vi "HP8753 Collect and Display Data_Modified_V3.vi"(4 "saved data comments":string, 5 "saver's name":string, 6 "saved data title":string, 7 "file name (read description)":path, 8 "error in (no error)":errorcluster, 9 "save to file":bool=TRUE, 10 "data type (6 : formatted data)":u16(ring)=6 items=["raw data array 1", "raw data array 2", "raw data array 3", "raw data array 4", "error-corrected data", "error-corrected trace memory", "formatted data", "formatted memory", "formatted data / memory", "formatted data - memory"], 11 "VISA session":refnum<visa-resource-name>="GPIB0::22::INSTR") -> (0 "error out":errorcluster, 1 "data values":cluster{"real / stim":dbl, "imag / resp":sgl}[](array[cluster])=[{"real / stim"=50000000.0, "imag / resp"=-3.4421387}, {"real / stim"=51531250.0, "imag / resp"=-3.4520264}, {"real / stim"=53062500.0, "imag / resp"=-3.460205}, {"real / stim"=54593750.0, "imag / resp"=-3.465454}, {"real / stim"=56125000.0, "imag / resp"=-3.4788818}, {"real / stim"=57656250.0, "imag / resp"=-3.4852295}, {"real / stim"=59187500.0, "imag / resp"=-3.4934082}, {"real / stim"=60718750.0, "imag / resp"=-3.501587}, {"real / stim"=62250000.0, "imag / resp"=-3.5073242}, {"real / stim"=63781250.0, "imag / resp"=-3.5158691}, {"real / stim"=65312500.0, "imag / resp"=-3.5167236}, {"real / stim"=66843750.0, "imag / resp"=-3.5233154}, {"real / stim"=68375000.0, "imag / resp"=-3.5305176}, {"real / stim"=69906250.0, "imag / resp"=-3.5341797}, {"real / stim"=71437500.0, "imag / resp"=-3.5355225}, {"real / stim"=72968750.0, "imag / resp"=-3.5379639}, {"real / stim"=74500000.0, "imag / resp"=-3.53833}, {"real / stim"=76031250.0, "imag / resp"=-3.5405273}, {"real / stim"=77562500.0, "imag / resp"=-3.539917}, {"real / stim"=79093750.0, "imag / resp"=-3.5395508}, {"real / stim"=80625000.0, "imag / resp"=-3.5390625}, {"real / stim"=82156250.0, "imag / resp"=-3.53833}, {"real / stim"=83687500.0, "imag / resp"=-3.536499}, {"real / stim"=85218750.0, "imag / resp"=-3.5343018}, {"real / stim"=86750000.0, "imag / resp"=-3.53479}, {"real / stim"=88281250.0, "imag / resp"=-3.5333252}, {"real / stim"=89812500.0, "imag / resp"=-3.5310059}, {"real / stim"=91343750.0, "imag / resp"=-3.5339355}, {"real / stim"=92875000.0, "imag / resp"=-3.5319824}, {"real / stim"=94406250.0, "imag / resp"=-3.53479}, {"real / stim"=95937500.0, "imag / resp"=-3.5344238}, {"real / stim"=97468750.0, "imag / resp"=-3.5341797}, {"real / stim"=99000000.0, "imag / resp"=-3.5372314}, {"real / stim"=100531250.0, "imag / resp"=-3.539917}, {"real / stim"=102062500.0, "imag / resp"=-3.5408936}, {"real / stim"=103593750.0, "imag / resp"=-3.5462646}, {"real / stim"=105125000.0, "imag / resp"=-3.548706}, {"real / stim"=106656250.0, "imag / resp"=-3.5534668}, {"real / stim"=108187500.0, "imag / resp"=-3.557495}, {"real / stim"=109718750.0, "imag / resp"=-3.5615234}, {"real / stim"=111250000.0, "imag / resp"=-3.567871}, {"real / stim"=112781250.0, "imag / resp"=-3.5754395}, {"real / stim"=114312500.0, "imag / resp"=-3.578125}, {"real / stim"=115843750.0, "imag / resp"=-3.586792}, {"real / stim"=117375000.0, "imag / resp"=-3.5878906}, {"real / stim"=118906250.0, "imag / resp"=-3.5941162}, {"real / stim"=120437500.0, "imag / resp"=-3.600708}, {"real / stim"=121968750.0, "imag / resp"=-3.6297607}, {"real / stim"=123500000.0, "imag / resp"=-3.6346436}, {"real / stim"=125031250.0, "imag / resp"=-3.637329}, {"real / stim"=126562500.0, "imag / resp"=-3.6402588}, {"real / stim"=128093750.0, "imag / resp"=-3.6430664}, {"real / stim"=129625000.0, "imag / resp"=-3.6451416}, {"real / stim"=131156250.0, "imag / resp"=-3.6461182}, {"real / stim"=132687500.0, "imag / resp"=-3.649414}, {"real / stim"=134218750.0, "imag / resp"=-3.6500244}, {"real / stim"=135750000.0, "imag / resp"=-3.650879}, {"real / stim"=137281250.0, "imag / resp"=-3.649414}, {"real / stim"=138812500.0, "imag / resp"=-3.6502686}, {"real / stim"=140343750.0, "imag / resp"=-3.6501465}, {"real / stim"=141875000.0, "imag / resp"=-3.6499023}, {"real / stim"=143406250.0, "imag / resp"=-3.6488037}, {"real / stim"=144937500.0, "imag / resp"=-3.6505127}, {"real / stim"=146468750.0, "imag / resp"=-3.645874}, {"real / stim"=148000000.0, "imag / resp"=-3.6451416}, {"real / stim"=149531250.0, "imag / resp"=-3.6470947}, {"real / stim"=151062500.0, "imag / resp"=-3.647583}, {"real / stim"=152593750.0, "imag / resp"=-3.647583}, {"real / stim"=154125000.0, "imag / resp"=-3.6468506}, {"real / stim"=155656250.0, "imag / resp"=-3.6461182}, {"real / stim"=157187500.0, "imag / resp"=-3.6483154}, {"real / stim"=158718750.0, "imag / resp"=-3.6479492}, {"real / stim"=160250000.0, "imag / resp"=-3.6478271}, {"real / stim"=161781250.0, "imag / resp"=-3.6495361}, {"real / stim"=163312500.0, "imag / resp"=-3.647461}, {"real / stim"=164843750.0, "imag / resp"=-3.6467285}, {"real / stim"=166375000.0, "imag / resp"=-3.6429443}, {"real / stim"=167906250.0, "imag / resp"=-3.6403809}, {"real / stim"=169437500.0, "imag / resp"=-3.6375732}, {"real / stim"=170968750.0, "imag / resp"=-3.6330566}, {"real / stim"=172500000.0, "imag / resp"=-3.628296}, {"real / stim"=174031250.0, "imag / resp"=-3.6224365}, {"real / stim"=175562500.0, "imag / resp"=-3.6166992}, {"real / stim"=177093750.0, "imag / resp"=-3.6138916}, {"real / stim"=178625000.0, "imag / resp"=-3.605713}, {"real / stim"=180156250.0, "imag / resp"=-3.6018066}, {"real / stim"=181687500.0, "imag / resp"=-3.5952148}, {"real / stim"=183218750.0, "imag / resp"=-3.5897217}, {"real / stim"=184750000.0, "imag / resp"=-3.588501}, {"real / stim"=186281250.0, "imag / resp"=-3.5822754}, {"real / stim"=187812500.0, "imag / resp"=-3.5819092}, {"real / stim"=189343750.0, "imag / resp"=-3.5794678}, {"real / stim"=190875000.0, "imag / resp"=-3.5766602}, {"real / stim"=192406250.0, "imag / resp"=-3.5737305}, {"real / stim"=193937500.0, "imag / resp"=-3.5733643}, {"real / stim"=195468750.0, "imag / resp"=-3.5751953}, {"real / stim"=197000000.0, "imag / resp"=-3.5737305}, {"real / stim"=198531250.0, "imag / resp"=-3.5755615}, {"real / stim"=200062500.0, "imag / resp"=-3.5767822}, {"real / stim"=201593750.0, "imag / resp"=-3.5800781}, {"real / stim"=203125000.0, "imag / resp"=-3.5819092}, {"real / stim"=204656250.0, "imag / resp"=-3.5917969}, {"real / stim"=206187500.0, "imag / resp"=-3.5958252}, {"real / stim"=207718750.0, "imag / resp"=-3.6035156}, {"real / stim"=209250000.0, "imag / resp"=-3.611084}, {"real / stim"=210781250.0, "imag / resp"=-3.6195068}, {"real / stim"=212312500.0, "imag / resp"=-3.6246338}, {"real / stim"=213843750.0, "imag / resp"=-3.6364746}, {"real / stim"=215375000.0, "imag / resp"=-3.6450195}, {"real / stim"=216906250.0, "imag / resp"=-3.6513672}, {"real / stim"=218437500.0, "imag / resp"=-3.6573486}, {"real / stim"=219968750.0, "imag / resp"=-3.664795}, {"real / stim"=221500000.0, "imag / resp"=-3.6678467}, {"real / stim"=223031250.0, "imag / resp"=-3.6729736}, {"real / stim"=224562500.0, "imag / resp"=-3.6712646}, {"real / stim"=226093750.0, "imag / resp"=-3.670288}, {"real / stim"=227625000.0, "imag / resp"=-3.666626}, {"real / stim"=229156250.0, "imag / resp"=-3.6635742}, {"real / stim"=230687500.0, "imag / resp"=-3.657837}, {"real / stim"=232218750.0, "imag / resp"=-3.6553955}, {"real / stim"=233750000.0, "imag / resp"=-3.6481934}, {"real / stim"=235281250.0, "imag / resp"=-3.6396484}, {"real / stim"=236812500.0, "imag / resp"=-3.631836}, {"real / stim"=238343750.0, "imag / resp"=-3.6229248}, {"real / stim"=239875000.0, "imag / resp"=-3.6166992}, {"real / stim"=241406250.0, "imag / resp"=-3.6079102}, {"real / stim"=242937500.0, "imag / resp"=-3.602295}, {"real / stim"=244468750.0, "imag / resp"=-3.5928955}, {"real / stim"=246000000.0, "imag / resp"=-3.5859375}, {"real / stim"=247531250.0, "imag / resp"=-3.579712}, {"real / stim"=249062500.0, "imag / resp"=-3.5720215}, {"real / stim"=250593750.0, "imag / resp"=-3.5701904}, {"real / stim"=252125000.0, "imag / resp"=-3.567871}, {"real / stim"=253656250.0, "imag / resp"=-3.564087}, {"real / stim"=255187500.0, "imag / resp"=-3.5595703}, {"real / stim"=256718750.0, "imag / resp"=-3.5560303}, {"real / stim"=258250000.0, "imag / resp"=-3.5516357}, {"real / stim"=259781250.0, "imag / resp"=-3.5488281}, {"real / stim"=261312500.0, "imag / resp"=-3.5445557}, {"real / stim"=262843750.0, "imag / resp"=-3.545288}, {"real / stim"=264375000.0, "imag / resp"=-3.541626}, {"real / stim"=265906250.0, "imag / resp"=-3.5411377}, {"real / stim"=267437500.0, "imag / resp"=-3.5386963}, {"real / stim"=268968750.0, "imag / resp"=-3.5327148}, {"real / stim"=270500000.0, "imag / resp"=-3.529541}, {"real / stim"=272031250.0, "imag / resp"=-3.5256348}, {"real / stim"=273562500.0, "imag / resp"=-3.5212402}, {"real / stim"=275093750.0, "imag / resp"=-3.5153809}, {"real / stim"=276625000.0, "imag / resp"=-3.5135498}, {"real / stim"=278156250.0, "imag / resp"=-3.5101318}, {"real / stim"=279687500.0, "imag / resp"=-3.5045166}, {"real / stim"=281218750.0, "imag / resp"=-3.50354}, {"real / stim"=282750000.0, "imag / resp"=-3.5014648}, {"real / stim"=284281250.0, "imag / resp"=-3.4952393}, {"real / stim"=285812500.0, "imag / resp"=-3.4960938}, {"real / stim"=287343750.0, "imag / resp"=-3.4942627}, {"real / stim"=288875000.0, "imag / resp"=-3.4920654}, {"real / stim"=290406250.0, "imag / resp"=-3.4903564}, {"real / stim"=291937500.0, "imag / resp"=-3.4906006}, {"real / stim"=293468750.0, "imag / resp"=-3.493042}, {"real / stim"=295000000.0, "imag / resp"=-3.4952393}, {"real / stim"=296531250.0, "imag / resp"=-3.496582}, {"real / stim"=298062500.0, "imag / resp"=-3.5}, {"real / stim"=299593750.0, "imag / resp"=-3.5042725}, {"real / stim"=301125000.0, "imag / resp"=-3.5093994}, {"real / stim"=302656250.0, "imag / resp"=-3.515503}, {"real / stim"=304187500.0, "imag / resp"=-3.5222168}, {"real / stim"=305718750.0, "imag / resp"=-3.5230713}, {"real / stim"=307250000.0, "imag / resp"=-3.5317383}, {"real / stim"=308781250.0, "imag / resp"=-3.5350342}, {"real / stim"=310312500.0, "imag / resp"=-3.5384521}, {"real / stim"=311843750.0, "imag / resp"=-3.5410156}, {"real / stim"=313375000.0, "imag / resp"=-3.5408936}, {"real / stim"=314906250.0, "imag / resp"=-3.5386963}, {"real / stim"=316437500.0, "imag / resp"=-3.536499}, {"real / stim"=317968750.0, "imag / resp"=-3.5317383}, {"real / stim"=319500000.0, "imag / resp"=-3.5231934}, {"real / stim"=321031250.0, "imag / resp"=-3.5150146}, {"real / stim"=322562500.0, "imag / resp"=-3.5029297}, {"real / stim"=324093750.0, "imag / resp"=-3.4937744}, {"real / stim"=325625000.0, "imag / resp"=-3.4818115}, {"real / stim"=327156250.0, "imag / resp"=-3.4685059}, {"real / stim"=328687500.0, "imag / resp"=-3.4542236}, {"real / stim"=330218750.0, "imag / resp"=-3.4396973}, {"real / stim"=331750000.0, "imag / resp"=-3.4239502}, {"real / stim"=333281250.0, "imag / resp"=-3.4139404}, {"real / stim"=334812500.0, "imag / resp"=-3.3981934}, {"real / stim"=336343750.0, "imag / resp"=-3.3891602}, {"real / stim"=337875000.0, "imag / resp"=-3.3780518}, {"real / stim"=339406250.0, "imag / resp"=-3.3676758}, {"real / stim"=340937500.0, "imag / resp"=-3.359253}, {"real / stim"=342468750.0, "imag / resp"=-3.348877}, {"real / stim"=344000000.0, "imag / resp"=-3.3426514}, {"real / stim"=345531250.0, "imag / resp"=-3.3361816}, {"real / stim"=347062500.0, "imag / resp"=-3.3267822}, {"real / stim"=348593750.0, "imag / resp"=-3.3200684}, {"real / stim"=350125000.0, "imag / resp"=-3.314209}, {"real / stim"=351656250.0, "imag / resp"=-3.3060303}, {"real / stim"=353187500.0, "imag / resp"=-3.2999268}, {"real / stim"=354718750.0, "imag / resp"=-3.2924805}, {"real / stim"=356250000.0, "imag / resp"=-3.2878418}, {"real / stim"=357781250.0, "imag / resp"=-3.2827148}, {"real / stim"=359312500.0, "imag / resp"=-3.2756348}, {"real / stim"=360843750.0, "imag / resp"=-3.268921}, {"real / stim"=362375000.0, "imag / resp"=-3.265747}, {"real / stim"=363906250.0, "imag / resp"=-3.2613525}, {"real / stim"=365437500.0, "imag / resp"=-3.2561035}, {"real / stim"=366968750.0, "imag / resp"=-3.248291}, {"real / stim"=368500000.0, "imag / resp"=-3.2403564}, {"real / stim"=370031250.0, "imag / resp"=-3.2387695}, {"real / stim"=371562500.0, "imag / resp"=-3.232544}, {"real / stim"=373093750.0, "imag / resp"=-3.2229004}, {"real / stim"=374625000.0, "imag / resp"=-3.2219238}, {"real / stim"=376156250.0, "imag / resp"=-3.213379}, {"real / stim"=377687500.0, "imag / resp"=-3.2088623}, {"real / stim"=379218750.0, "imag / resp"=-3.2069092}, {"real / stim"=380750000.0, "imag / resp"=-3.2022705}, {"real / stim"=382281250.0, "imag / resp"=-3.197998}, {"real / stim"=383812500.0, "imag / resp"=-3.1929932}, {"real / stim"=385343750.0, "imag / resp"=-3.1867676}, {"real / stim"=386875000.0, "imag / resp"=-3.1846924}, {"real / stim"=388406250.0, "imag / resp"=-3.182251}, {"real / stim"=389937500.0, "imag / resp"=-3.1723633}, {"real / stim"=391468750.0, "imag / resp"=-3.1693115}, {"real / stim"=393000000.0, "imag / resp"=-3.1618652}, {"real / stim"=394531250.0, "imag / resp"=-3.1582031}, {"real / stim"=396062500.0, "imag / resp"=-3.151123}, {"real / stim"=397593750.0, "imag / resp"=-3.1497803}, {"real / stim"=399125000.0, "imag / resp"=-3.1468506}, {"real / stim"=400656250.0, "imag / resp"=-3.142334}, {"real / stim"=402187500.0, "imag / resp"=-3.1401367}, {"real / stim"=403718750.0, "imag / resp"=-3.1350098}, {"real / stim"=405250000.0, "imag / resp"=-3.1322021}, {"real / stim"=406781250.0, "imag / resp"=-3.1287842}, {"real / stim"=408312500.0, "imag / resp"=-3.1269531}, {"real / stim"=409843750.0, "imag / resp"=-3.1207275}, {"real / stim"=411375000.0, "imag / resp"=-3.1124268}, {"real / stim"=412906250.0, "imag / resp"=-3.109253}, {"real / stim"=414437500.0, "imag / resp"=-3.1004639}, {"real / stim"=415968750.0, "imag / resp"=-3.0942383}, {"real / stim"=417500000.0, "imag / resp"=-3.086792}, {"real / stim"=419031250.0, "imag / resp"=-3.0787354}, {"real / stim"=420562500.0, "imag / resp"=-3.071289}, {"real / stim"=422093750.0, "imag / resp"=-3.0628662}, {"real / stim"=423625000.0, "imag / resp"=-3.060913}, {"real / stim"=425156250.0, "imag / resp"=-3.0493164}, {"real / stim"=426687500.0, "imag / resp"=-3.0463867}, {"real / stim"=428218750.0, "imag / resp"=-3.0390625}, {"real / stim"=429750000.0, "imag / resp"=-3.0340576}, {"real / stim"=431281250.0, "imag / resp"=-3.0281982}, {"real / stim"=432812500.0, "imag / resp"=-3.020752}, {"real / stim"=434343750.0, "imag / resp"=-3.0109863}, {"real / stim"=435875000.0, "imag / resp"=-3.0072021}, {"real / stim"=437406250.0, "imag / resp"=-3.0039062}, {"real / stim"=438937500.0, "imag / resp"=-2.9969482}, {"real / stim"=440468750.0, "imag / resp"=-2.994873}, {"real / stim"=442000000.0, "imag / resp"=-2.9940186}, {"real / stim"=443531250.0, "imag / resp"=-2.9868164}, {"real / stim"=445062500.0, "imag / resp"=-2.9829102}, {"real / stim"=446593750.0, "imag / resp"=-2.9801025}, {"real / stim"=448125000.0, "imag / resp"=-2.9782715}, {"real / stim"=449656250.0, "imag / resp"=-2.979248}, {"real / stim"=451187500.0, "imag / resp"=-2.9776611}, {"real / stim"=452718750.0, "imag / resp"=-2.9768066}, {"real / stim"=454250000.0, "imag / resp"=-2.97583}, {"real / stim"=455781250.0, "imag / resp"=-2.975586}, {"real / stim"=457312500.0, "imag / resp"=-2.9731445}, {"real / stim"=458843750.0, "imag / resp"=-2.9672852}, {"real / stim"=460375000.0, "imag / resp"=-2.963379}, {"real / stim"=461906250.0, "imag / resp"=-2.9614258}, {"real / stim"=463437500.0, "imag / resp"=-2.9541016}, {"real / stim"=464968750.0, "imag / resp"=-2.947998}, {"real / stim"=466500000.0, "imag / resp"=-2.939087}, {"real / stim"=468031250.0, "imag / resp"=-2.930664}, {"real / stim"=469562500.0, "imag / resp"=-2.9232178}, {"real / stim"=471093750.0, "imag / resp"=-2.9160156}, {"real / stim"=472625000.0, "imag / resp"=-2.9084473}, {"real / stim"=474156250.0, "imag / resp"=-2.8984375}, {"real / stim"=475687500.0, "imag / resp"=-2.8894043}, {"real / stim"=477218750.0, "imag / resp"=-2.8780518}, {"real / stim"=478750000.0, "imag / resp"=-2.87146}, {"real / stim"=480281250.0, "imag / resp"=-2.862915}, {"real / stim"=481812500.0, "imag / resp"=-2.8583984}, {"real / stim"=483343750.0, "imag / resp"=-2.8497314}, {"real / stim"=484875000.0, "imag / resp"=-2.8443604}, {"real / stim"=486406250.0, "imag / resp"=-2.8378906}, {"real / stim"=487937500.0, "imag / resp"=-2.833496}, {"real / stim"=489468750.0, "imag / resp"=-2.8250732}, {"real / stim"=491000000.0, "imag / resp"=-2.826416}, {"real / stim"=492531250.0, "imag / resp"=-2.8209229}, {"real / stim"=494062500.0, "imag / resp"=-2.8170166}, {"real / stim"=495593750.0, "imag / resp"=-2.8131104}, {"real / stim"=497125000.0, "imag / resp"=-2.8127441}, {"real / stim"=498656250.0, "imag / resp"=-2.8111572}, {"real / stim"=500187500.0, "imag / resp"=-2.8095703}, {"real / stim"=501718750.0, "imag / resp"=-2.8087158}, {"real / stim"=503250000.0, "imag / resp"=-2.8051758}, {"real / stim"=504781250.0, "imag / resp"=-2.800415}, {"real / stim"=506312500.0, "imag / resp"=-2.7983398}, {"real / stim"=507843750.0, "imag / resp"=-2.800537}, {"real / stim"=509375000.0, "imag / resp"=-2.7972412}, {"real / stim"=510906250.0, "imag / resp"=-2.7955322}, {"real / stim"=512437500.0, "imag / resp"=-2.7893066}, {"real / stim"=513968750.0, "imag / resp"=-2.789795}, {"real / stim"=515500000.0, "imag / resp"=-2.7834473}, {"real / stim"=517031250.0, "imag / resp"=-2.779541}, {"real / stim"=518562500.0, "imag / resp"=-2.7781982}, {"real / stim"=520093750.0, "imag / resp"=-2.775879}, {"real / stim"=521625000.0, "imag / resp"=-2.7729492}, {"real / stim"=523156250.0, "imag / resp"=-2.770874}, {"real / stim"=524687500.0, "imag / resp"=-2.7645264}, {"real / stim"=526218750.0, "imag / resp"=-2.7635498}, {"real / stim"=527750000.0, "imag / resp"=-2.7574463}, {"real / stim"=529281250.0, "imag / resp"=-2.7558594}, {"real / stim"=530812500.0, "imag / resp"=-2.7543945}, {"real / stim"=532343750.0, "imag / resp"=-2.7503662}, {"real / stim"=533875000.0, "imag / resp"=-2.7474365}, {"real / stim"=535406250.0, "imag / resp"=-2.7425537}, {"real / stim"=536937500.0, "imag / resp"=-2.7371826}, {"real / stim"=538468750.0, "imag / resp"=-2.7368164}, {"real / stim"=540000000.0, "imag / resp"=-2.7336426}, {"real / stim"=541531250.0, "imag / resp"=-2.7313232}, {"real / stim"=543062500.0, "imag / resp"=-2.72937}, {"real / stim"=544593750.0, "imag / resp"=-2.7286377}, {"real / stim"=546125000.0, "imag / resp"=-2.7264404}, {"real / stim"=547656250.0, "imag / resp"=-2.7231445}, {"real / stim"=549187500.0, "imag / resp"=-2.7215576}, {"real / stim"=550718750.0, "imag / resp"=-2.71875}, {"real / stim"=552250000.0, "imag / resp"=-2.7202148}, {"real / stim"=553781250.0, "imag / resp"=-2.7163086}, {"real / stim"=555312500.0, "imag / resp"=-2.7155762}, {"real / stim"=556843750.0, "imag / resp"=-2.7121582}, {"real / stim"=558375000.0, "imag / resp"=-2.709961}, {"real / stim"=559906250.0, "imag / resp"=-2.709961}, {"real / stim"=561437500.0, "imag / resp"=-2.7073975}, {"real / stim"=562968750.0, "imag / resp"=-2.7020264}, {"real / stim"=564500000.0, "imag / resp"=-2.701416}, {"real / stim"=566031250.0, "imag / resp"=-2.6993408}, {"real / stim"=567562500.0, "imag / resp"=-2.6949463}, {"real / stim"=569093750.0, "imag / resp"=-2.6939697}, {"real / stim"=570625000.0, "imag / resp"=-2.6903076}, {"real / stim"=572156250.0, "imag / resp"=-2.6895752}, {"real / stim"=573687500.0, "imag / resp"=-2.6875}, {"real / stim"=575218750.0, "imag / resp"=-2.684082}, {"real / stim"=576750000.0, "imag / resp"=-2.6843262}, {"real / stim"=578281250.0, "imag / resp"=-2.6846924}, {"real / stim"=579812500.0, "imag / resp"=-2.6829834}, {"real / stim"=581343750.0, "imag / resp"=-2.6826172}, {"real / stim"=582875000.0, "imag / resp"=-2.6817627}, {"real / stim"=584406250.0, "imag / resp"=-2.684082}, {"real / stim"=585937500.0, "imag / resp"=-2.6811523}, {"real / stim"=587468750.0, "imag / resp"=-2.683838}, {"real / stim"=589000000.0, "imag / resp"=-2.685669}, {"real / stim"=590531250.0, "imag / resp"=-2.6853027}, {"real / stim"=592062500.0, "imag / resp"=-2.6868896}, {"real / stim"=593593750.0, "imag / resp"=-2.6906738}, {"real / stim"=595125000.0, "imag / resp"=-2.6914062}, {"real / stim"=596656250.0, "imag / resp"=-2.6934814}, {"real / stim"=598187500.0, "imag / resp"=-2.6942139}, {"real / stim"=599718750.0, "imag / resp"=-2.6964111}, {"real / stim"=601250000.0, "imag / resp"=-2.7023926}, {"real / stim"=602781250.0, "imag / resp"=-2.7038574}, {"real / stim"=604312500.0, "imag / resp"=-2.7019043}, {"real / stim"=605843750.0, "imag / resp"=-2.7053223}, {"real / stim"=607375000.0, "imag / resp"=-2.7088623}, {"real / stim"=608906250.0, "imag / resp"=-2.7130127}, {"real / stim"=610437500.0, "imag / resp"=-2.713501}, {"real / stim"=611968750.0, "imag / resp"=-2.7181396}, {"real / stim"=613500000.0, "imag / resp"=-2.7231445}, {"real / stim"=615031250.0, "imag / resp"=-2.7226562}, {"real / stim"=616562500.0, "imag / resp"=-2.7263184}, {"real / stim"=618093750.0, "imag / resp"=-2.7285156}, {"real / stim"=619625000.0, "imag / resp"=-2.7320557}, {"real / stim"=621156250.0, "imag / resp"=-2.732788}, {"real / stim"=622687500.0, "imag / resp"=-2.7375488}, {"real / stim"=624218750.0, "imag / resp"=-2.7432861}, {"real / stim"=625750000.0, "imag / resp"=-2.7454834}, {"real / stim"=627281250.0, "imag / resp"=-2.7487793}, {"real / stim"=628812500.0, "imag / resp"=-2.7545166}, {"real / stim"=630343750.0, "imag / resp"=-2.7589111}, {"real / stim"=631875000.0, "imag / resp"=-2.7633057}, {"real / stim"=633406250.0, "imag / resp"=-2.7698975}, {"real / stim"=634937500.0, "imag / resp"=-2.7734375}, {"real / stim"=636468750.0, "imag / resp"=-2.7840576}, {"real / stim"=638000000.0, "imag / resp"=-2.7890625}, {"real / stim"=639531250.0, "imag / resp"=-2.7982178}, {"real / stim"=641062500.0, "imag / resp"=-2.8051758}, {"real / stim"=642593750.0, "imag / resp"=-2.8135986}, {"real / stim"=644125000.0, "imag / resp"=-2.819336}, {"real / stim"=645656250.0, "imag / resp"=-2.8310547}, {"real / stim"=647187500.0, "imag / resp"=-2.8365479}, {"real / stim"=648718750.0, "imag / resp"=-2.850586}, {"real / stim"=650250000.0, "imag / resp"=-2.857544}, {"real / stim"=651781250.0, "imag / resp"=-2.866211}, {"real / stim"=653312500.0, "imag / resp"=-2.8760986}, {"real / stim"=654843750.0, "imag / resp"=-2.8884277}, {"real / stim"=656375000.0, "imag / resp"=-2.900879}, {"real / stim"=657906250.0, "imag / resp"=-2.9106445}, {"real / stim"=659437500.0, "imag / resp"=-2.9228516}, {"real / stim"=660968750.0, "imag / resp"=-2.9395752}, {"real / stim"=662500000.0, "imag / resp"=-2.951416}, {"real / stim"=664031250.0, "imag / resp"=-2.9677734}, {"real / stim"=665562500.0, "imag / resp"=-2.9816895}, {"real / stim"=667093750.0, "imag / resp"=-2.9985352}, {"real / stim"=668625000.0, "imag / resp"=-3.0142822}, {"real / stim"=670156250.0, "imag / resp"=-3.0336914}, {"real / stim"=671687500.0, "imag / resp"=-3.0532227}, {"real / stim"=673218750.0, "imag / resp"=-3.0703125}, {"real / stim"=674750000.0, "imag / resp"=-3.0942383}, {"real / stim"=676281250.0, "imag / resp"=-3.1136475}, {"real / stim"=677812500.0, "imag / resp"=-3.1384277}, {"real / stim"=679343750.0, "imag / resp"=-3.1657715}, {"real / stim"=680875000.0, "imag / resp"=-3.1912842}, {"real / stim"=682406250.0, "imag / resp"=-3.2218018}, {"real / stim"=683937500.0, "imag / resp"=-3.2485352}, {"real / stim"=685468750.0, "imag / resp"=-3.2784424}, {"real / stim"=687000000.0, "imag / resp"=-3.3138428}, {"real / stim"=688531250.0, "imag / resp"=-3.345337}, {"real / stim"=690062500.0, "imag / resp"=-3.3814697}, {"real / stim"=691593750.0, "imag / resp"=-3.418457}, {"real / stim"=693125000.0, "imag / resp"=-3.4538574}, {"real / stim"=694656250.0, "imag / resp"=-3.4940186}, {"real / stim"=696187500.0, "imag / resp"=-3.5374756}, {"real / stim"=697718750.0, "imag / resp"=-3.579834}, {"real / stim"=699250000.0, "imag / resp"=-3.619751}, {"real / stim"=700781250.0, "imag / resp"=-3.665039}, {"real / stim"=702312500.0, "imag / resp"=-3.7087402}, {"real / stim"=703843750.0, "imag / resp"=-3.7529297}, {"real / stim"=705375000.0, "imag / resp"=-3.796875}, {"real / stim"=706906250.0, "imag / resp"=-3.843872}, {"real / stim"=708437500.0, "imag / resp"=-3.8878174}, {"real / stim"=709968750.0, "imag / resp"=-3.928711}, {"real / stim"=711500000.0, "imag / resp"=-3.9735107}, {"real / stim"=713031250.0, "imag / resp"=-4.0117188}, {"real / stim"=714562500.0, "imag / resp"=-4.0495605}, {"real / stim"=716093750.0, "imag / resp"=-4.08667}, {"real / stim"=717625000.0, "imag / resp"=-4.1210938}, {"real / stim"=719156250.0, "imag / resp"=-4.150879}, {"real / stim"=720687500.0, "imag / resp"=-4.178955}, {"real / stim"=722218750.0, "imag / resp"=-4.2009277}, {"real / stim"=723750000.0, "imag / resp"=-4.220459}, {"real / stim"=725281250.0, "imag / resp"=-4.2370605}, {"real / stim"=726812500.0, "imag / resp"=-4.2470703}, {"real / stim"=728343750.0, "imag / resp"=-4.2509766}, {"real / stim"=729875000.0, "imag / resp"=-4.253174}, {"real / stim"=731406250.0, "imag / resp"=-4.2487793}, {"real / stim"=732937500.0, "imag / resp"=-4.238037}, {"real / stim"=734468750.0, "imag / resp"=-4.2250977}, {"real / stim"=736000000.0, "imag / resp"=-4.2106934}, {"real / stim"=737531250.0, "imag / resp"=-4.1884766}, {"real / stim"=739062500.0, "imag / resp"=-4.166748}, {"real / stim"=740593750.0, "imag / resp"=-4.147461}, {"real / stim"=742125000.0, "imag / resp"=-4.116455}, {"real / stim"=743656250.0, "imag / resp"=-4.0915527}, {"real / stim"=745187500.0, "imag / resp"=-4.065918}, {"real / stim"=746718750.0, "imag / resp"=-4.033203}, {"real / stim"=748250000.0, "imag / resp"=-4.0080566}, {"real / stim"=749781250.0, "imag / resp"=-3.9819336}, {"real / stim"=751312500.0, "imag / resp"=-3.9525146}, {"real / stim"=752843750.0, "imag / resp"=-3.9273682}, {"real / stim"=754375000.0, "imag / resp"=-3.9002686}, {"real / stim"=755906250.0, "imag / resp"=-3.8754883}, {"real / stim"=757437500.0, "imag / resp"=-3.8496094}, {"real / stim"=758968750.0, "imag / resp"=-3.8243408}, {"real / stim"=760500000.0, "imag / resp"=-3.8017578}, {"real / stim"=762031250.0, "imag / resp"=-3.7774658}, {"real / stim"=763562500.0, "imag / resp"=-3.7528076}, {"real / stim"=765093750.0, "imag / resp"=-3.7271729}, {"real / stim"=766625000.0, "imag / resp"=-3.7041016}, {"real / stim"=768156250.0, "imag / resp"=-3.6816406}, {"real / stim"=769687500.0, "imag / resp"=-3.659546}, {"real / stim"=771218750.0, "imag / resp"=-3.6368408}, {"real / stim"=772750000.0, "imag / resp"=-3.6119385}, {"real / stim"=774281250.0, "imag / resp"=-3.5906982}, {"real / stim"=775812500.0, "imag / resp"=-3.5682373}, {"real / stim"=777343750.0, "imag / resp"=-3.546997}, {"real / stim"=778875000.0, "imag / resp"=-3.5256348}, {"real / stim"=780406250.0, "imag / resp"=-3.5039062}, {"real / stim"=781937500.0, "imag / resp"=-3.4840088}, {"real / stim"=783468750.0, "imag / resp"=-3.4656982}, {"real / stim"=785000000.0, "imag / resp"=-3.4483643}, {"real / stim"=786531250.0, "imag / resp"=-3.432129}, {"real / stim"=788062500.0, "imag / resp"=-3.4139404}, {"real / stim"=789593750.0, "imag / resp"=-3.4006348}, {"real / stim"=791125000.0, "imag / resp"=-3.3862305}, {"real / stim"=792656250.0, "imag / resp"=-3.374878}, {"real / stim"=794187500.0, "imag / resp"=-3.362671}, {"real / stim"=795718750.0, "imag / resp"=-3.3515625}, {"real / stim"=797250000.0, "imag / resp"=-3.3410645}, {"real / stim"=798781250.0, "imag / resp"=-3.3305664}, {"real / stim"=800312500.0, "imag / resp"=-3.3204346}, {"real / stim"=801843750.0, "imag / resp"=-3.3148193}, {"real / stim"=803375000.0, "imag / resp"=-3.307495}, {"real / stim"=804906250.0, "imag / resp"=-3.3006592}, {"real / stim"=806437500.0, "imag / resp"=-3.293335}, {"real / stim"=807968750.0, "imag / resp"=-3.286499}, {"real / stim"=809500000.0, "imag / resp"=-3.2797852}, {"real / stim"=811031250.0, "imag / resp"=-3.2736816}, {"real / stim"=812562500.0, "imag / resp"=-3.2696533}, {"real / stim"=814093750.0, "imag / resp"=-3.2633057}, {"real / stim"=815625000.0, "imag / resp"=-3.255005}, {"real / stim"=817156250.0, "imag / resp"=-3.2507324}, {"real / stim"=818687500.0, "imag / resp"=-3.248291}, {"real / stim"=820218750.0, "imag / resp"=-3.241211}, {"real / stim"=821750000.0, "imag / resp"=-3.2398682}, {"real / stim"=823281250.0, "imag / resp"=-3.2357178}, {"real / stim"=824812500.0, "imag / resp"=-3.2305908}, {"real / stim"=826343750.0, "imag / resp"=-3.225708}, {"real / stim"=827875000.0, "imag / resp"=-3.2196045}, {"real / stim"=829406250.0, "imag / resp"=-3.2180176}, {"real / stim"=830937500.0, "imag / resp"=-3.2143555}, {"real / stim"=832468750.0, "imag / resp"=-3.208252}, {"real / stim"=834000000.0, "imag / resp"=-3.2075195}, {"real / stim"=835531250.0, "imag / resp"=-3.2010498}, {"real / stim"=837062500.0, "imag / resp"=-3.1973877}, {"real / stim"=838593750.0, "imag / resp"=-3.1965332}, {"real / stim"=840125000.0, "imag / resp"=-3.1904297}, {"real / stim"=841656250.0, "imag / resp"=-3.1870117}, {"real / stim"=843187500.0, "imag / resp"=-3.1846924}, {"real / stim"=844718750.0, "imag / resp"=-3.1813965}, {"real / stim"=846250000.0, "imag / resp"=-3.177246}, {"real / stim"=847781250.0, "imag / resp"=-3.1762695}, {"real / stim"=849312500.0, "imag / resp"=-3.1711426}, {"real / stim"=850843750.0, "imag / resp"=-3.1711426}, {"real / stim"=852375000.0, "imag / resp"=-3.168213}, {"real / stim"=853906250.0, "imag / resp"=-3.1643066}, {"real / stim"=855437500.0, "imag / resp"=-3.1606445}, {"real / stim"=856968750.0, "imag / resp"=-3.1583252}, {"real / stim"=858500000.0, "imag / resp"=-3.1530762}, {"real / stim"=860031250.0, "imag / resp"=-3.1481934}, {"real / stim"=861562500.0, "imag / resp"=-3.1428223}, {"real / stim"=863093750.0, "imag / resp"=-3.1376953}, {"real / stim"=864625000.0, "imag / resp"=-3.1367188}, {"real / stim"=866156250.0, "imag / resp"=-3.1328125}, {"real / stim"=867687500.0, "imag / resp"=-3.1315918}, {"real / stim"=869218750.0, "imag / resp"=-3.1312256}, {"real / stim"=870750000.0, "imag / resp"=-3.1274414}, {"real / stim"=872281250.0, "imag / resp"=-3.1226807}, {"real / stim"=873812500.0, "imag / resp"=-3.1237793}, {"real / stim"=875343750.0, "imag / resp"=-3.1235352}, {"real / stim"=876875000.0, "imag / resp"=-3.1228027}, {"real / stim"=878406250.0, "imag / resp"=-3.1208496}, {"real / stim"=879937500.0, "imag / resp"=-3.1206055}, {"real / stim"=881468750.0, "imag / resp"=-3.1218262}, {"real / stim"=883000000.0, "imag / resp"=-3.1241455}, {"real / stim"=884531250.0, "imag / resp"=-3.1257324}, {"real / stim"=886062500.0, "imag / resp"=-3.1291504}, {"real / stim"=887593750.0, "imag / resp"=-3.126709}, {"real / stim"=889125000.0, "imag / resp"=-3.1326904}, {"real / stim"=890656250.0, "imag / resp"=-3.1345215}, {"real / stim"=892187500.0, "imag / resp"=-3.1363525}, {"real / stim"=893718750.0, "imag / resp"=-3.142456}, {"real / stim"=895250000.0, "imag / resp"=-3.143921}, {"real / stim"=896781250.0, "imag / resp"=-3.1467285}, {"real / stim"=898312500.0, "imag / resp"=-3.151123}, {"real / stim"=899843750.0, "imag / resp"=-3.154419}, {"real / stim"=901375000.0, "imag / resp"=-3.1571045}, {"real / stim"=902906250.0, "imag / resp"=-3.1629639}, {"real / stim"=904437500.0, "imag / resp"=-3.1638184}, {"real / stim"=905968750.0, "imag / resp"=-3.168457}, {"real / stim"=907500000.0, "imag / resp"=-3.1716309}, {"real / stim"=909031250.0, "imag / resp"=-3.1750488}, {"real / stim"=910562500.0, "imag / resp"=-3.1816406}, {"real / stim"=912093750.0, "imag / resp"=-3.1827393}, {"real / stim"=913625000.0, "imag / resp"=-3.1862793}, {"real / stim"=915156250.0, "imag / resp"=-3.1881104}, {"real / stim"=916687500.0, "imag / resp"=-3.1901855}, {"real / stim"=918218750.0, "imag / resp"=-3.1948242}, {"real / stim"=919750000.0, "imag / resp"=-3.1934814}, {"real / stim"=921281250.0, "imag / resp"=-3.1986084}, {"real / stim"=922812500.0, "imag / resp"=-3.199829}, {"real / stim"=924343750.0, "imag / resp"=-3.2038574}, {"real / stim"=925875000.0, "imag / resp"=-3.2055664}, {"real / stim"=927406250.0, "imag / resp"=-3.206665}, {"real / stim"=928937500.0, "imag / resp"=-3.2087402}, {"real / stim"=930468750.0, "imag / resp"=-3.2126465}, {"real / stim"=932000000.0, "imag / resp"=-3.2144775}, {"real / stim"=933531250.0, "imag / resp"=-3.211792}, {"real / stim"=935062500.0, "imag / resp"=-3.2163086}, {"real / stim"=936593750.0, "imag / resp"=-3.2172852}, {"real / stim"=938125000.0, "imag / resp"=-3.2183838}, {"real / stim"=939656250.0, "imag / resp"=-3.2194824}, {"real / stim"=941187500.0, "imag / resp"=-3.2210693}, {"real / stim"=942718750.0, "imag / resp"=-3.2216797}, {"real / stim"=944250000.0, "imag / resp"=-3.2247314}, {"real / stim"=945781250.0, "imag / resp"=-3.2253418}, {"real / stim"=947312500.0, "imag / resp"=-3.2283936}, {"real / stim"=948843750.0, "imag / resp"=-3.2266846}, {"real / stim"=950375000.0, "imag / resp"=-3.2281494}, {"real / stim"=951906250.0, "imag / resp"=-3.227295}, {"real / stim"=953437500.0, "imag / resp"=-3.2299805}, {"real / stim"=954968750.0, "imag / resp"=-3.2301025}, {"real / stim"=956500000.0, "imag / resp"=-3.2319336}, {"real / stim"=958031250.0, "imag / resp"=-3.231079}, {"real / stim"=959562500.0, "imag / resp"=-3.229248}, {"real / stim"=961093750.0, "imag / resp"=-3.235962}, {"real / stim"=962625000.0, "imag / resp"=-3.2352295}, {"real / stim"=964156250.0, "imag / resp"=-3.2340088}, {"real / stim"=965687500.0, "imag / resp"=-3.2347412}, {"real / stim"=967218750.0, "imag / resp"=-3.237793}, {"real / stim"=968750000.0, "imag / resp"=-3.2388916}, {"real / stim"=970281250.0, "imag / resp"=-3.2403564}, {"real / stim"=971812500.0, "imag / resp"=-3.241455}, {"real / stim"=973343750.0, "imag / resp"=-3.2427979}, {"real / stim"=974875000.0, "imag / resp"=-3.2443848}, {"real / stim"=976406250.0, "imag / resp"=-3.244995}, {"real / stim"=977937500.0, "imag / resp"=-3.2458496}, {"real / stim"=979468750.0, "imag / resp"=-3.249878}, {"real / stim"=981000000.0, "imag / resp"=-3.2520752}, {"real / stim"=982531250.0, "imag / resp"=-3.2528076}, {"real / stim"=984062500.0, "imag / resp"=-3.2559814}, {"real / stim"=985593750.0, "imag / resp"=-3.26062}, {"real / stim"=987125000.0, "imag / resp"=-3.2652588}, {"real / stim"=988656250.0, "imag / resp"=-3.2664795}, {"real / stim"=990187500.0, "imag / resp"=-3.2722168}, {"real / stim"=991718750.0, "imag / resp"=-3.2752686}, {"real / stim"=993250000.0, "imag / resp"=-3.2823486}, {"real / stim"=994781250.0, "imag / resp"=-3.2877197}, {"real / stim"=996312500.0, "imag / resp"=-3.2929688}, {"real / stim"=997843750.0, "imag / resp"=-3.2956543}, {"real / stim"=999375000.0, "imag / resp"=-3.2980957}, {"real / stim"=1000906250.0, "imag / resp"=-3.30542}, {"real / stim"=1002437500.0, "imag / resp"=-3.3076172}, {"real / stim"=1003968750.0, "imag / resp"=-3.3115234}, {"real / stim"=1005500000.0, "imag / resp"=-3.3162842}, {"real / stim"=1007031250.0, "imag / resp"=-3.3223877}, {"real / stim"=1008562500.0, "imag / resp"=-3.326416}, {"real / stim"=1010093750.0, "imag / resp"=-3.3325195}, {"real / stim"=1011625000.0, "imag / resp"=-3.3370361}, {"real / stim"=1013156250.0, "imag / resp"=-3.3406982}, {"real / stim"=1014687500.0, "imag / resp"=-3.3479004}, {"real / stim"=1016218750.0, "imag / resp"=-3.3535156}, {"real / stim"=1017750000.0, "imag / resp"=-3.359253}, {"real / stim"=1019281250.0, "imag / resp"=-3.3649902}, {"real / stim"=1020812500.0, "imag / resp"=-3.3685303}, {"real / stim"=1022343750.0, "imag / resp"=-3.3742676}, {"real / stim"=1023875000.0, "imag / resp"=-3.3774414}, {"real / stim"=1025406250.0, "imag / resp"=-3.3811035}, {"real / stim"=1026937500.0, "imag / resp"=-3.388794}, {"real / stim"=1028468750.0, "imag / resp"=-3.3950195}, {"real / stim"=1030000000.0, "imag / resp"=-3.3966064}, {"real / stim"=1031531250.0, "imag / resp"=-3.401123}, {"real / stim"=1033062500.0, "imag / resp"=-3.4075928}, {"real / stim"=1034593750.0, "imag / resp"=-3.413086}, {"real / stim"=1036125000.0, "imag / resp"=-3.420044}, {"real / stim"=1037656250.0, "imag / resp"=-3.4213867}, {"real / stim"=1039187500.0, "imag / resp"=-3.4277344}, {"real / stim"=1040718750.0, "imag / resp"=-3.4311523}, {"real / stim"=1042250000.0, "imag / resp"=-3.434204}, {"real / stim"=1043781250.0, "imag / resp"=-3.4375}, {"real / stim"=1045312500.0, "imag / resp"=-3.4422607}, {"real / stim"=1046843750.0, "imag / resp"=-3.4468994}, {"real / stim"=1048375000.0, "imag / resp"=-3.4510498}, {"real / stim"=1049906250.0, "imag / resp"=-3.454956}, {"real / stim"=1051437500.0, "imag / resp"=-3.4575195}, {"real / stim"=1052968750.0, "imag / resp"=-3.46167}, {"real / stim"=1054500000.0, "imag / resp"=-3.4609375}, {"real / stim"=1056031250.0, "imag / resp"=-3.465088}, {"real / stim"=1057562500.0, "imag / resp"=-3.4649658}, {"real / stim"=1059093750.0, "imag / resp"=-3.468872}, {"real / stim"=1060625000.0, "imag / resp"=-3.472168}, {"real / stim"=1062156250.0, "imag / resp"=-3.4746094}, {"real / stim"=1063687500.0, "imag / resp"=-3.4770508}, {"real / stim"=1065218750.0, "imag / resp"=-3.473755}, {"real / stim"=1066750000.0, "imag / resp"=-3.4766846}, {"real / stim"=1068281250.0, "imag / resp"=-3.4798584}, {"real / stim"=1069812500.0, "imag / resp"=-3.481079}, {"real / stim"=1071343750.0, "imag / resp"=-3.4829102}, {"real / stim"=1072875000.0, "imag / resp"=-3.4838867}, {"real / stim"=1074406250.0, "imag / resp"=-3.4837646}, {"real / stim"=1075937500.0, "imag / resp"=-3.4854736}, {"real / stim"=1077468750.0, "imag / resp"=-3.4841309}, {"real / stim"=1079000000.0, "imag / resp"=-3.487915}, {"real / stim"=1080531250.0, "imag / resp"=-3.4907227}, {"real / stim"=1082062500.0, "imag / resp"=-3.4937744}, {"real / stim"=1083593750.0, "imag / resp"=-3.4938965}, {"real / stim"=1085125000.0, "imag / resp"=-3.498291}, {"real / stim"=1086656250.0, "imag / resp"=-3.5039062}, {"real / stim"=1088187500.0, "imag / resp"=-3.508667}, {"real / stim"=1089718750.0, "imag / resp"=-3.5117188}, {"real / stim"=1091250000.0, "imag / resp"=-3.5144043}, {"real / stim"=1092781250.0, "imag / resp"=-3.5184326}, {"real / stim"=1094312500.0, "imag / resp"=-3.5250244}, {"real / stim"=1095843750.0, "imag / resp"=-3.5289307}, {"real / stim"=1097375000.0, "imag / resp"=-3.536377}, {"real / stim"=1098906250.0, "imag / resp"=-3.5441895}, {"real / stim"=1100437500.0, "imag / resp"=-3.548706}, {"real / stim"=1101968750.0, "imag / resp"=-3.559082}, {"real / stim"=1103500000.0, "imag / resp"=-3.567749}, {"real / stim"=1105031250.0, "imag / resp"=-3.5739746}, {"real / stim"=1106562500.0, "imag / resp"=-3.5822754}, {"real / stim"=1108093750.0, "imag / resp"=-3.5888672}, {"real / stim"=1109625000.0, "imag / resp"=-3.6013184}, {"real / stim"=1111156250.0, "imag / resp"=-3.605835}, {"real / stim"=1112687500.0, "imag / resp"=-3.6142578}, {"real / stim"=1114218750.0, "imag / resp"=-3.6201172}, {"real / stim"=1115750000.0, "imag / resp"=-3.6317139}, {"real / stim"=1117281250.0, "imag / resp"=-3.6385498}, {"real / stim"=1118812500.0, "imag / resp"=-3.6501465}, {"real / stim"=1120343750.0, "imag / resp"=-3.6552734}, {"real / stim"=1121875000.0, "imag / resp"=-3.665039}, {"real / stim"=1123406250.0, "imag / resp"=-3.675293}, {"real / stim"=1124937500.0, "imag / resp"=-3.6831055}, {"real / stim"=1126468750.0, "imag / resp"=-3.692871}, {"real / stim"=1128000000.0, "imag / resp"=-3.7001953}, {"real / stim"=1129531250.0, "imag / resp"=-3.70813}, {"real / stim"=1131062500.0, "imag / resp"=-3.7164307}, {"real / stim"=1132593750.0, "imag / resp"=-3.7252197}, {"real / stim"=1134125000.0, "imag / resp"=-3.7302246}, {"real / stim"=1135656250.0, "imag / resp"=-3.741455}, {"real / stim"=1137187500.0, "imag / resp"=-3.7492676}, {"real / stim"=1138718750.0, "imag / resp"=-3.7556152}, {"real / stim"=1140250000.0, "imag / resp"=-3.7614746}, {"real / stim"=1141781250.0, "imag / resp"=-3.7717285}, {"real / stim"=1143312500.0, "imag / resp"=-3.777832}, {"real / stim"=1144843750.0, "imag / resp"=-3.7824707}, {"real / stim"=1146375000.0, "imag / resp"=-3.7896729}, {"real / stim"=1147906250.0, "imag / resp"=-3.7929688}, {"real / stim"=1149437500.0, "imag / resp"=-3.798706}, {"real / stim"=1150968750.0, "imag / resp"=-3.8051758}, {"real / stim"=1152500000.0, "imag / resp"=-3.8129883}, {"real / stim"=1154031250.0, "imag / resp"=-3.815796}, {"real / stim"=1155562500.0, "imag / resp"=-3.8222656}, {"real / stim"=1157093750.0, "imag / resp"=-3.8220215}, {"real / stim"=1158625000.0, "imag / resp"=-3.8272705}, {"real / stim"=1160156250.0, "imag / resp"=-3.831421}, {"real / stim"=1161687500.0, "imag / resp"=-3.8342285}, {"real / stim"=1163218750.0, "imag / resp"=-3.8389893}, {"real / stim"=1164750000.0, "imag / resp"=-3.8457031}, {"real / stim"=1166281250.0, "imag / resp"=-3.8481445}, {"real / stim"=1167812500.0, "imag / resp"=-3.85437}, {"real / stim"=1169343750.0, "imag / resp"=-3.8603516}, {"real / stim"=1170875000.0, "imag / resp"=-3.8613281}, {"real / stim"=1172406250.0, "imag / resp"=-3.8706055}, {"real / stim"=1173937500.0, "imag / resp"=-3.8745117}, {"real / stim"=1175468750.0, "imag / resp"=-3.8824463}, {"real / stim"=1177000000.0, "imag / resp"=-3.8867188}, {"real / stim"=1178531250.0, "imag / resp"=-3.8934326}, {"real / stim"=1180062500.0, "imag / resp"=-3.8989258}, {"real / stim"=1181593750.0, "imag / resp"=-3.907959}, {"real / stim"=1183125000.0, "imag / resp"=-3.9172363}, {"real / stim"=1184656250.0, "imag / resp"=-3.9246826}, {"real / stim"=1186187500.0, "imag / resp"=-3.9372559}, {"real / stim"=1187718750.0, "imag / resp"=-3.9468994}, {"real / stim"=1189250000.0, "imag / resp"=-3.9558105}, {"real / stim"=1190781250.0, "imag / resp"=-3.9692383}, {"real / stim"=1192312500.0, "imag / resp"=-3.980713}, {"real / stim"=1193843750.0, "imag / resp"=-3.9919434}, {"real / stim"=1195375000.0, "imag / resp"=-4.0058594}, {"real / stim"=1196906250.0, "imag / resp"=-4.0161133}, {"real / stim"=1198437500.0, "imag / resp"=-4.0334473}, {"real / stim"=1199968750.0, "imag / resp"=-4.0456543}, {"real / stim"=1201500000.0, "imag / resp"=-4.0634766}, {"real / stim"=1203031250.0, "imag / resp"=-4.074463}, {"real / stim"=1204562500.0, "imag / resp"=-4.0944824}, {"real / stim"=1206093750.0, "imag / resp"=-4.1105957}, {"real / stim"=1207625000.0, "imag / resp"=-4.1279297}, {"real / stim"=1209156250.0, "imag / resp"=-4.140625}, {"real / stim"=1210687500.0, "imag / resp"=-4.161377}, {"real / stim"=1212218750.0, "imag / resp"=-4.1726074}, {"real / stim"=1213750000.0, "imag / resp"=-4.1882324}, {"real / stim"=1215281250.0, "imag / resp"=-4.2109375}, {"real / stim"=1216812500.0, "imag / resp"=-4.2248535}, {"real / stim"=1218343750.0, "imag / resp"=-4.243164}, {"real / stim"=1219875000.0, "imag / resp"=-4.2612305}, {"real / stim"=1221406250.0, "imag / resp"=-4.279541}, {"real / stim"=1222937500.0, "imag / resp"=-4.2980957}, {"real / stim"=1224468750.0, "imag / resp"=-4.3137207}, {"real / stim"=1226000000.0, "imag / resp"=-4.335205}, {"real / stim"=1227531250.0, "imag / resp"=-4.352539}, {"real / stim"=1229062500.0, "imag / resp"=-4.371826}, {"real / stim"=1230593750.0, "imag / resp"=-4.3916016}, {"real / stim"=1232125000.0, "imag / resp"=-4.409912}, {"real / stim"=1233656250.0, "imag / resp"=-4.430664}, {"real / stim"=1235187500.0, "imag / resp"=-4.4519043}, {"real / stim"=1236718750.0, "imag / resp"=-4.468994}, {"real / stim"=1238250000.0, "imag / resp"=-4.4919434}, {"real / stim"=1239781250.0, "imag / resp"=-4.5097656}, {"real / stim"=1241312500.0, "imag / resp"=-4.5319824}, {"real / stim"=1242843750.0, "imag / resp"=-4.554199}, {"real / stim"=1244375000.0, "imag / resp"=-4.574951}, {"real / stim"=1245906250.0, "imag / resp"=-4.597168}, {"real / stim"=1247437500.0, "imag / resp"=-4.6186523}, {"real / stim"=1248968750.0, "imag / resp"=-4.6398926}, {"real / stim"=1250500000.0, "imag / resp"=-4.664795}, {"real / stim"=1252031250.0, "imag / resp"=-4.685791}, {"real / stim"=1253562500.0, "imag / resp"=-4.71167}, {"real / stim"=1255093750.0, "imag / resp"=-4.731201}, {"real / stim"=1256625000.0, "imag / resp"=-4.755127}, {"real / stim"=1258156250.0, "imag / resp"=-4.776367}, {"real / stim"=1259687500.0, "imag / resp"=-4.8032227}, {"real / stim"=1261218750.0, "imag / resp"=-4.8237305}, {"real / stim"=1262750000.0, "imag / resp"=-4.8500977}, {"real / stim"=1264281250.0, "imag / resp"=-4.878662}, {"real / stim"=1265812500.0, "imag / resp"=-4.898926}, {"real / stim"=1267343750.0, "imag / resp"=-4.9257812}, {"real / stim"=1268875000.0, "imag / resp"=-4.951172}, {"real / stim"=1270406250.0, "imag / resp"=-4.9797363}, {"real / stim"=1271937500.0, "imag / resp"=-5.005615}, {"real / stim"=1273468750.0, "imag / resp"=-5.0317383}, {"real / stim"=1275000000.0, "imag / resp"=-5.064209}, {"real / stim"=1276531250.0, "imag / resp"=-5.090088}, {"real / stim"=1278062500.0, "imag / resp"=-5.1208496}, {"real / stim"=1279593750.0, "imag / resp"=-5.1540527}, {"real / stim"=1281125000.0, "imag / resp"=-5.1853027}, {"real / stim"=1282656250.0, "imag / resp"=-5.2177734}, {"real / stim"=1284187500.0, "imag / resp"=-5.253662}, {"real / stim"=1285718750.0, "imag / resp"=-5.2856445}, {"real / stim"=1287250000.0, "imag / resp"=-5.32251}, {"real / stim"=1288781250.0, "imag / resp"=-5.362793}, {"real / stim"=1290312500.0, "imag / resp"=-5.3984375}, {"real / stim"=1291843750.0, "imag / resp"=-5.437744}, {"real / stim"=1293375000.0, "imag / resp"=-5.477783}, {"real / stim"=1294906250.0, "imag / resp"=-5.5166016}, {"real / stim"=1296437500.0, "imag / resp"=-5.5617676}, {"real / stim"=1297968750.0, "imag / resp"=-5.604248}, {"real / stim"=1299500000.0, "imag / resp"=-5.644287}, {"real / stim"=1301031250.0, "imag / resp"=-5.6896973}, {"real / stim"=1302562500.0, "imag / resp"=-5.734375}, {"real / stim"=1304093750.0, "imag / resp"=-5.779297}, {"real / stim"=1305625000.0, "imag / resp"=-5.8239746}, {"real / stim"=1307156250.0, "imag / resp"=-5.8720703}, {"real / stim"=1308687500.0, "imag / resp"=-5.9189453}, {"real / stim"=1310218750.0, "imag / resp"=-5.966797}, {"real / stim"=1311750000.0, "imag / resp"=-6.0129395}, {"real / stim"=1313281250.0, "imag / resp"=-6.0632324}, {"real / stim"=1314812500.0, "imag / resp"=-6.114258}, {"real / stim"=1316343750.0, "imag / resp"=-6.163086}, {"real / stim"=1317875000.0, "imag / resp"=-6.215576}, {"real / stim"=1319406250.0, "imag / resp"=-6.2651367}, {"real / stim"=1320937500.0, "imag / resp"=-6.315674}, {"real / stim"=1322468750.0, "imag / resp"=-6.369873}, {"real / stim"=1324000000.0, "imag / resp"=-6.419922}, {"real / stim"=1325531250.0, "imag / resp"=-6.472412}, {"real / stim"=1327062500.0, "imag / resp"=-6.524414}, {"real / stim"=1328593750.0, "imag / resp"=-6.581543}, {"real / stim"=1330125000.0, "imag / resp"=-6.6325684}, {"real / stim"=1331656250.0, "imag / resp"=-6.684082}, {"real / stim"=1333187500.0, "imag / resp"=-6.739746}, {"real / stim"=1334718750.0, "imag / resp"=-6.793213}, {"real / stim"=1336250000.0, "imag / resp"=-6.8481445}, {"real / stim"=1337781250.0, "imag / resp"=-6.9018555}, {"real / stim"=1339312500.0, "imag / resp"=-6.956787}, {"real / stim"=1340843750.0, "imag / resp"=-7.0131836}, {"real / stim"=1342375000.0, "imag / resp"=-7.071533}, {"real / stim"=1343906250.0, "imag / resp"=-7.1271973}, {"real / stim"=1345437500.0, "imag / resp"=-7.18042}, {"real / stim"=1346968750.0, "imag / resp"=-7.236084}, {"real / stim"=1348500000.0, "imag / resp"=-7.29126}, {"real / stim"=1350031250.0, "imag / resp"=-7.347412}, {"real / stim"=1351562500.0, "imag / resp"=-7.4016113}, {"real / stim"=1353093750.0, "imag / resp"=-7.4553223}, {"real / stim"=1354625000.0, "imag / resp"=-7.512207}, {"real / stim"=1356156250.0, "imag / resp"=-7.567627}, {"real / stim"=1357687500.0, "imag / resp"=-7.618408}, {"real / stim"=1359218750.0, "imag / resp"=-7.671875}, {"real / stim"=1360750000.0, "imag / resp"=-7.7282715}, {"real / stim"=1362281250.0, "imag / resp"=-7.783203}, {"real / stim"=1363812500.0, "imag / resp"=-7.8320312}, {"real / stim"=1365343750.0, "imag / resp"=-7.883789}, {"real / stim"=1366875000.0, "imag / resp"=-7.9401855}, {"real / stim"=1368406250.0, "imag / resp"=-7.9919434}, {"real / stim"=1369937500.0, "imag / resp"=-8.044434}, {"real / stim"=1371468750.0, "imag / resp"=-8.097168}, {"real / stim"=1373000000.0, "imag / resp"=-8.150391}, {"real / stim"=1374531250.0, "imag / resp"=-8.205566}, {"real / stim"=1376062500.0, "imag / resp"=-8.255371}, {"real / stim"=1377593750.0, "imag / resp"=-8.312988}, {"real / stim"=1379125000.0, "imag / resp"=-8.361816}, {"real / stim"=1380656250.0, "imag / resp"=-8.416504}, {"real / stim"=1382187500.0, "imag / resp"=-8.469238}, {"real / stim"=1383718750.0, "imag / resp"=-8.521973}, {"real / stim"=1385250000.0, "imag / resp"=-8.572754}, {"real / stim"=1386781250.0, "imag / resp"=-8.625977}, {"real / stim"=1388312500.0, "imag / resp"=-8.681152}, {"real / stim"=1389843750.0, "imag / resp"=-8.731445}, {"real / stim"=1391375000.0, "imag / resp"=-8.786133}, {"real / stim"=1392906250.0, "imag / resp"=-8.838379}, {"real / stim"=1394437500.0, "imag / resp"=-8.891113}, {"real / stim"=1395968750.0, "imag / resp"=-8.938477}, {"real / stim"=1397500000.0, "imag / resp"=-8.993164}, {"real / stim"=1399031250.0, "imag / resp"=-9.042969}, {"real / stim"=1400562500.0, "imag / resp"=-9.093262}, {"real / stim"=1402093750.0, "imag / resp"=-9.140137}, {"real / stim"=1403625000.0, "imag / resp"=-9.189453}, {"real / stim"=1405156250.0, "imag / resp"=-9.236328}, {"real / stim"=1406687500.0, "imag / resp"=-9.28125}, {"real / stim"=1408218750.0, "imag / resp"=-9.32666}, {"real / stim"=1409750000.0, "imag / resp"=-9.368652}, {"real / stim"=1411281250.0, "imag / resp"=-9.412109}, {"real / stim"=1412812500.0, "imag / resp"=-9.452637}, {"real / stim"=1414343750.0, "imag / resp"=-9.495605}, {"real / stim"=1415875000.0, "imag / resp"=-9.534668}, {"real / stim"=1417406250.0, "imag / resp"=-9.572754}, {"real / stim"=1418937500.0, "imag / resp"=-9.60791}, {"real / stim"=1420468750.0, "imag / resp"=-9.641113}, {"real / stim"=1422000000.0, "imag / resp"=-9.674316}, {"real / stim"=1423531250.0, "imag / resp"=-9.703613}, {"real / stim"=1425062500.0, "imag / resp"=-9.73291}, {"real / stim"=1426593750.0, "imag / resp"=-9.755859}, {"real / stim"=1428125000.0, "imag / resp"=-9.783203}, {"real / stim"=1429656250.0, "imag / resp"=-9.803711}, {"real / stim"=1431187500.0, "imag / resp"=-9.82373}, {"real / stim"=1432718750.0, "imag / resp"=-9.845215}, {"real / stim"=1434250000.0, "imag / resp"=-9.858887}, {"real / stim"=1435781250.0, "imag / resp"=-9.873535}, {"real / stim"=1437312500.0, "imag / resp"=-9.881836}, {"real / stim"=1438843750.0, "imag / resp"=-9.89209}, {"real / stim"=1440375000.0, "imag / resp"=-9.8984375}, {"real / stim"=1441906250.0, "imag / resp"=-9.901855}, {"real / stim"=1443437500.0, "imag / resp"=-9.908203}, {"real / stim"=1444968750.0, "imag / resp"=-9.912598}, {"real / stim"=1446500000.0, "imag / resp"=-9.907715}, {"real / stim"=1448031250.0, "imag / resp"=-9.904785}, {"real / stim"=1449562500.0, "imag / resp"=-9.901367}, {"real / stim"=1451093750.0, "imag / resp"=-9.893066}, {"real / stim"=1452625000.0, "imag / resp"=-9.888672}, {"real / stim"=1454156250.0, "imag / resp"=-9.878418}, {"real / stim"=1455687500.0, "imag / resp"=-9.87207}, {"real / stim"=1457218750.0, "imag / resp"=-9.85791}, {"real / stim"=1458750000.0, "imag / resp"=-9.84375}, {"real / stim"=1460281250.0, "imag / resp"=-9.830566}, {"real / stim"=1461812500.0, "imag / resp"=-9.816895}, {"real / stim"=1463343750.0, "imag / resp"=-9.800293}, {"real / stim"=1464875000.0, "imag / resp"=-9.783691}, {"real / stim"=1466406250.0, "imag / resp"=-9.765625}, {"real / stim"=1467937500.0, "imag / resp"=-9.745605}, {"real / stim"=1469468750.0, "imag / resp"=-9.728027}, {"real / stim"=1471000000.0, "imag / resp"=-9.705078}, {"real / stim"=1472531250.0, "imag / resp"=-9.689453}, {"real / stim"=1474062500.0, "imag / resp"=-9.6640625}, {"real / stim"=1475593750.0, "imag / resp"=-9.643555}, {"real / stim"=1477125000.0, "imag / resp"=-9.617676}, {"real / stim"=1478656250.0, "imag / resp"=-9.596191}, {"real / stim"=1480187500.0, "imag / resp"=-9.568359}, {"real / stim"=1481718750.0, "imag / resp"=-9.54541}, {"real / stim"=1483250000.0, "imag / resp"=-9.518555}, {"real / stim"=1484781250.0, "imag / resp"=-9.495605}, {"real / stim"=1486312500.0, "imag / resp"=-9.464355}, {"real / stim"=1487843750.0, "imag / resp"=-9.436035}, {"real / stim"=1489375000.0, "imag / resp"=-9.40918}, {"real / stim"=1490906250.0, "imag / resp"=-9.376953}, {"real / stim"=1492437500.0, "imag / resp"=-9.347656}, {"real / stim"=1493968750.0, "imag / resp"=-9.320801}, {"real / stim"=1495500000.0, "imag / resp"=-9.290039}, {"real / stim"=1497031250.0, "imag / resp"=-9.258301}, {"real / stim"=1498562500.0, "imag / resp"=-9.227051}, {"real / stim"=1500093750.0, "imag / resp"=-9.191895}, {"real / stim"=1501625000.0, "imag / resp"=-9.162598}, {"real / stim"=1503156250.0, "imag / resp"=-9.122559}, {"real / stim"=1504687500.0, "imag / resp"=-9.090332}, {"real / stim"=1506218750.0, "imag / resp"=-9.057617}, {"real / stim"=1507750000.0, "imag / resp"=-9.023926}, {"real / stim"=1509281250.0, "imag / resp"=-8.988281}, {"real / stim"=1510812500.0, "imag / resp"=-8.949219}, {"real / stim"=1512343750.0, "imag / resp"=-8.911133}, {"real / stim"=1513875000.0, "imag / resp"=-8.871582}, {"real / stim"=1515406250.0, "imag / resp"=-8.836426}, {"real / stim"=1516937500.0, "imag / resp"=-8.795898}, {"real / stim"=1518468750.0, "imag / resp"=-8.76123}, {"real / stim"=1520000000.0, "imag / resp"=-8.720703}, {"real / stim"=1521531250.0, "imag / resp"=-8.682129}, {"real / stim"=1523062500.0, "imag / resp"=-8.642578}, {"real / stim"=1524593750.0, "imag / resp"=-8.599609}, {"real / stim"=1526125000.0, "imag / resp"=-8.563965}, {"real / stim"=1527656250.0, "imag / resp"=-8.52002}, {"real / stim"=1529187500.0, "imag / resp"=-8.484863}, {"real / stim"=1530718750.0, "imag / resp"=-8.444336}, {"real / stim"=1532250000.0, "imag / resp"=-8.407227}, {"real / stim"=1533781250.0, "imag / resp"=-8.36377}, {"real / stim"=1535312500.0, "imag / resp"=-8.325684}, {"real / stim"=1536843750.0, "imag / resp"=-8.286621}, {"real / stim"=1538375000.0, "imag / resp"=-8.245117}, {"real / stim"=1539906250.0, "imag / resp"=-8.209473}, {"real / stim"=1541437500.0, "imag / resp"=-8.171387}, {"real / stim"=1542968750.0, "imag / resp"=-8.1328125}, {"real / stim"=1544500000.0, "imag / resp"=-8.097168}, {"real / stim"=1546031250.0, "imag / resp"=-8.054199}, {"real / stim"=1547562500.0, "imag / resp"=-8.021973}, {"real / stim"=1549093750.0, "imag / resp"=-7.9836426}, {"real / stim"=1550625000.0, "imag / resp"=-7.946289}, {"real / stim"=1552156250.0, "imag / resp"=-7.9089355}, {"real / stim"=1553687500.0, "imag / resp"=-7.875}, {"real / stim"=1555218750.0, "imag / resp"=-7.840332}, {"real / stim"=1556750000.0, "imag / resp"=-7.802246}, {"real / stim"=1558281250.0, "imag / resp"=-7.7678223}, {"real / stim"=1559812500.0, "imag / resp"=-7.7382812}, {"real / stim"=1561343750.0, "imag / resp"=-7.7036133}, {"real / stim"=1562875000.0, "imag / resp"=-7.6730957}, {"real / stim"=1564406250.0, "imag / resp"=-7.6428223}, {"real / stim"=1565937500.0, "imag / resp"=-7.6064453}, {"real / stim"=1567468750.0, "imag / resp"=-7.5751953}, {"real / stim"=1569000000.0, "imag / resp"=-7.5461426}, {"real / stim"=1570531250.0, "imag / resp"=-7.5148926}, {"real / stim"=1572062500.0, "imag / resp"=-7.4890137}, {"real / stim"=1573593750.0, "imag / resp"=-7.4560547}, {"real / stim"=1575125000.0, "imag / resp"=-7.429199}, {"real / stim"=1576656250.0, "imag / resp"=-7.404541}, {"real / stim"=1578187500.0, "imag / resp"=-7.3759766}, {"real / stim"=1579718750.0, "imag / resp"=-7.348877}, {"real / stim"=1581250000.0, "imag / resp"=-7.32251}, {"real / stim"=1582781250.0, "imag / resp"=-7.2963867}, {"real / stim"=1584312500.0, "imag / resp"=-7.270752}, {"real / stim"=1585843750.0, "imag / resp"=-7.240967}, {"real / stim"=1587375000.0, "imag / resp"=-7.2194824}, {"real / stim"=1588906250.0, "imag / resp"=-7.194092}, {"real / stim"=1590437500.0, "imag / resp"=-7.1679688}, {"real / stim"=1591968750.0, "imag / resp"=-7.1450195}, {"real / stim"=1593500000.0, "imag / resp"=-7.1191406}, {"real / stim"=1595031250.0, "imag / resp"=-7.095459}, {"real / stim"=1596562500.0, "imag / resp"=-7.072754}, {"real / stim"=1598093750.0, "imag / resp"=-7.046875}, {"real / stim"=1599625000.0, "imag / resp"=-7.0249023}, {"real / stim"=1601156250.0, "imag / resp"=-7.0046387}, {"real / stim"=1602687500.0, "imag / resp"=-6.9821777}, {"real / stim"=1604218750.0, "imag / resp"=-6.960449}, {"real / stim"=1605750000.0, "imag / resp"=-6.935791}, {"real / stim"=1607281250.0, "imag / resp"=-6.919922}, {"real / stim"=1608812500.0, "imag / resp"=-6.900879}, {"real / stim"=1610343750.0, "imag / resp"=-6.8776855}, {"real / stim"=1611875000.0, "imag / resp"=-6.8586426}, {"real / stim"=1613406250.0, "imag / resp"=-6.8359375}, {"real / stim"=1614937500.0, "imag / resp"=-6.819824}, {"real / stim"=1616468750.0, "imag / resp"=-6.8032227}, {"real / stim"=1618000000.0, "imag / resp"=-6.7802734}, {"real / stim"=1619531250.0, "imag / resp"=-6.7668457}, {"real / stim"=1621062500.0, "imag / resp"=-6.748047}, {"real / stim"=1622593750.0, "imag / resp"=-6.732666}, {"real / stim"=1624125000.0, "imag / resp"=-6.7141113}, {"real / stim"=1625656250.0, "imag / resp"=-6.7038574}, {"real / stim"=1627187500.0, "imag / resp"=-6.6862793}, {"real / stim"=1628718750.0, "imag / resp"=-6.6706543}, {"real / stim"=1630250000.0, "imag / resp"=-6.6621094}, {"real / stim"=1631781250.0, "imag / resp"=-6.647217}, {"real / stim"=1633312500.0, "imag / resp"=-6.640381}, {"real / stim"=1634843750.0, "imag / resp"=-6.625244}, {"real / stim"=1636375000.0, "imag / resp"=-6.618164}, {"real / stim"=1637906250.0, "imag / resp"=-6.6049805}, {"real / stim"=1639437500.0, "imag / resp"=-6.599121}, {"real / stim"=1640968750.0, "imag / resp"=-6.5895996}, {"real / stim"=1642500000.0, "imag / resp"=-6.578369}, {"real / stim"=1644031250.0, "imag / resp"=-6.5756836}, {"real / stim"=1645562500.0, "imag / resp"=-6.5668945}, {"real / stim"=1647093750.0, "imag / resp"=-6.5620117}, {"real / stim"=1648625000.0, "imag / resp"=-6.555908}, {"real / stim"=1650156250.0, "imag / resp"=-6.5498047}, {"real / stim"=1651687500.0, "imag / resp"=-6.546875}, {"real / stim"=1653218750.0, "imag / resp"=-6.5495605}, {"real / stim"=1654750000.0, "imag / resp"=-6.5458984}, {"real / stim"=1656281250.0, "imag / resp"=-6.5463867}, {"real / stim"=1657812500.0, "imag / resp"=-6.5495605}, {"real / stim"=1659343750.0, "imag / resp"=-6.5463867}, {"real / stim"=1660875000.0, "imag / resp"=-6.548828}, {"real / stim"=1662406250.0, "imag / resp"=-6.553467}, {"real / stim"=1663937500.0, "imag / resp"=-6.5583496}, {"real / stim"=1665468750.0, "imag / resp"=-6.562256}, {"real / stim"=1667000000.0, "imag / resp"=-6.5686035}, {"real / stim"=1668531250.0, "imag / resp"=-6.5754395}, {"real / stim"=1670062500.0, "imag / resp"=-6.581299}, {"real / stim"=1671593750.0, "imag / resp"=-6.5910645}, {"real / stim"=1673125000.0, "imag / resp"=-6.602295}, {"real / stim"=1674656250.0, "imag / resp"=-6.6118164}, {"real / stim"=1676187500.0, "imag / resp"=-6.6210938}, {"real / stim"=1677718750.0, "imag / resp"=-6.6330566}, {"real / stim"=1679250000.0, "imag / resp"=-6.644287}, {"real / stim"=1680781250.0, "imag / resp"=-6.6569824}, {"real / stim"=1682312500.0, "imag / resp"=-6.669922}, {"real / stim"=1683843750.0, "imag / resp"=-6.6845703}, {"real / stim"=1685375000.0, "imag / resp"=-6.7004395}, {"real / stim"=1686906250.0, "imag / resp"=-6.71167}, {"real / stim"=1688437500.0, "imag / resp"=-6.7263184}, {"real / stim"=1689968750.0, "imag / resp"=-6.7441406}, {"real / stim"=1691500000.0, "imag / resp"=-6.7595215}, {"real / stim"=1693031250.0, "imag / resp"=-6.7753906}, {"real / stim"=1694562500.0, "imag / resp"=-6.7929688}, {"real / stim"=1696093750.0, "imag / resp"=-6.809326}, {"real / stim"=1697625000.0, "imag / resp"=-6.824951}, {"real / stim"=1699156250.0, "imag / resp"=-6.840332}, {"real / stim"=1700687500.0, "imag / resp"=-6.86084}, {"real / stim"=1702218750.0, "imag / resp"=-6.876465}, {"real / stim"=1703750000.0, "imag / resp"=-6.894043}, {"real / stim"=1705281250.0, "imag / resp"=-6.911133}, {"real / stim"=1706812500.0, "imag / resp"=-6.925537}, {"real / stim"=1708343750.0, "imag / resp"=-6.942627}, {"real / stim"=1709875000.0, "imag / resp"=-6.960449}, {"real / stim"=1711406250.0, "imag / resp"=-6.979248}, {"real / stim"=1712937500.0, "imag / resp"=-6.99292}, {"real / stim"=1714468750.0, "imag / resp"=-7.0126953}, {"real / stim"=1716000000.0, "imag / resp"=-7.0319824}, {"real / stim"=1717531250.0, "imag / resp"=-7.04541}, {"real / stim"=1719062500.0, "imag / resp"=-7.0620117}, {"real / stim"=1720593750.0, "imag / resp"=-7.080078}, {"real / stim"=1722125000.0, "imag / resp"=-7.0930176}, {"real / stim"=1723656250.0, "imag / resp"=-7.1098633}, {"real / stim"=1725187500.0, "imag / resp"=-7.125244}, {"real / stim"=1726718750.0, "imag / resp"=-7.1401367}, {"real / stim"=1728250000.0, "imag / resp"=-7.1569824}, {"real / stim"=1729781250.0, "imag / resp"=-7.168213}, {"real / stim"=1731312500.0, "imag / resp"=-7.1831055}, {"real / stim"=1732843750.0, "imag / resp"=-7.191162}, {"real / stim"=1734375000.0, "imag / resp"=-7.20459}, {"real / stim"=1735906250.0, "imag / resp"=-7.2158203}, {"real / stim"=1737437500.0, "imag / resp"=-7.2226562}, {"real / stim"=1738968750.0, "imag / resp"=-7.2336426}, {"real / stim"=1740500000.0, "imag / resp"=-7.23999}, {"real / stim"=1742031250.0, "imag / resp"=-7.2470703}, {"real / stim"=1743562500.0, "imag / resp"=-7.253418}, {"real / stim"=1745093750.0, "imag / resp"=-7.2546387}, {"real / stim"=1746625000.0, "imag / resp"=-7.2578125}, {"real / stim"=1748156250.0, "imag / resp"=-7.259033}, {"real / stim"=1749687500.0, "imag / resp"=-7.2614746}, {"real / stim"=1751218750.0, "imag / resp"=-7.2597656}, {"real / stim"=1752750000.0, "imag / resp"=-7.2578125}, {"real / stim"=1754281250.0, "imag / resp"=-7.25708}, {"real / stim"=1755812500.0, "imag / resp"=-7.253174}, {"real / stim"=1757343750.0, "imag / resp"=-7.246582}, {"real / stim"=1758875000.0, "imag / resp"=-7.242676}, {"real / stim"=1760406250.0, "imag / resp"=-7.229248}, {"real / stim"=1761937500.0, "imag / resp"=-7.2231445}, {"real / stim"=1763468750.0, "imag / resp"=-7.209961}, {"real / stim"=1765000000.0, "imag / resp"=-7.19751}, {"real / stim"=1766531250.0, "imag / resp"=-7.184326}, {"real / stim"=1768062500.0, "imag / resp"=-7.1660156}, {"real / stim"=1769593750.0, "imag / resp"=-7.1516113}, {"real / stim"=1771125000.0, "imag / resp"=-7.133301}, {"real / stim"=1772656250.0, "imag / resp"=-7.1154785}, {"real / stim"=1774187500.0, "imag / resp"=-7.093506}, {"real / stim"=1775718750.0, "imag / resp"=-7.069092}, {"real / stim"=1777250000.0, "imag / resp"=-7.0476074}, {"real / stim"=1778781250.0, "imag / resp"=-7.023926}, {"real / stim"=1780312500.0, "imag / resp"=-6.999756}, {"real / stim"=1781843750.0, "imag / resp"=-6.970459}, {"real / stim"=1783375000.0, "imag / resp"=-6.947998}, {"real / stim"=1784906250.0, "imag / resp"=-6.914795}, {"real / stim"=1786437500.0, "imag / resp"=-6.887207}, {"real / stim"=1787968750.0, "imag / resp"=-6.854492}, {"real / stim"=1789500000.0, "imag / resp"=-6.821045}, {"real / stim"=1791031250.0, "imag / resp"=-6.7922363}, {"real / stim"=1792562500.0, "imag / resp"=-6.7612305}, {"real / stim"=1794093750.0, "imag / resp"=-6.727295}, {"real / stim"=1795625000.0, "imag / resp"=-6.688965}, {"real / stim"=1797156250.0, "imag / resp"=-6.6520996}, {"real / stim"=1798687500.0, "imag / resp"=-6.6169434}, {"real / stim"=1800218750.0, "imag / resp"=-6.5788574}, {"real / stim"=1801750000.0, "imag / resp"=-6.540039}, {"real / stim"=1803281250.0, "imag / resp"=-6.501709}, {"real / stim"=1804812500.0, "imag / resp"=-6.467285}, {"real / stim"=1806343750.0, "imag / resp"=-6.4333496}, {"real / stim"=1807875000.0, "imag / resp"=-6.3916016}, {"real / stim"=1809406250.0, "imag / resp"=-6.3535156}, {"real / stim"=1810937500.0, "imag / resp"=-6.3154297}, {"real / stim"=1812468750.0, "imag / resp"=-6.2785645}, {"real / stim"=1814000000.0, "imag / resp"=-6.238037}, {"real / stim"=1815531250.0, "imag / resp"=-6.199463}, {"real / stim"=1817062500.0, "imag / resp"=-6.159424}, {"real / stim"=1818593750.0, "imag / resp"=-6.1223145}, {"real / stim"=1820125000.0, "imag / resp"=-6.0844727}, {"real / stim"=1821656250.0, "imag / resp"=-6.0495605}, {"real / stim"=1823187500.0, "imag / resp"=-6.012207}, {"real / stim"=1824718750.0, "imag / resp"=-5.9750977}, {"real / stim"=1826250000.0, "imag / resp"=-5.940918}, {"real / stim"=1827781250.0, "imag / resp"=-5.9069824}, {"real / stim"=1829312500.0, "imag / resp"=-5.8669434}, {"real / stim"=1830843750.0, "imag / resp"=-5.8339844}, {"real / stim"=1832375000.0, "imag / resp"=-5.800537}, {"real / stim"=1833906250.0, "imag / resp"=-5.763916}, {"real / stim"=1835437500.0, "imag / resp"=-5.7319336}, {"real / stim"=1836968750.0, "imag / resp"=-5.696533}, {"real / stim"=1838500000.0, "imag / resp"=-5.6672363}, {"real / stim"=1840031250.0, "imag / resp"=-5.6342773}, {"real / stim"=1841562500.0, "imag / resp"=-5.598633}, {"real / stim"=1843093750.0, "imag / resp"=-5.569824}, {"real / stim"=1844625000.0, "imag / resp"=-5.5407715}, {"real / stim"=1846156250.0, "imag / resp"=-5.509033}, {"real / stim"=1847687500.0, "imag / resp"=-5.4726562}, {"real / stim"=1849218750.0, "imag / resp"=-5.445801}, {"real / stim"=1850750000.0, "imag / resp"=-5.41333}, {"real / stim"=1852281250.0, "imag / resp"=-5.3828125}, {"real / stim"=1853812500.0, "imag / resp"=-5.3566895}, {"real / stim"=1855343750.0, "imag / resp"=-5.3342285}, {"real / stim"=1856875000.0, "imag / resp"=-5.307129}, {"real / stim"=1858406250.0, "imag / resp"=-5.282959}, {"real / stim"=1859937500.0, "imag / resp"=-5.2578125}, {"real / stim"=1861468750.0, "imag / resp"=-5.230713}, {"real / stim"=1863000000.0, "imag / resp"=-5.206543}, {"real / stim"=1864531250.0, "imag / resp"=-5.182373}, {"real / stim"=1866062500.0, "imag / resp"=-5.165039}, {"real / stim"=1867593750.0, "imag / resp"=-5.1396484}, {"real / stim"=1869125000.0, "imag / resp"=-5.119385}, {"real / stim"=1870656250.0, "imag / resp"=-5.1013184}, {"real / stim"=1872187500.0, "imag / resp"=-5.08374}, {"real / stim"=1873718750.0, "imag / resp"=-5.0651855}, {"real / stim"=1875250000.0, "imag / resp"=-5.0480957}, {"real / stim"=1876781250.0, "imag / resp"=-5.0302734}, {"real / stim"=1878312500.0, "imag / resp"=-5.0144043}, {"real / stim"=1879843750.0, "imag / resp"=-4.9992676}, {"real / stim"=1881375000.0, "imag / resp"=-4.980713}, {"real / stim"=1882906250.0, "imag / resp"=-4.967041}, {"real / stim"=1884437500.0, "imag / resp"=-4.949463}, {"real / stim"=1885968750.0, "imag / resp"=-4.9313965}, {"real / stim"=1887500000.0, "imag / resp"=-4.916992}, {"real / stim"=1889031250.0, "imag / resp"=-4.9040527}, {"real / stim"=1890562500.0, "imag / resp"=-4.888672}, {"real / stim"=1892093750.0, "imag / resp"=-4.8710938}, {"real / stim"=1893625000.0, "imag / resp"=-4.8586426}, {"real / stim"=1895156250.0, "imag / resp"=-4.841797}, {"real / stim"=1896687500.0, "imag / resp"=-4.8291016}, {"real / stim"=1898218750.0, "imag / resp"=-4.811035}, {"real / stim"=1899750000.0, "imag / resp"=-4.79834}, {"real / stim"=1901281250.0, "imag / resp"=-4.7834473}, {"real / stim"=1902812500.0, "imag / resp"=-4.7666016}, {"real / stim"=1904343750.0, "imag / resp"=-4.7526855}, {"real / stim"=1905875000.0, "imag / resp"=-4.734619}, {"real / stim"=1907406250.0, "imag / resp"=-4.720459}, {"real / stim"=1908937500.0, "imag / resp"=-4.704834}, {"real / stim"=1910468750.0, "imag / resp"=-4.6875}, {"real / stim"=1912000000.0, "imag / resp"=-4.6708984}, {"real / stim"=1913531250.0, "imag / resp"=-4.6557617}, {"real / stim"=1915062500.0, "imag / resp"=-4.6379395}, {"real / stim"=1916593750.0, "imag / resp"=-4.625244}, {"real / stim"=1918125000.0, "imag / resp"=-4.607422}, {"real / stim"=1919656250.0, "imag / resp"=-4.593506}, {"real / stim"=1921187500.0, "imag / resp"=-4.5791016}, {"real / stim"=1922718750.0, "imag / resp"=-4.562256}, {"real / stim"=1924250000.0, "imag / resp"=-4.5461426}, {"real / stim"=1925781250.0, "imag / resp"=-4.5300293}, {"real / stim"=1927312500.0, "imag / resp"=-4.5166016}, {"real / stim"=1928843750.0, "imag / resp"=-4.5007324}, {"real / stim"=1930375000.0, "imag / resp"=-4.4838867}, {"real / stim"=1931906250.0, "imag / resp"=-4.468994}, {"real / stim"=1933437500.0, "imag / resp"=-4.4541016}, {"real / stim"=1934968750.0, "imag / resp"=-4.439453}, {"real / stim"=1936500000.0, "imag / resp"=-4.425293}, {"real / stim"=1938031250.0, "imag / resp"=-4.4106445}, {"real / stim"=1939562500.0, "imag / resp"=-4.395996}, {"real / stim"=1941093750.0, "imag / resp"=-4.3813477}, {"real / stim"=1942625000.0, "imag / resp"=-4.3657227}, {"real / stim"=1944156250.0, "imag / resp"=-4.3515625}, {"real / stim"=1945687500.0, "imag / resp"=-4.338135}, {"real / stim"=1947218750.0, "imag / resp"=-4.323242}, {"real / stim"=1948750000.0, "imag / resp"=-4.3112793}, {"real / stim"=1950281250.0, "imag / resp"=-4.29834}, {"real / stim"=1951812500.0, "imag / resp"=-4.2839355}, {"real / stim"=1953343750.0, "imag / resp"=-4.2702637}, {"real / stim"=1954875000.0, "imag / resp"=-4.2592773}, {"real / stim"=1956406250.0, "imag / resp"=-4.2487793}, {"real / stim"=1957937500.0, "imag / resp"=-4.2304688}, {"real / stim"=1959468750.0, "imag / resp"=-4.2211914}, {"real / stim"=1961000000.0, "imag / resp"=-4.213867}, {"real / stim"=1962531250.0, "imag / resp"=-4.202881}, {"real / stim"=1964062500.0, "imag / resp"=-4.1901855}, {"real / stim"=1965593750.0, "imag / resp"=-4.179199}, {"real / stim"=1967125000.0, "imag / resp"=-4.1711426}, {"real / stim"=1968656250.0, "imag / resp"=-4.165039}, {"real / stim"=1970187500.0, "imag / resp"=-4.152588}, {"real / stim"=1971718750.0, "imag / resp"=-4.147217}, {"real / stim"=1973250000.0, "imag / resp"=-4.135498}, {"real / stim"=1974781250.0, "imag / resp"=-4.1293945}, {"real / stim"=1976312500.0, "imag / resp"=-4.1228027}, {"real / stim"=1977843750.0, "imag / resp"=-4.119385}, {"real / stim"=1979375000.0, "imag / resp"=-4.107666}, {"real / stim"=1980906250.0, "imag / resp"=-4.105713}, {"real / stim"=1982437500.0, "imag / resp"=-4.0998535}, {"real / stim"=1983968750.0, "imag / resp"=-4.090576}, {"real / stim"=1985500000.0, "imag / resp"=-4.087158}, {"real / stim"=1987031250.0, "imag / resp"=-4.0776367}, {"real / stim"=1988562500.0, "imag / resp"=-4.072998}, {"real / stim"=1990093750.0, "imag / resp"=-4.0649414}, {"real / stim"=1991625000.0, "imag / resp"=-4.057129}, {"real / stim"=1993156250.0, "imag / resp"=-4.0549316}, {"real / stim"=1994687500.0, "imag / resp"=-4.0473633}, {"real / stim"=1996218750.0, "imag / resp"=-4.0405273}, {"real / stim"=1997750000.0, "imag / resp"=-4.0356445}, {"real / stim"=1999281250.0, "imag / resp"=-4.0273438}, {"real / stim"=2000812500.0, "imag / resp"=-4.017578}, {"real / stim"=2002343750.0, "imag / resp"=-4.015381}, {"real / stim"=2003875000.0, "imag / resp"=-4.0046387}, {"real / stim"=2005406250.0, "imag / resp"=-3.9997559}, {"real / stim"=2006937500.0, "imag / resp"=-3.9918213}, {"real / stim"=2008468750.0, "imag / resp"=-3.986206}, {"real / stim"=2010000000.0, "imag / resp"=-3.977539}, {"real / stim"=2011531250.0, "imag / resp"=-3.9718018}, {"real / stim"=2013062500.0, "imag / resp"=-3.9674072}, {"real / stim"=2014593750.0, "imag / resp"=-3.956421}, {"real / stim"=2016125000.0, "imag / resp"=-3.9472656}, {"real / stim"=2017656250.0, "imag / resp"=-3.9422607}, {"real / stim"=2019187500.0, "imag / resp"=-3.9353027}, {"real / stim"=2020718750.0, "imag / resp"=-3.928711}, {"real / stim"=2022250000.0, "imag / resp"=-3.9207764}, {"real / stim"=2023781250.0, "imag / resp"=-3.9140625}, {"real / stim"=2025312500.0, "imag / resp"=-3.9055176}, {"real / stim"=2026843750.0, "imag / resp"=-3.901123}, {"real / stim"=2028375000.0, "imag / resp"=-3.8945312}, {"real / stim"=2029906250.0, "imag / resp"=-3.883667}, {"real / stim"=2031437500.0, "imag / resp"=-3.8762207}, {"real / stim"=2032968750.0, "imag / resp"=-3.8707275}, {"real / stim"=2034500000.0, "imag / resp"=-3.859253}, {"real / stim"=2036031250.0, "imag / resp"=-3.8570557}, {"real / stim"=2037562500.0, "imag / resp"=-3.8464355}, {"real / stim"=2039093750.0, "imag / resp"=-3.842163}, {"real / stim"=2040625000.0, "imag / resp"=-3.8321533}, {"real / stim"=2042156250.0, "imag / resp"=-3.8220215}, {"real / stim"=2043687500.0, "imag / resp"=-3.817505}, {"real / stim"=2045218750.0, "imag / resp"=-3.8083496}, {"real / stim"=2046750000.0, "imag / resp"=-3.800293}, {"real / stim"=2048281250.0, "imag / resp"=-3.7906494}, {"real / stim"=2049812500.0, "imag / resp"=-3.7860107}, {"real / stim"=2051343750.0, "imag / resp"=-3.7747803}, {"real / stim"=2052875000.0, "imag / resp"=-3.7714844}, {"real / stim"=2054406250.0, "imag / resp"=-3.7598877}, {"real / stim"=2055937500.0, "imag / resp"=-3.7537842}, {"real / stim"=2057468750.0, "imag / resp"=-3.7456055}, {"real / stim"=2059000000.0, "imag / resp"=-3.73938}, {"real / stim"=2060531250.0, "imag / resp"=-3.7329102}, {"real / stim"=2062062500.0, "imag / resp"=-3.7261963}, {"real / stim"=2063593750.0, "imag / resp"=-3.720337}, {"real / stim"=2065125000.0, "imag / resp"=-3.7145996}, {"real / stim"=2066656250.0, "imag / resp"=-3.7052002}, {"real / stim"=2068187500.0, "imag / resp"=-3.7003174}, {"real / stim"=2069718750.0, "imag / resp"=-3.6976318}, {"real / stim"=2071250000.0, "imag / resp"=-3.690918}, {"real / stim"=2072781250.0, "imag / resp"=-3.6905518}, {"real / stim"=2074312500.0, "imag / resp"=-3.6849365}, {"real / stim"=2075843750.0, "imag / resp"=-3.6782227}, {"real / stim"=2077375000.0, "imag / resp"=-3.6779785}, {"real / stim"=2078906250.0, "imag / resp"=-3.6756592}, {"real / stim"=2080437500.0, "imag / resp"=-3.675415}, {"real / stim"=2081968750.0, "imag / resp"=-3.6711426}, {"real / stim"=2083500000.0, "imag / resp"=-3.6693115}, {"real / stim"=2085031250.0, "imag / resp"=-3.6711426}, {"real / stim"=2086562500.0, "imag / resp"=-3.6625977}, {"real / stim"=2088093750.0, "imag / resp"=-3.6627197}, {"real / stim"=2089625000.0, "imag / resp"=-3.6600342}, {"real / stim"=2091156250.0, "imag / resp"=-3.6610107}, {"real / stim"=2092687500.0, "imag / resp"=-3.6569824}, {"real / stim"=2094218750.0, "imag / resp"=-3.6514893}, {"real / stim"=2095750000.0, "imag / resp"=-3.6507568}, {"real / stim"=2097281250.0, "imag / resp"=-3.6450195}, {"real / stim"=2098812500.0, "imag / resp"=-3.6408691}, {"real / stim"=2100343750.0, "imag / resp"=-3.6403809}, {"real / stim"=2101875000.0, "imag / resp"=-3.635498}, {"real / stim"=2103406250.0, "imag / resp"=-3.6292725}, {"real / stim"=2104937500.0, "imag / resp"=-3.626709}, {"real / stim"=2106468750.0, "imag / resp"=-3.6254883}, {"real / stim"=2108000000.0, "imag / resp"=-3.6166992}, {"real / stim"=2109531250.0, "imag / resp"=-3.61438}, {"real / stim"=2111062500.0, "imag / resp"=-3.6088867}, {"real / stim"=2112593750.0, "imag / resp"=-3.6052246}, {"real / stim"=2114125000.0, "imag / resp"=-3.5979004}, {"real / stim"=2115656250.0, "imag / resp"=-3.5957031}, {"real / stim"=2117187500.0, "imag / resp"=-3.5909424}, {"real / stim"=2118718750.0, "imag / resp"=-3.5847168}, {"real / stim"=2120250000.0, "imag / resp"=-3.5855713}, {"real / stim"=2121781250.0, "imag / resp"=-3.5770264}, {"real / stim"=2123312500.0, "imag / resp"=-3.5761719}, {"real / stim"=2124843750.0, "imag / resp"=-3.5655518}, {"real / stim"=2126375000.0, "imag / resp"=-3.5601807}, {"real / stim"=2127906250.0, "imag / resp"=-3.5568848}, {"real / stim"=2129437500.0, "imag / resp"=-3.552124}, {"real / stim"=2130968750.0, "imag / resp"=-3.5465088}, {"real / stim"=2132500000.0, "imag / resp"=-3.543335}, {"real / stim"=2134031250.0, "imag / resp"=-3.5371094}, {"real / stim"=2135562500.0, "imag / resp"=-3.5236816}, {"real / stim"=2137093750.0, "imag / resp"=-3.5180664}, {"real / stim"=2138625000.0, "imag / resp"=-3.5124512}, {"real / stim"=2140156250.0, "imag / resp"=-3.508789}, {"real / stim"=2141687500.0, "imag / resp"=-3.5019531}, {"real / stim"=2143218750.0, "imag / resp"=-3.496582}, {"real / stim"=2144750000.0, "imag / resp"=-3.482544}, {"real / stim"=2146281250.0, "imag / resp"=-3.4769287}, {"real / stim"=2147812500.0, "imag / resp"=-3.4666748}, {"real / stim"=2149343750.0, "imag / resp"=-3.4608154}, {"real / stim"=2150875000.0, "imag / resp"=-3.453125}, {"real / stim"=2152406250.0, "imag / resp"=-3.4439697}, {"real / stim"=2153937500.0, "imag / resp"=-3.4361572}, {"real / stim"=2155468750.0, "imag / resp"=-3.4310303}, {"real / stim"=2157000000.0, "imag / resp"=-3.421875}, {"real / stim"=2158531250.0, "imag / resp"=-3.4146729}, {"real / stim"=2160062500.0, "imag / resp"=-3.4055176}, {"real / stim"=2161593750.0, "imag / resp"=-3.3973389}, {"real / stim"=2163125000.0, "imag / resp"=-3.3886719}, {"real / stim"=2164656250.0, "imag / resp"=-3.3829346}, {"real / stim"=2166187500.0, "imag / resp"=-3.3770752}, {"real / stim"=2167718750.0, "imag / resp"=-3.3728027}, {"real / stim"=2169250000.0, "imag / resp"=-3.369873}, {"real / stim"=2170781250.0, "imag / resp"=-3.3620605}, {"real / stim"=2172312500.0, "imag / resp"=-3.3583984}, {"real / stim"=2173843750.0, "imag / resp"=-3.3518066}, {"real / stim"=2175375000.0, "imag / resp"=-3.3477783}, {"real / stim"=2176906250.0, "imag / resp"=-3.3464355}, {"real / stim"=2178437500.0, "imag / resp"=-3.3426514}, {"real / stim"=2179968750.0, "imag / resp"=-3.3370361}, {"real / stim"=2181500000.0, "imag / resp"=-3.3370361}, {"real / stim"=2183031250.0, "imag / resp"=-3.3354492}, {"real / stim"=2184562500.0, "imag / resp"=-3.333496}, {"real / stim"=2186093750.0, "imag / resp"=-3.3320312}, {"real / stim"=2187625000.0, "imag / resp"=-3.3306885}, {"real / stim"=2189156250.0, "imag / resp"=-3.328003}, {"real / stim"=2190687500.0, "imag / resp"=-3.3267822}, {"real / stim"=2192218750.0, "imag / resp"=-3.3275146}, {"real / stim"=2193750000.0, "imag / resp"=-3.3286133}, {"real / stim"=2195281250.0, "imag / resp"=-3.3291016}, {"real / stim"=2196812500.0, "imag / resp"=-3.328247}, {"real / stim"=2198343750.0, "imag / resp"=-3.3250732}, {"real / stim"=2199875000.0, "imag / resp"=-3.31958}, {"real / stim"=2201406250.0, "imag / resp"=-3.321289}, {"real / stim"=2202937500.0, "imag / resp"=-3.3187256}, {"real / stim"=2204468750.0, "imag / resp"=-3.3173828}, {"real / stim"=2206000000.0, "imag / resp"=-3.3154297}, {"real / stim"=2207531250.0, "imag / resp"=-3.3165283}, {"real / stim"=2209062500.0, "imag / resp"=-3.310669}, {"real / stim"=2210593750.0, "imag / resp"=-3.3114014}, {"real / stim"=2212125000.0, "imag / resp"=-3.3067627}, {"real / stim"=2213656250.0, "imag / resp"=-3.307373}, {"real / stim"=2215187500.0, "imag / resp"=-3.2988281}, {"real / stim"=2216718750.0, "imag / resp"=-3.3006592}, {"real / stim"=2218250000.0, "imag / resp"=-3.2982178}, {"real / stim"=2219781250.0, "imag / resp"=-3.2922363}, {"real / stim"=2221312500.0, "imag / resp"=-3.2929688}, {"real / stim"=2222843750.0, "imag / resp"=-3.288086}, {"real / stim"=2224375000.0, "imag / resp"=-3.2839355}, {"real / stim"=2225906250.0, "imag / resp"=-3.284912}, {"real / stim"=2227437500.0, "imag / resp"=-3.281372}, {"real / stim"=2228968750.0, "imag / resp"=-3.2757568}, {"real / stim"=2230500000.0, "imag / resp"=-3.2767334}, {"real / stim"=2232031250.0, "imag / resp"=-3.269165}, {"real / stim"=2233562500.0, "imag / resp"=-3.270752}, {"real / stim"=2235093750.0, "imag / resp"=-3.2653809}, {"real / stim"=2236625000.0, "imag / resp"=-3.2624512}, {"real / stim"=2238156250.0, "imag / resp"=-3.260376}, {"real / stim"=2239687500.0, "imag / resp"=-3.251831}, {"real / stim"=2241218750.0, "imag / resp"=-3.2508545}, {"real / stim"=2242750000.0, "imag / resp"=-3.2487793}, {"real / stim"=2244281250.0, "imag / resp"=-3.2388916}, {"real / stim"=2245812500.0, "imag / resp"=-3.23938}, {"real / stim"=2247343750.0, "imag / resp"=-3.2299805}, {"real / stim"=2248875000.0, "imag / resp"=-3.2282715}, {"real / stim"=2250406250.0, "imag / resp"=-3.220581}, {"real / stim"=2251937500.0, "imag / resp"=-3.2132568}, {"real / stim"=2253468750.0, "imag / resp"=-3.210205}, {"real / stim"=2255000000.0, "imag / resp"=-3.203247}, {"real / stim"=2256531250.0, "imag / resp"=-3.1948242}, {"real / stim"=2258062500.0, "imag / resp"=-3.1879883}, {"real / stim"=2259593750.0, "imag / resp"=-3.1833496}, {"real / stim"=2261125000.0, "imag / resp"=-3.1776123}, {"real / stim"=2262656250.0, "imag / resp"=-3.1693115}, {"real / stim"=2264187500.0, "imag / resp"=-3.1639404}, {"real / stim"=2265718750.0, "imag / resp"=-3.158081}, {"real / stim"=2267250000.0, "imag / resp"=-3.1452637}, {"real / stim"=2268781250.0, "imag / resp"=-3.1385498}, {"real / stim"=2270312500.0, "imag / resp"=-3.1365967}, {"real / stim"=2271843750.0, "imag / resp"=-3.128662}, {"real / stim"=2273375000.0, "imag / resp"=-3.1271973}, {"real / stim"=2274906250.0, "imag / resp"=-3.1209717}, {"real / stim"=2276437500.0, "imag / resp"=-3.116333}, {"real / stim"=2277968750.0, "imag / resp"=-3.1157227}, {"real / stim"=2279500000.0, "imag / resp"=-3.107666}, {"real / stim"=2281031250.0, "imag / resp"=-3.106079}, {"real / stim"=2282562500.0, "imag / resp"=-3.0980225}, {"real / stim"=2284093750.0, "imag / resp"=-3.1026611}, {"real / stim"=2285625000.0, "imag / resp"=-3.0979004}, {"real / stim"=2287156250.0, "imag / resp"=-3.0998535}, {"real / stim"=2288687500.0, "imag / resp"=-3.0981445}, {"real / stim"=2290218750.0, "imag / resp"=-3.0960693}, {"real / stim"=2291750000.0, "imag / resp"=-3.095337}, {"real / stim"=2293281250.0, "imag / resp"=-3.0957031}, {"real / stim"=2294812500.0, "imag / resp"=-3.0968018}, {"real / stim"=2296343750.0, "imag / resp"=-3.0947266}, {"real / stim"=2297875000.0, "imag / resp"=-3.0914307}, {"real / stim"=2299406250.0, "imag / resp"=-3.0926514}, {"real / stim"=2300937500.0, "imag / resp"=-3.093872}, {"real / stim"=2302468750.0, "imag / resp"=-3.0979004}, {"real / stim"=2304000000.0, "imag / resp"=-3.0931396}, {"real / stim"=2305531250.0, "imag / resp"=-3.0946045}, {"real / stim"=2307062500.0, "imag / resp"=-3.09375}, {"real / stim"=2308593750.0, "imag / resp"=-3.097412}, {"real / stim"=2310125000.0, "imag / resp"=-3.0943604}, {"real / stim"=2311656250.0, "imag / resp"=-3.1019287}, {"real / stim"=2313187500.0, "imag / resp"=-3.0994873}, {"real / stim"=2314718750.0, "imag / resp"=-3.1031494}, {"real / stim"=2316250000.0, "imag / resp"=-3.1009521}, {"real / stim"=2317781250.0, "imag / resp"=-3.1031494}, {"real / stim"=2319312500.0, "imag / resp"=-3.1064453}, {"real / stim"=2320843750.0, "imag / resp"=-3.1068115}, {"real / stim"=2322375000.0, "imag / resp"=-3.1107178}, {"real / stim"=2323906250.0, "imag / resp"=-3.1091309}, {"real / stim"=2325437500.0, "imag / resp"=-3.1120605}, {"real / stim"=2326968750.0, "imag / resp"=-3.1120605}, {"real / stim"=2328500000.0, "imag / resp"=-3.1124268}, {"real / stim"=2330031250.0, "imag / resp"=-3.1152344}, {"real / stim"=2331562500.0, "imag / resp"=-3.1101074}, {"real / stim"=2333093750.0, "imag / resp"=-3.113037}, {"real / stim"=2334625000.0, "imag / resp"=-3.1173096}, {"real / stim"=2336156250.0, "imag / resp"=-3.1192627}, {"real / stim"=2337687500.0, "imag / resp"=-3.1157227}, {"real / stim"=2339218750.0, "imag / resp"=-3.1165771}, {"real / stim"=2340750000.0, "imag / resp"=-3.1160889}, {"real / stim"=2342281250.0, "imag / resp"=-3.1118164}, {"real / stim"=2343812500.0, "imag / resp"=-3.1114502}, {"real / stim"=2345343750.0, "imag / resp"=-3.1108398}, {"real / stim"=2346875000.0, "imag / resp"=-3.1037598}, {"real / stim"=2348406250.0, "imag / resp"=-3.0998535}, {"real / stim"=2349937500.0, "imag / resp"=-3.098999}, {"real / stim"=2351468750.0, "imag / resp"=-3.0914307}, {"real / stim"=2353000000.0, "imag / resp"=-3.0875244}, {"real / stim"=2354531250.0, "imag / resp"=-3.081421}, {"real / stim"=2356062500.0, "imag / resp"=-3.0734863}, {"real / stim"=2357593750.0, "imag / resp"=-3.069336}, {"real / stim"=2359125000.0, "imag / resp"=-3.0598145}, {"real / stim"=2360656250.0, "imag / resp"=-3.0541992}, {"real / stim"=2362187500.0, "imag / resp"=-3.0496826}, {"real / stim"=2363718750.0, "imag / resp"=-3.0427246}, {"real / stim"=2365250000.0, "imag / resp"=-3.0343018}, {"real / stim"=2366781250.0, "imag / resp"=-3.0245361}, {"real / stim"=2368312500.0, "imag / resp"=-3.0179443}, {"real / stim"=2369843750.0, "imag / resp"=-3.0126953}, {"real / stim"=2371375000.0, "imag / resp"=-3.0056152}, {"real / stim"=2372906250.0, "imag / resp"=-3.0007324}, {"real / stim"=2374437500.0, "imag / resp"=-2.9925537}, {"real / stim"=2375968750.0, "imag / resp"=-2.984253}, {"real / stim"=2377500000.0, "imag / resp"=-2.9816895}, {"real / stim"=2379031250.0, "imag / resp"=-2.9752197}, {"real / stim"=2380562500.0, "imag / resp"=-2.96875}, {"real / stim"=2382093750.0, "imag / resp"=-2.9677734}, {"real / stim"=2383625000.0, "imag / resp"=-2.9610596}, {"real / stim"=2385156250.0, "imag / resp"=-2.9559326}, {"real / stim"=2386687500.0, "imag / resp"=-2.9537354}, {"real / stim"=2388218750.0, "imag / resp"=-2.9473877}, {"real / stim"=2389750000.0, "imag / resp"=-2.9467773}, {"real / stim"=2391281250.0, "imag / resp"=-2.9448242}, {"real / stim"=2392812500.0, "imag / resp"=-2.9434814}, {"real / stim"=2394343750.0, "imag / resp"=-2.942627}, {"real / stim"=2395875000.0, "imag / resp"=-2.9398193}, {"real / stim"=2397406250.0, "imag / resp"=-2.9399414}, {"real / stim"=2398937500.0, "imag / resp"=-2.9383545}, {"real / stim"=2400468750.0, "imag / resp"=-2.9383545}, {"real / stim"=2402000000.0, "imag / resp"=-2.9348145}, {"real / stim"=2403531250.0, "imag / resp"=-2.9333496}, {"real / stim"=2405062500.0, "imag / resp"=-2.9345703}, {"real / stim"=2406593750.0, "imag / resp"=-2.9326172}, {"real / stim"=2408125000.0, "imag / resp"=-2.9331055}, {"real / stim"=2409656250.0, "imag / resp"=-2.932495}, {"real / stim"=2411187500.0, "imag / resp"=-2.9333496}, {"real / stim"=2412718750.0, "imag / resp"=-2.93042}, {"real / stim"=2414250000.0, "imag / resp"=-2.928955}, {"real / stim"=2415781250.0, "imag / resp"=-2.9348145}, {"real / stim"=2417312500.0, "imag / resp"=-2.9331055}, {"real / stim"=2418843750.0, "imag / resp"=-2.9351807}, {"real / stim"=2420375000.0, "imag / resp"=-2.9399414}, {"real / stim"=2421906250.0, "imag / resp"=-2.9355469}, {"real / stim"=2423437500.0, "imag / resp"=-2.9403076}, {"real / stim"=2424968750.0, "imag / resp"=-2.9415283}, {"real / stim"=2426500000.0, "imag / resp"=-2.9486084}, {"real / stim"=2428031250.0, "imag / resp"=-2.9442139}, {"real / stim"=2429562500.0, "imag / resp"=-2.947754}, {"real / stim"=2431093750.0, "imag / resp"=-2.9526367}, {"real / stim"=2432625000.0, "imag / resp"=-2.9527588}, {"real / stim"=2434156250.0, "imag / resp"=-2.9598389}, {"real / stim"=2435687500.0, "imag / resp"=-2.9631348}, {"real / stim"=2437218750.0, "imag / resp"=-2.9625244}, {"real / stim"=2438750000.0, "imag / resp"=-2.9655762}, {"real / stim"=2440281250.0, "imag / resp"=-2.9666748}, {"real / stim"=2441812500.0, "imag / resp"=-2.9693604}, {"real / stim"=2443343750.0, "imag / resp"=-2.97229}, {"real / stim"=2444875000.0, "imag / resp"=-2.9708252}, {"real / stim"=2446406250.0, "imag / resp"=-2.9694824}, {"real / stim"=2447937500.0, "imag / resp"=-2.9716797}, {"real / stim"=2449468750.0, "imag / resp"=-2.9696045}, {"real / stim"=2451000000.0, "imag / resp"=-2.968872}, {"real / stim"=2452531250.0, "imag / resp"=-2.9713135}, {"real / stim"=2454062500.0, "imag / resp"=-2.9680176}, {"real / stim"=2455593750.0, "imag / resp"=-2.9641113}, {"real / stim"=2457125000.0, "imag / resp"=-2.9631348}, {"real / stim"=2458656250.0, "imag / resp"=-2.9575195}, {"real / stim"=2460187500.0, "imag / resp"=-2.9555664}, {"real / stim"=2461718750.0, "imag / resp"=-2.9476318}, {"real / stim"=2463250000.0, "imag / resp"=-2.9436035}, {"real / stim"=2464781250.0, "imag / resp"=-2.937378}, {"real / stim"=2466312500.0, "imag / resp"=-2.9344482}, {"real / stim"=2467843750.0, "imag / resp"=-2.9240723}, {"real / stim"=2469375000.0, "imag / resp"=-2.920288}, {"real / stim"=2470906250.0, "imag / resp"=-2.9102783}, {"real / stim"=2472437500.0, "imag / resp"=-2.904419}, {"real / stim"=2473968750.0, "imag / resp"=-2.9005127}, {"real / stim"=2475500000.0, "imag / resp"=-2.8952637}, {"real / stim"=2477031250.0, "imag / resp"=-2.8848877}, {"real / stim"=2478562500.0, "imag / resp"=-2.878662}, {"real / stim"=2480093750.0, "imag / resp"=-2.8737793}, {"real / stim"=2481625000.0, "imag / resp"=-2.866455}, {"real / stim"=2483156250.0, "imag / resp"=-2.8590088}, {"real / stim"=2484687500.0, "imag / resp"=-2.8555908}, {"real / stim"=2486218750.0, "imag / resp"=-2.854004}, {"real / stim"=2487750000.0, "imag / resp"=-2.8486328}, {"real / stim"=2489281250.0, "imag / resp"=-2.84375}, {"real / stim"=2490812500.0, "imag / resp"=-2.8417969}, {"real / stim"=2492343750.0, "imag / resp"=-2.838745}, {"real / stim"=2493875000.0, "imag / resp"=-2.8371582}, {"real / stim"=2495406250.0, "imag / resp"=-2.8336182}, {"real / stim"=2496937500.0, "imag / resp"=-2.83313}, {"real / stim"=2498468750.0, "imag / resp"=-2.8311768}, {"real / stim"=2500000000.0, "imag / resp"=-2.8309326}] {"imag / resp" format="%.4e"; "real / stim" format="%.4e"}, 2 "graphical display":cluster{dbl, dbl}[](graph)=[{50000000.0, -3.442138671875}, {51531250.0, -3.4520263671875}, {53062500.0, -3.460205078125}, {54593750.0, -3.4654541015625}, {56125000.0, -3.4788818359375}, {57656250.0, -3.4852294921875}, {59187500.0, -3.493408203125}, {60718750.0, -3.5015869140625}, {62250000.0, -3.50732421875}, {63781250.0, -3.515869140625}, {65312500.0, -3.5167236328125}, {66843750.0, -3.5233154296875}, {68375000.0, -3.530517578125}, {69906250.0, -3.5341796875}, {71437500.0, -3.5355224609375}, {72968750.0, -3.5379638671875}, {74500000.0, -3.538330078125}, {76031250.0, -3.54052734375}, {77562500.0, -3.5399169921875}, {79093750.0, -3.53955078125}, {80625000.0, -3.5390625}, {82156250.0, -3.538330078125}, {83687500.0, -3.5364990234375}, {85218750.0, -3.5343017578125}, {86750000.0, -3.5347900390625}, {88281250.0, -3.5333251953125}, {89812500.0, -3.531005859375}, {91343750.0, -3.533935546875}, {92875000.0, -3.531982421875}, {94406250.0, -3.5347900390625}, {95937500.0, -3.534423828125}, {97468750.0, -3.5341796875}, {99000000.0, -3.5372314453125}, {100531250.0, -3.5399169921875}, {102062500.0, -3.5408935546875}, {103593750.0, -3.5462646484375}, {105125000.0, -3.5487060546875}, {106656250.0, -3.553466796875}, {108187500.0, -3.5574951171875}, {109718750.0, -3.5615234375}, {111250000.0, -3.56787109375}, {112781250.0, -3.575439453125}, {114312500.0, -3.578125}, {115843750.0, -3.5867919921875}, {117375000.0, -3.587890625}, {118906250.0, -3.5941162109375}, {120437500.0, -3.6007080078125}, {121968750.0, -3.6297607421875}, {123500000.0, -3.6346435546875}, {125031250.0, -3.6373291015625}, {126562500.0, -3.6402587890625}, {128093750.0, -3.64306640625}, {129625000.0, -3.6451416015625}, {131156250.0, -3.6461181640625}, {132687500.0, -3.6494140625}, {134218750.0, -3.6500244140625}, {135750000.0, -3.65087890625}, {137281250.0, -3.6494140625}, {138812500.0, -3.6502685546875}, {140343750.0, -3.650146484375}, {141875000.0, -3.64990234375}, {143406250.0, -3.6488037109375}, {144937500.0, -3.6505126953125}, {146468750.0, -3.6458740234375}, {148000000.0, -3.6451416015625}, {149531250.0, -3.6470947265625}, {151062500.0, -3.6475830078125}, {152593750.0, -3.6475830078125}, {154125000.0, -3.6468505859375}, {155656250.0, -3.6461181640625}, {157187500.0, -3.6483154296875}, {158718750.0, -3.64794921875}, {160250000.0, -3.6478271484375}, {161781250.0, -3.6495361328125}, {163312500.0, -3.6474609375}, {164843750.0, -3.646728515625}, {166375000.0, -3.6429443359375}, {167906250.0, -3.640380859375}, {169437500.0, -3.6375732421875}, {170968750.0, -3.633056640625}, {172500000.0, -3.6282958984375}, {174031250.0, -3.6224365234375}, {175562500.0, -3.61669921875}, {177093750.0, -3.6138916015625}, {178625000.0, -3.605712890625}, {180156250.0, -3.601806640625}, {181687500.0, -3.59521484375}, {183218750.0, -3.5897216796875}, {184750000.0, -3.5885009765625}, {186281250.0, -3.582275390625}, {187812500.0, -3.5819091796875}, {189343750.0, -3.5794677734375}, {190875000.0, -3.57666015625}, {192406250.0, -3.57373046875}, {193937500.0, -3.5733642578125}, {195468750.0, -3.5751953125}, {197000000.0, -3.57373046875}, {198531250.0, -3.5755615234375}, {200062500.0, -3.5767822265625}, {201593750.0, -3.580078125}, {203125000.0, -3.5819091796875}, {204656250.0, -3.591796875}, {206187500.0, -3.5958251953125}, {207718750.0, -3.603515625}, {209250000.0, -3.611083984375}, {210781250.0, -3.6195068359375}, {212312500.0, -3.6246337890625}, {213843750.0, -3.636474609375}, {215375000.0, -3.64501953125}, {216906250.0, -3.6513671875}, {218437500.0, -3.6573486328125}, {219968750.0, -3.664794921875}, {221500000.0, -3.6678466796875}, {223031250.0, -3.6729736328125}, {224562500.0, -3.6712646484375}, {226093750.0, -3.6702880859375}, {227625000.0, -3.6666259765625}, {229156250.0, -3.66357421875}, {230687500.0, -3.6578369140625}, {232218750.0, -3.6553955078125}, {233750000.0, -3.648193359375}, {235281250.0, -3.6396484375}, {236812500.0, -3.6318359375}, {238343750.0, -3.6229248046875}, {239875000.0, -3.61669921875}, {241406250.0, -3.60791015625}, {242937500.0, -3.602294921875}, {244468750.0, -3.5928955078125}, {246000000.0, -3.5859375}, {247531250.0, -3.5797119140625}, {249062500.0, -3.572021484375}, {250593750.0, -3.5701904296875}, {252125000.0, -3.56787109375}, {253656250.0, -3.5640869140625}, {255187500.0, -3.5595703125}, {256718750.0, -3.5560302734375}, {258250000.0, -3.5516357421875}, {259781250.0, -3.548828125}, {261312500.0, -3.5445556640625}, {262843750.0, -3.5452880859375}, {264375000.0, -3.5416259765625}, {265906250.0, -3.5411376953125}, {267437500.0, -3.5386962890625}, {268968750.0, -3.53271484375}, {270500000.0, -3.529541015625}, {272031250.0, -3.525634765625}, {273562500.0, -3.521240234375}, {275093750.0, -3.515380859375}, {276625000.0, -3.5135498046875}, {278156250.0, -3.5101318359375}, {279687500.0, -3.5045166015625}, {281218750.0, -3.5035400390625}, {282750000.0, -3.50146484375}, {284281250.0, -3.4952392578125}, {285812500.0, -3.49609375}, {287343750.0, -3.4942626953125}, {288875000.0, -3.4920654296875}, {290406250.0, -3.4903564453125}, {291937500.0, -3.4906005859375}, {293468750.0, -3.4930419921875}, {295000000.0, -3.4952392578125}, {296531250.0, -3.49658203125}, {298062500.0, -3.5}, {299593750.0, -3.5042724609375}, {301125000.0, -3.5093994140625}, {302656250.0, -3.5155029296875}, {304187500.0, -3.522216796875}, {305718750.0, -3.5230712890625}, {307250000.0, -3.53173828125}, {308781250.0, -3.5350341796875}, {310312500.0, -3.5384521484375}, {311843750.0, -3.541015625}, {313375000.0, -3.5408935546875}, {314906250.0, -3.5386962890625}, {316437500.0, -3.5364990234375}, {317968750.0, -3.53173828125}, {319500000.0, -3.523193359375}, {321031250.0, -3.5150146484375}, {322562500.0, -3.5029296875}, {324093750.0, -3.4937744140625}, {325625000.0, -3.4818115234375}, {327156250.0, -3.468505859375}, {328687500.0, -3.4542236328125}, {330218750.0, -3.439697265625}, {331750000.0, -3.4239501953125}, {333281250.0, -3.4139404296875}, {334812500.0, -3.398193359375}, {336343750.0, -3.38916015625}, {337875000.0, -3.3780517578125}, {339406250.0, -3.36767578125}, {340937500.0, -3.3592529296875}, {342468750.0, -3.348876953125}, {344000000.0, -3.3426513671875}, {345531250.0, -3.336181640625}, {347062500.0, -3.3267822265625}, {348593750.0, -3.320068359375}, {350125000.0, -3.314208984375}, {351656250.0, -3.3060302734375}, {353187500.0, -3.2999267578125}, {354718750.0, -3.29248046875}, {356250000.0, -3.287841796875}, {357781250.0, -3.28271484375}, {359312500.0, -3.275634765625}, {360843750.0, -3.2689208984375}, {362375000.0, -3.2657470703125}, {363906250.0, -3.2613525390625}, {365437500.0, -3.256103515625}, {366968750.0, -3.248291015625}, {368500000.0, -3.2403564453125}, {370031250.0, -3.23876953125}, {371562500.0, -3.2325439453125}, {373093750.0, -3.222900390625}, {374625000.0, -3.221923828125}, {376156250.0, -3.21337890625}, {377687500.0, -3.2088623046875}, {379218750.0, -3.2069091796875}, {380750000.0, -3.2022705078125}, {382281250.0, -3.197998046875}, {383812500.0, -3.1929931640625}, {385343750.0, -3.186767578125}, {386875000.0, -3.1846923828125}, {388406250.0, -3.1822509765625}, {389937500.0, -3.17236328125}, {391468750.0, -3.1693115234375}, {393000000.0, -3.161865234375}, {394531250.0, -3.158203125}, {396062500.0, -3.151123046875}, {397593750.0, -3.1497802734375}, {399125000.0, -3.1468505859375}, {400656250.0, -3.142333984375}, {402187500.0, -3.14013671875}, {403718750.0, -3.135009765625}, {405250000.0, -3.1322021484375}, {406781250.0, -3.1287841796875}, {408312500.0, -3.126953125}, {409843750.0, -3.1207275390625}, {411375000.0, -3.1124267578125}, {412906250.0, -3.1092529296875}, {414437500.0, -3.1004638671875}, {415968750.0, -3.09423828125}, {417500000.0, -3.0867919921875}, {419031250.0, -3.0787353515625}, {420562500.0, -3.0712890625}, {422093750.0, -3.0628662109375}, {423625000.0, -3.0609130859375}, {425156250.0, -3.04931640625}, {426687500.0, -3.04638671875}, {428218750.0, -3.0390625}, {429750000.0, -3.0340576171875}, {431281250.0, -3.0281982421875}, {432812500.0, -3.020751953125}, {434343750.0, -3.010986328125}, {435875000.0, -3.0072021484375}, {437406250.0, -3.00390625}, {438937500.0, -2.9969482421875}, {440468750.0, -2.994873046875}, {442000000.0, -2.9940185546875}, {443531250.0, -2.98681640625}, {445062500.0, -2.98291015625}, {446593750.0, -2.9801025390625}, {448125000.0, -2.978271484375}, {449656250.0, -2.979248046875}, {451187500.0, -2.9776611328125}, {452718750.0, -2.976806640625}, {454250000.0, -2.975830078125}, {455781250.0, -2.9755859375}, {457312500.0, -2.97314453125}, {458843750.0, -2.96728515625}, {460375000.0, -2.96337890625}, {461906250.0, -2.96142578125}, {463437500.0, -2.9541015625}, {464968750.0, -2.947998046875}, {466500000.0, -2.9390869140625}, {468031250.0, -2.9306640625}, {469562500.0, -2.9232177734375}, {471093750.0, -2.916015625}, {472625000.0, -2.908447265625}, {474156250.0, -2.8984375}, {475687500.0, -2.889404296875}, {477218750.0, -2.8780517578125}, {478750000.0, -2.8714599609375}, {480281250.0, -2.8629150390625}, {481812500.0, -2.8583984375}, {483343750.0, -2.8497314453125}, {484875000.0, -2.8443603515625}, {486406250.0, -2.837890625}, {487937500.0, -2.83349609375}, {489468750.0, -2.8250732421875}, {491000000.0, -2.826416015625}, {492531250.0, -2.8209228515625}, {494062500.0, -2.8170166015625}, {495593750.0, -2.8131103515625}, {497125000.0, -2.812744140625}, {498656250.0, -2.8111572265625}, {500187500.0, -2.8095703125}, {501718750.0, -2.8087158203125}, {503250000.0, -2.80517578125}, {504781250.0, -2.8004150390625}, {506312500.0, -2.79833984375}, {507843750.0, -2.800537109375}, {509375000.0, -2.7972412109375}, {510906250.0, -2.7955322265625}, {512437500.0, -2.789306640625}, {513968750.0, -2.789794921875}, {515500000.0, -2.783447265625}, {517031250.0, -2.779541015625}, {518562500.0, -2.7781982421875}, {520093750.0, -2.77587890625}, {521625000.0, -2.77294921875}, {523156250.0, -2.7708740234375}, {524687500.0, -2.7645263671875}, {526218750.0, -2.7635498046875}, {527750000.0, -2.7574462890625}, {529281250.0, -2.755859375}, {530812500.0, -2.75439453125}, {532343750.0, -2.7503662109375}, {533875000.0, -2.7474365234375}, {535406250.0, -2.7425537109375}, {536937500.0, -2.7371826171875}, {538468750.0, -2.73681640625}, {540000000.0, -2.733642578125}, {541531250.0, -2.7313232421875}, {543062500.0, -2.7293701171875}, {544593750.0, -2.7286376953125}, {546125000.0, -2.7264404296875}, {547656250.0, -2.72314453125}, {549187500.0, -2.7215576171875}, {550718750.0, -2.71875}, {552250000.0, -2.72021484375}, {553781250.0, -2.71630859375}, {555312500.0, -2.715576171875}, {556843750.0, -2.712158203125}, {558375000.0, -2.7099609375}, {559906250.0, -2.7099609375}, {561437500.0, -2.7073974609375}, {562968750.0, -2.7020263671875}, {564500000.0, -2.701416015625}, {566031250.0, -2.6993408203125}, {567562500.0, -2.6949462890625}, {569093750.0, -2.6939697265625}, {570625000.0, -2.6903076171875}, {572156250.0, -2.6895751953125}, {573687500.0, -2.6875}, {575218750.0, -2.68408203125}, {576750000.0, -2.684326171875}, {578281250.0, -2.6846923828125}, {579812500.0, -2.6829833984375}, {581343750.0, -2.6826171875}, {582875000.0, -2.6817626953125}, {584406250.0, -2.68408203125}, {585937500.0, -2.68115234375}, {587468750.0, -2.683837890625}, {589000000.0, -2.6856689453125}, {590531250.0, -2.685302734375}, {592062500.0, -2.6868896484375}, {593593750.0, -2.690673828125}, {595125000.0, -2.69140625}, {596656250.0, -2.6934814453125}, {598187500.0, -2.6942138671875}, {599718750.0, -2.6964111328125}, {601250000.0, -2.702392578125}, {602781250.0, -2.703857421875}, {604312500.0, -2.701904296875}, {605843750.0, -2.705322265625}, {607375000.0, -2.7088623046875}, {608906250.0, -2.7130126953125}, {610437500.0, -2.7135009765625}, {611968750.0, -2.7181396484375}, {613500000.0, -2.72314453125}, {615031250.0, -2.72265625}, {616562500.0, -2.726318359375}, {618093750.0, -2.728515625}, {619625000.0, -2.7320556640625}, {621156250.0, -2.7327880859375}, {622687500.0, -2.737548828125}, {624218750.0, -2.7432861328125}, {625750000.0, -2.7454833984375}, {627281250.0, -2.748779296875}, {628812500.0, -2.7545166015625}, {630343750.0, -2.7589111328125}, {631875000.0, -2.7633056640625}, {633406250.0, -2.7698974609375}, {634937500.0, -2.7734375}, {636468750.0, -2.7840576171875}, {638000000.0, -2.7890625}, {639531250.0, -2.7982177734375}, {641062500.0, -2.80517578125}, {642593750.0, -2.8135986328125}, {644125000.0, -2.8193359375}, {645656250.0, -2.8310546875}, {647187500.0, -2.8365478515625}, {648718750.0, -2.8505859375}, {650250000.0, -2.8575439453125}, {651781250.0, -2.8662109375}, {653312500.0, -2.8760986328125}, {654843750.0, -2.888427734375}, {656375000.0, -2.90087890625}, {657906250.0, -2.91064453125}, {659437500.0, -2.9228515625}, {660968750.0, -2.9395751953125}, {662500000.0, -2.951416015625}, {664031250.0, -2.9677734375}, {665562500.0, -2.981689453125}, {667093750.0, -2.99853515625}, {668625000.0, -3.0142822265625}, {670156250.0, -3.03369140625}, {671687500.0, -3.05322265625}, {673218750.0, -3.0703125}, {674750000.0, -3.09423828125}, {676281250.0, -3.1136474609375}, {677812500.0, -3.138427734375}, {679343750.0, -3.165771484375}, {680875000.0, -3.1912841796875}, {682406250.0, -3.2218017578125}, {683937500.0, -3.24853515625}, {685468750.0, -3.2784423828125}, {687000000.0, -3.3138427734375}, {688531250.0, -3.3453369140625}, {690062500.0, -3.3814697265625}, {691593750.0, -3.41845703125}, {693125000.0, -3.453857421875}, {694656250.0, -3.4940185546875}, {696187500.0, -3.5374755859375}, {697718750.0, -3.579833984375}, {699250000.0, -3.6197509765625}, {700781250.0, -3.6650390625}, {702312500.0, -3.708740234375}, {703843750.0, -3.7529296875}, {705375000.0, -3.796875}, {706906250.0, -3.8438720703125}, {708437500.0, -3.8878173828125}, {709968750.0, -3.9287109375}, {711500000.0, -3.9735107421875}, {713031250.0, -4.01171875}, {714562500.0, -4.049560546875}, {716093750.0, -4.086669921875}, {717625000.0, -4.12109375}, {719156250.0, -4.15087890625}, {720687500.0, -4.178955078125}, {722218750.0, -4.200927734375}, {723750000.0, -4.220458984375}, {725281250.0, -4.237060546875}, {726812500.0, -4.2470703125}, {728343750.0, -4.2509765625}, {729875000.0, -4.253173828125}, {731406250.0, -4.248779296875}, {732937500.0, -4.238037109375}, {734468750.0, -4.22509765625}, {736000000.0, -4.210693359375}, {737531250.0, -4.1884765625}, {739062500.0, -4.166748046875}, {740593750.0, -4.1474609375}, {742125000.0, -4.116455078125}, {743656250.0, -4.091552734375}, {745187500.0, -4.06591796875}, {746718750.0, -4.033203125}, {748250000.0, -4.008056640625}, {749781250.0, -3.98193359375}, {751312500.0, -3.9525146484375}, {752843750.0, -3.9273681640625}, {754375000.0, -3.9002685546875}, {755906250.0, -3.87548828125}, {757437500.0, -3.849609375}, {758968750.0, -3.8243408203125}, {760500000.0, -3.8017578125}, {762031250.0, -3.7774658203125}, {763562500.0, -3.7528076171875}, {765093750.0, -3.7271728515625}, {766625000.0, -3.7041015625}, {768156250.0, -3.681640625}, {769687500.0, -3.6595458984375}, {771218750.0, -3.6368408203125}, {772750000.0, -3.6119384765625}, {774281250.0, -3.5906982421875}, {775812500.0, -3.5682373046875}, {777343750.0, -3.5469970703125}, {778875000.0, -3.525634765625}, {780406250.0, -3.50390625}, {781937500.0, -3.4840087890625}, {783468750.0, -3.4656982421875}, {785000000.0, -3.4483642578125}, {786531250.0, -3.43212890625}, {788062500.0, -3.4139404296875}, {789593750.0, -3.400634765625}, {791125000.0, -3.38623046875}, {792656250.0, -3.3748779296875}, {794187500.0, -3.3626708984375}, {795718750.0, -3.3515625}, {797250000.0, -3.341064453125}, {798781250.0, -3.33056640625}, {800312500.0, -3.3204345703125}, {801843750.0, -3.3148193359375}, {803375000.0, -3.3074951171875}, {804906250.0, -3.3006591796875}, {806437500.0, -3.2933349609375}, {807968750.0, -3.2864990234375}, {809500000.0, -3.27978515625}, {811031250.0, -3.273681640625}, {812562500.0, -3.2696533203125}, {814093750.0, -3.2633056640625}, {815625000.0, -3.2550048828125}, {817156250.0, -3.250732421875}, {818687500.0, -3.248291015625}, {820218750.0, -3.2412109375}, {821750000.0, -3.2398681640625}, {823281250.0, -3.2357177734375}, {824812500.0, -3.2305908203125}, {826343750.0, -3.2257080078125}, {827875000.0, -3.2196044921875}, {829406250.0, -3.218017578125}, {830937500.0, -3.21435546875}, {832468750.0, -3.208251953125}, {834000000.0, -3.20751953125}, {835531250.0, -3.2010498046875}, {837062500.0, -3.1973876953125}, {838593750.0, -3.196533203125}, {840125000.0, -3.1904296875}, {841656250.0, -3.18701171875}, {843187500.0, -3.1846923828125}, {844718750.0, -3.181396484375}, {846250000.0, -3.17724609375}, {847781250.0, -3.17626953125}, {849312500.0, -3.171142578125}, {850843750.0, -3.171142578125}, {852375000.0, -3.168212890625}, {853906250.0, -3.164306640625}, {855437500.0, -3.16064453125}, {856968750.0, -3.1583251953125}, {858500000.0, -3.153076171875}, {860031250.0, -3.148193359375}, {861562500.0, -3.142822265625}, {863093750.0, -3.1376953125}, {864625000.0, -3.13671875}, {866156250.0, -3.1328125}, {867687500.0, -3.131591796875}, {869218750.0, -3.1312255859375}, {870750000.0, -3.12744140625}, {872281250.0, -3.1226806640625}, {873812500.0, -3.123779296875}, {875343750.0, -3.12353515625}, {876875000.0, -3.122802734375}, {878406250.0, -3.120849609375}, {879937500.0, -3.12060546875}, {881468750.0, -3.121826171875}, {883000000.0, -3.1241455078125}, {884531250.0, -3.125732421875}, {886062500.0, -3.129150390625}, {887593750.0, -3.126708984375}, {889125000.0, -3.1326904296875}, {890656250.0, -3.134521484375}, {892187500.0, -3.1363525390625}, {893718750.0, -3.1424560546875}, {895250000.0, -3.1439208984375}, {896781250.0, -3.146728515625}, {898312500.0, -3.151123046875}, {899843750.0, -3.1544189453125}, {901375000.0, -3.1571044921875}, {902906250.0, -3.1629638671875}, {904437500.0, -3.163818359375}, {905968750.0, -3.16845703125}, {907500000.0, -3.171630859375}, {909031250.0, -3.175048828125}, {910562500.0, -3.181640625}, {912093750.0, -3.1827392578125}, {913625000.0, -3.186279296875}, {915156250.0, -3.1881103515625}, {916687500.0, -3.190185546875}, {918218750.0, -3.19482421875}, {919750000.0, -3.1934814453125}, {921281250.0, -3.1986083984375}, {922812500.0, -3.1998291015625}, {924343750.0, -3.203857421875}, {925875000.0, -3.20556640625}, {927406250.0, -3.2066650390625}, {928937500.0, -3.208740234375}, {930468750.0, -3.212646484375}, {932000000.0, -3.2144775390625}, {933531250.0, -3.2117919921875}, {935062500.0, -3.21630859375}, {936593750.0, -3.21728515625}, {938125000.0, -3.2183837890625}, {939656250.0, -3.219482421875}, {941187500.0, -3.2210693359375}, {942718750.0, -3.2216796875}, {944250000.0, -3.2247314453125}, {945781250.0, -3.225341796875}, {947312500.0, -3.2283935546875}, {948843750.0, -3.2266845703125}, {950375000.0, -3.2281494140625}, {951906250.0, -3.227294921875}, {953437500.0, -3.22998046875}, {954968750.0, -3.2301025390625}, {956500000.0, -3.23193359375}, {958031250.0, -3.2310791015625}, {959562500.0, -3.229248046875}, {961093750.0, -3.2359619140625}, {962625000.0, -3.2352294921875}, {964156250.0, -3.2340087890625}, {965687500.0, -3.2347412109375}, {967218750.0, -3.23779296875}, {968750000.0, -3.2388916015625}, {970281250.0, -3.2403564453125}, {971812500.0, -3.241455078125}, {973343750.0, -3.2427978515625}, {974875000.0, -3.244384765625}, {976406250.0, -3.2449951171875}, {977937500.0, -3.245849609375}, {979468750.0, -3.2498779296875}, {981000000.0, -3.2520751953125}, {982531250.0, -3.2528076171875}, {984062500.0, -3.2559814453125}, {985593750.0, -3.2606201171875}, {987125000.0, -3.2652587890625}, {988656250.0, -3.2664794921875}, {990187500.0, -3.272216796875}, {991718750.0, -3.2752685546875}, {993250000.0, -3.2823486328125}, {994781250.0, -3.2877197265625}, {996312500.0, -3.29296875}, {997843750.0, -3.295654296875}, {999375000.0, -3.298095703125}, {1000906250.0, -3.305419921875}, {1002437500.0, -3.3076171875}, {1003968750.0, -3.3115234375}, {1005500000.0, -3.3162841796875}, {1007031250.0, -3.3223876953125}, {1008562500.0, -3.326416015625}, {1010093750.0, -3.33251953125}, {1011625000.0, -3.3370361328125}, {1013156250.0, -3.3406982421875}, {1014687500.0, -3.347900390625}, {1016218750.0, -3.353515625}, {1017750000.0, -3.3592529296875}, {1019281250.0, -3.364990234375}, {1020812500.0, -3.3685302734375}, {1022343750.0, -3.374267578125}, {1023875000.0, -3.37744140625}, {1025406250.0, -3.381103515625}, {1026937500.0, -3.3887939453125}, {1028468750.0, -3.39501953125}, {1030000000.0, -3.3966064453125}, {1031531250.0, -3.401123046875}, {1033062500.0, -3.4075927734375}, {1034593750.0, -3.4130859375}, {1036125000.0, -3.4200439453125}, {1037656250.0, -3.42138671875}, {1039187500.0, -3.427734375}, {1040718750.0, -3.43115234375}, {1042250000.0, -3.4342041015625}, {1043781250.0, -3.4375}, {1045312500.0, -3.4422607421875}, {1046843750.0, -3.4468994140625}, {1048375000.0, -3.4510498046875}, {1049906250.0, -3.4549560546875}, {1051437500.0, -3.45751953125}, {1052968750.0, -3.461669921875}, {1054500000.0, -3.4609375}, {1056031250.0, -3.465087890625}, {1057562500.0, -3.4649658203125}, {1059093750.0, -3.4688720703125}, {1060625000.0, -3.47216796875}, {1062156250.0, -3.474609375}, {1063687500.0, -3.47705078125}, {1065218750.0, -3.4737548828125}, {1066750000.0, -3.4766845703125}, {1068281250.0, -3.4798583984375}, {1069812500.0, -3.4810791015625}, {1071343750.0, -3.48291015625}, {1072875000.0, -3.48388671875}, {1074406250.0, -3.4837646484375}, {1075937500.0, -3.4854736328125}, {1077468750.0, -3.484130859375}, {1079000000.0, -3.4879150390625}, {1080531250.0, -3.49072265625}, {1082062500.0, -3.4937744140625}, {1083593750.0, -3.493896484375}, {1085125000.0, -3.498291015625}, {1086656250.0, -3.50390625}, {1088187500.0, -3.5086669921875}, {1089718750.0, -3.51171875}, {1091250000.0, -3.514404296875}, {1092781250.0, -3.5184326171875}, {1094312500.0, -3.5250244140625}, {1095843750.0, -3.5289306640625}, {1097375000.0, -3.536376953125}, {1098906250.0, -3.544189453125}, {1100437500.0, -3.5487060546875}, {1101968750.0, -3.55908203125}, {1103500000.0, -3.5677490234375}, {1105031250.0, -3.573974609375}, {1106562500.0, -3.582275390625}, {1108093750.0, -3.5888671875}, {1109625000.0, -3.601318359375}, {1111156250.0, -3.6058349609375}, {1112687500.0, -3.6142578125}, {1114218750.0, -3.6201171875}, {1115750000.0, -3.6317138671875}, {1117281250.0, -3.6385498046875}, {1118812500.0, -3.650146484375}, {1120343750.0, -3.6552734375}, {1121875000.0, -3.6650390625}, {1123406250.0, -3.67529296875}, {1124937500.0, -3.68310546875}, {1126468750.0, -3.69287109375}, {1128000000.0, -3.7001953125}, {1129531250.0, -3.7081298828125}, {1131062500.0, -3.7164306640625}, {1132593750.0, -3.7252197265625}, {1134125000.0, -3.730224609375}, {1135656250.0, -3.741455078125}, {1137187500.0, -3.749267578125}, {1138718750.0, -3.755615234375}, {1140250000.0, -3.761474609375}, {1141781250.0, -3.771728515625}, {1143312500.0, -3.77783203125}, {1144843750.0, -3.782470703125}, {1146375000.0, -3.7896728515625}, {1147906250.0, -3.79296875}, {1149437500.0, -3.7987060546875}, {1150968750.0, -3.80517578125}, {1152500000.0, -3.81298828125}, {1154031250.0, -3.8157958984375}, {1155562500.0, -3.822265625}, {1157093750.0, -3.822021484375}, {1158625000.0, -3.8272705078125}, {1160156250.0, -3.8314208984375}, {1161687500.0, -3.834228515625}, {1163218750.0, -3.8389892578125}, {1164750000.0, -3.845703125}, {1166281250.0, -3.84814453125}, {1167812500.0, -3.8543701171875}, {1169343750.0, -3.8603515625}, {1170875000.0, -3.861328125}, {1172406250.0, -3.87060546875}, {1173937500.0, -3.87451171875}, {1175468750.0, -3.8824462890625}, {1177000000.0, -3.88671875}, {1178531250.0, -3.8934326171875}, {1180062500.0, -3.89892578125}, {1181593750.0, -3.907958984375}, {1183125000.0, -3.917236328125}, {1184656250.0, -3.9246826171875}, {1186187500.0, -3.937255859375}, {1187718750.0, -3.9468994140625}, {1189250000.0, -3.955810546875}, {1190781250.0, -3.96923828125}, {1192312500.0, -3.980712890625}, {1193843750.0, -3.991943359375}, {1195375000.0, -4.005859375}, {1196906250.0, -4.01611328125}, {1198437500.0, -4.033447265625}, {1199968750.0, -4.045654296875}, {1201500000.0, -4.0634765625}, {1203031250.0, -4.074462890625}, {1204562500.0, -4.094482421875}, {1206093750.0, -4.110595703125}, {1207625000.0, -4.1279296875}, {1209156250.0, -4.140625}, {1210687500.0, -4.161376953125}, {1212218750.0, -4.172607421875}, {1213750000.0, -4.188232421875}, {1215281250.0, -4.2109375}, {1216812500.0, -4.224853515625}, {1218343750.0, -4.2431640625}, {1219875000.0, -4.26123046875}, {1221406250.0, -4.279541015625}, {1222937500.0, -4.298095703125}, {1224468750.0, -4.313720703125}, {1226000000.0, -4.335205078125}, {1227531250.0, -4.3525390625}, {1229062500.0, -4.371826171875}, {1230593750.0, -4.3916015625}, {1232125000.0, -4.409912109375}, {1233656250.0, -4.4306640625}, {1235187500.0, -4.451904296875}, {1236718750.0, -4.468994140625}, {1238250000.0, -4.491943359375}, {1239781250.0, -4.509765625}, {1241312500.0, -4.531982421875}, {1242843750.0, -4.55419921875}, {1244375000.0, -4.574951171875}, {1245906250.0, -4.59716796875}, {1247437500.0, -4.61865234375}, {1248968750.0, -4.639892578125}, {1250500000.0, -4.664794921875}, {1252031250.0, -4.685791015625}, {1253562500.0, -4.711669921875}, {1255093750.0, -4.731201171875}, {1256625000.0, -4.755126953125}, {1258156250.0, -4.7763671875}, {1259687500.0, -4.80322265625}, {1261218750.0, -4.82373046875}, {1262750000.0, -4.85009765625}, {1264281250.0, -4.878662109375}, {1265812500.0, -4.89892578125}, {1267343750.0, -4.92578125}, {1268875000.0, -4.951171875}, {1270406250.0, -4.979736328125}, {1271937500.0, -5.005615234375}, {1273468750.0, -5.03173828125}, {1275000000.0, -5.064208984375}, {1276531250.0, -5.090087890625}, {1278062500.0, -5.120849609375}, {1279593750.0, -5.154052734375}, {1281125000.0, -5.185302734375}, {1282656250.0, -5.2177734375}, {1284187500.0, -5.253662109375}, {1285718750.0, -5.28564453125}, {1287250000.0, -5.322509765625}, {1288781250.0, -5.36279296875}, {1290312500.0, -5.3984375}, {1291843750.0, -5.437744140625}, {1293375000.0, -5.477783203125}, {1294906250.0, -5.5166015625}, {1296437500.0, -5.561767578125}, {1297968750.0, -5.604248046875}, {1299500000.0, -5.644287109375}, {1301031250.0, -5.689697265625}, {1302562500.0, -5.734375}, {1304093750.0, -5.779296875}, {1305625000.0, -5.823974609375}, {1307156250.0, -5.8720703125}, {1308687500.0, -5.9189453125}, {1310218750.0, -5.966796875}, {1311750000.0, -6.012939453125}, {1313281250.0, -6.063232421875}, {1314812500.0, -6.1142578125}, {1316343750.0, -6.1630859375}, {1317875000.0, -6.215576171875}, {1319406250.0, -6.26513671875}, {1320937500.0, -6.315673828125}, {1322468750.0, -6.369873046875}, {1324000000.0, -6.419921875}, {1325531250.0, -6.472412109375}, {1327062500.0, -6.5244140625}, {1328593750.0, -6.58154296875}, {1330125000.0, -6.632568359375}, {1331656250.0, -6.68408203125}, {1333187500.0, -6.73974609375}, {1334718750.0, -6.793212890625}, {1336250000.0, -6.84814453125}, {1337781250.0, -6.90185546875}, {1339312500.0, -6.956787109375}, {1340843750.0, -7.01318359375}, {1342375000.0, -7.071533203125}, {1343906250.0, -7.127197265625}, {1345437500.0, -7.180419921875}, {1346968750.0, -7.236083984375}, {1348500000.0, -7.291259765625}, {1350031250.0, -7.347412109375}, {1351562500.0, -7.401611328125}, {1353093750.0, -7.455322265625}, {1354625000.0, -7.51220703125}, {1356156250.0, -7.567626953125}, {1357687500.0, -7.618408203125}, {1359218750.0, -7.671875}, {1360750000.0, -7.728271484375}, {1362281250.0, -7.783203125}, {1363812500.0, -7.83203125}, {1365343750.0, -7.8837890625}, {1366875000.0, -7.940185546875}, {1368406250.0, -7.991943359375}, {1369937500.0, -8.04443359375}, {1371468750.0, -8.09716796875}, {1373000000.0, -8.150390625}, {1374531250.0, -8.20556640625}, {1376062500.0, -8.25537109375}, {1377593750.0, -8.31298828125}, {1379125000.0, -8.36181640625}, {1380656250.0, -8.41650390625}, {1382187500.0, -8.46923828125}, {1383718750.0, -8.52197265625}, {1385250000.0, -8.57275390625}, {1386781250.0, -8.6259765625}, {1388312500.0, -8.68115234375}, {1389843750.0, -8.7314453125}, {1391375000.0, -8.7861328125}, {1392906250.0, -8.83837890625}, {1394437500.0, -8.89111328125}, {1395968750.0, -8.9384765625}, {1397500000.0, -8.9931640625}, {1399031250.0, -9.04296875}, {1400562500.0, -9.09326171875}, {1402093750.0, -9.14013671875}, {1403625000.0, -9.189453125}, {1405156250.0, -9.236328125}, {1406687500.0, -9.28125}, {1408218750.0, -9.32666015625}, {1409750000.0, -9.36865234375}, {1411281250.0, -9.412109375}, {1412812500.0, -9.45263671875}, {1414343750.0, -9.49560546875}, {1415875000.0, -9.53466796875}, {1417406250.0, -9.57275390625}, {1418937500.0, -9.60791015625}, {1420468750.0, -9.64111328125}, {1422000000.0, -9.67431640625}, {1423531250.0, -9.70361328125}, {1425062500.0, -9.73291015625}, {1426593750.0, -9.755859375}, {1428125000.0, -9.783203125}, {1429656250.0, -9.8037109375}, {1431187500.0, -9.82373046875}, {1432718750.0, -9.84521484375}, {1434250000.0, -9.85888671875}, {1435781250.0, -9.87353515625}, {1437312500.0, -9.8818359375}, {1438843750.0, -9.89208984375}, {1440375000.0, -9.8984375}, {1441906250.0, -9.90185546875}, {1443437500.0, -9.908203125}, {1444968750.0, -9.91259765625}, {1446500000.0, -9.90771484375}, {1448031250.0, -9.90478515625}, {1449562500.0, -9.9013671875}, {1451093750.0, -9.89306640625}, {1452625000.0, -9.888671875}, {1454156250.0, -9.87841796875}, {1455687500.0, -9.8720703125}, {1457218750.0, -9.85791015625}, {1458750000.0, -9.84375}, {1460281250.0, -9.83056640625}, {1461812500.0, -9.81689453125}, {1463343750.0, -9.80029296875}, {1464875000.0, -9.78369140625}, {1466406250.0, -9.765625}, {1467937500.0, -9.74560546875}, {1469468750.0, -9.72802734375}, {1471000000.0, -9.705078125}, {1472531250.0, -9.689453125}, {1474062500.0, -9.6640625}, {1475593750.0, -9.6435546875}, {1477125000.0, -9.61767578125}, {1478656250.0, -9.59619140625}, {1480187500.0, -9.568359375}, {1481718750.0, -9.54541015625}, {1483250000.0, -9.5185546875}, {1484781250.0, -9.49560546875}, {1486312500.0, -9.46435546875}, {1487843750.0, -9.43603515625}, {1489375000.0, -9.4091796875}, {1490906250.0, -9.376953125}, {1492437500.0, -9.34765625}, {1493968750.0, -9.32080078125}, {1495500000.0, -9.2900390625}, {1497031250.0, -9.25830078125}, {1498562500.0, -9.22705078125}, {1500093750.0, -9.19189453125}, {1501625000.0, -9.16259765625}, {1503156250.0, -9.12255859375}, {1504687500.0, -9.09033203125}, {1506218750.0, -9.0576171875}, {1507750000.0, -9.02392578125}, {1509281250.0, -8.98828125}, {1510812500.0, -8.94921875}, {1512343750.0, -8.9111328125}, {1513875000.0, -8.87158203125}, {1515406250.0, -8.83642578125}, {1516937500.0, -8.7958984375}, {1518468750.0, -8.76123046875}, {1520000000.0, -8.720703125}, {1521531250.0, -8.68212890625}, {1523062500.0, -8.642578125}, {1524593750.0, -8.599609375}, {1526125000.0, -8.56396484375}, {1527656250.0, -8.52001953125}, {1529187500.0, -8.48486328125}, {1530718750.0, -8.4443359375}, {1532250000.0, -8.4072265625}, {1533781250.0, -8.36376953125}, {1535312500.0, -8.32568359375}, {1536843750.0, -8.28662109375}, {1538375000.0, -8.2451171875}, {1539906250.0, -8.20947265625}, {1541437500.0, -8.17138671875}, {1542968750.0, -8.1328125}, {1544500000.0, -8.09716796875}, {1546031250.0, -8.05419921875}, {1547562500.0, -8.02197265625}, {1549093750.0, -7.983642578125}, {1550625000.0, -7.9462890625}, {1552156250.0, -7.908935546875}, {1553687500.0, -7.875}, {1555218750.0, -7.84033203125}, {1556750000.0, -7.80224609375}, {1558281250.0, -7.767822265625}, {1559812500.0, -7.73828125}, {1561343750.0, -7.70361328125}, {1562875000.0, -7.673095703125}, {1564406250.0, -7.642822265625}, {1565937500.0, -7.6064453125}, {1567468750.0, -7.5751953125}, {1569000000.0, -7.546142578125}, {1570531250.0, -7.514892578125}, {1572062500.0, -7.489013671875}, {1573593750.0, -7.4560546875}, {1575125000.0, -7.42919921875}, {1576656250.0, -7.404541015625}, {1578187500.0, -7.3759765625}, {1579718750.0, -7.348876953125}, {1581250000.0, -7.322509765625}, {1582781250.0, -7.29638671875}, {1584312500.0, -7.270751953125}, {1585843750.0, -7.240966796875}, {1587375000.0, -7.219482421875}, {1588906250.0, -7.194091796875}, {1590437500.0, -7.16796875}, {1591968750.0, -7.14501953125}, {1593500000.0, -7.119140625}, {1595031250.0, -7.095458984375}, {1596562500.0, -7.07275390625}, {1598093750.0, -7.046875}, {1599625000.0, -7.02490234375}, {1601156250.0, -7.004638671875}, {1602687500.0, -6.982177734375}, {1604218750.0, -6.96044921875}, {1605750000.0, -6.935791015625}, {1607281250.0, -6.919921875}, {1608812500.0, -6.90087890625}, {1610343750.0, -6.877685546875}, {1611875000.0, -6.858642578125}, {1613406250.0, -6.8359375}, {1614937500.0, -6.81982421875}, {1616468750.0, -6.80322265625}, {1618000000.0, -6.7802734375}, {1619531250.0, -6.766845703125}, {1621062500.0, -6.748046875}, {1622593750.0, -6.732666015625}, {1624125000.0, -6.714111328125}, {1625656250.0, -6.703857421875}, {1627187500.0, -6.686279296875}, {1628718750.0, -6.670654296875}, {1630250000.0, -6.662109375}, {1631781250.0, -6.647216796875}, {1633312500.0, -6.640380859375}, {1634843750.0, -6.625244140625}, {1636375000.0, -6.6181640625}, {1637906250.0, -6.60498046875}, {1639437500.0, -6.59912109375}, {1640968750.0, -6.589599609375}, {1642500000.0, -6.578369140625}, {1644031250.0, -6.57568359375}, {1645562500.0, -6.56689453125}, {1647093750.0, -6.56201171875}, {1648625000.0, -6.555908203125}, {1650156250.0, -6.5498046875}, {1651687500.0, -6.546875}, {1653218750.0, -6.549560546875}, {1654750000.0, -6.5458984375}, {1656281250.0, -6.54638671875}, {1657812500.0, -6.549560546875}, {1659343750.0, -6.54638671875}, {1660875000.0, -6.548828125}, {1662406250.0, -6.553466796875}, {1663937500.0, -6.558349609375}, {1665468750.0, -6.562255859375}, {1667000000.0, -6.568603515625}, {1668531250.0, -6.575439453125}, {1670062500.0, -6.581298828125}, {1671593750.0, -6.591064453125}, {1673125000.0, -6.602294921875}, {1674656250.0, -6.61181640625}, {1676187500.0, -6.62109375}, {1677718750.0, -6.633056640625}, {1679250000.0, -6.644287109375}, {1680781250.0, -6.656982421875}, {1682312500.0, -6.669921875}, {1683843750.0, -6.6845703125}, {1685375000.0, -6.700439453125}, {1686906250.0, -6.711669921875}, {1688437500.0, -6.726318359375}, {1689968750.0, -6.744140625}, {1691500000.0, -6.759521484375}, {1693031250.0, -6.775390625}, {1694562500.0, -6.79296875}, {1696093750.0, -6.809326171875}, {1697625000.0, -6.824951171875}, {1699156250.0, -6.84033203125}, {1700687500.0, -6.86083984375}, {1702218750.0, -6.87646484375}, {1703750000.0, -6.89404296875}, {1705281250.0, -6.9111328125}, {1706812500.0, -6.925537109375}, {1708343750.0, -6.942626953125}, {1709875000.0, -6.96044921875}, {1711406250.0, -6.979248046875}, {1712937500.0, -6.992919921875}, {1714468750.0, -7.0126953125}, {1716000000.0, -7.031982421875}, {1717531250.0, -7.04541015625}, {1719062500.0, -7.06201171875}, {1720593750.0, -7.080078125}, {1722125000.0, -7.093017578125}, {1723656250.0, -7.10986328125}, {1725187500.0, -7.125244140625}, {1726718750.0, -7.14013671875}, {1728250000.0, -7.156982421875}, {1729781250.0, -7.168212890625}, {1731312500.0, -7.18310546875}, {1732843750.0, -7.191162109375}, {1734375000.0, -7.20458984375}, {1735906250.0, -7.2158203125}, {1737437500.0, -7.22265625}, {1738968750.0, -7.233642578125}, {1740500000.0, -7.239990234375}, {1742031250.0, -7.2470703125}, {1743562500.0, -7.25341796875}, {1745093750.0, -7.254638671875}, {1746625000.0, -7.2578125}, {1748156250.0, -7.259033203125}, {1749687500.0, -7.261474609375}, {1751218750.0, -7.259765625}, {1752750000.0, -7.2578125}, {1754281250.0, -7.257080078125}, {1755812500.0, -7.253173828125}, {1757343750.0, -7.24658203125}, {1758875000.0, -7.24267578125}, {1760406250.0, -7.229248046875}, {1761937500.0, -7.22314453125}, {1763468750.0, -7.2099609375}, {1765000000.0, -7.197509765625}, {1766531250.0, -7.184326171875}, {1768062500.0, -7.166015625}, {1769593750.0, -7.151611328125}, {1771125000.0, -7.13330078125}, {1772656250.0, -7.115478515625}, {1774187500.0, -7.093505859375}, {1775718750.0, -7.069091796875}, {1777250000.0, -7.047607421875}, {1778781250.0, -7.02392578125}, {1780312500.0, -6.999755859375}, {1781843750.0, -6.970458984375}, {1783375000.0, -6.947998046875}, {1784906250.0, -6.914794921875}, {1786437500.0, -6.88720703125}, {1787968750.0, -6.8544921875}, {1789500000.0, -6.821044921875}, {1791031250.0, -6.792236328125}, {1792562500.0, -6.76123046875}, {1794093750.0, -6.727294921875}, {1795625000.0, -6.68896484375}, {1797156250.0, -6.652099609375}, {1798687500.0, -6.616943359375}, {1800218750.0, -6.578857421875}, {1801750000.0, -6.5400390625}, {1803281250.0, -6.501708984375}, {1804812500.0, -6.46728515625}, {1806343750.0, -6.433349609375}, {1807875000.0, -6.3916015625}, {1809406250.0, -6.353515625}, {1810937500.0, -6.3154296875}, {1812468750.0, -6.278564453125}, {1814000000.0, -6.238037109375}, {1815531250.0, -6.199462890625}, {1817062500.0, -6.159423828125}, {1818593750.0, -6.122314453125}, {1820125000.0, -6.08447265625}, {1821656250.0, -6.049560546875}, {1823187500.0, -6.01220703125}, {1824718750.0, -5.97509765625}, {1826250000.0, -5.94091796875}, {1827781250.0, -5.906982421875}, {1829312500.0, -5.866943359375}, {1830843750.0, -5.833984375}, {1832375000.0, -5.800537109375}, {1833906250.0, -5.763916015625}, {1835437500.0, -5.73193359375}, {1836968750.0, -5.696533203125}, {1838500000.0, -5.667236328125}, {1840031250.0, -5.63427734375}, {1841562500.0, -5.5986328125}, {1843093750.0, -5.56982421875}, {1844625000.0, -5.540771484375}, {1846156250.0, -5.509033203125}, {1847687500.0, -5.47265625}, {1849218750.0, -5.44580078125}, {1850750000.0, -5.413330078125}, {1852281250.0, -5.3828125}, {1853812500.0, -5.356689453125}, {1855343750.0, -5.334228515625}, {1856875000.0, -5.30712890625}, {1858406250.0, -5.282958984375}, {1859937500.0, -5.2578125}, {1861468750.0, -5.230712890625}, {1863000000.0, -5.20654296875}, {1864531250.0, -5.182373046875}, {1866062500.0, -5.1650390625}, {1867593750.0, -5.1396484375}, {1869125000.0, -5.119384765625}, {1870656250.0, -5.101318359375}, {1872187500.0, -5.083740234375}, {1873718750.0, -5.065185546875}, {1875250000.0, -5.048095703125}, {1876781250.0, -5.0302734375}, {1878312500.0, -5.014404296875}, {1879843750.0, -4.999267578125}, {1881375000.0, -4.980712890625}, {1882906250.0, -4.967041015625}, {1884437500.0, -4.949462890625}, {1885968750.0, -4.931396484375}, {1887500000.0, -4.9169921875}, {1889031250.0, -4.904052734375}, {1890562500.0, -4.888671875}, {1892093750.0, -4.87109375}, {1893625000.0, -4.858642578125}, {1895156250.0, -4.841796875}, {1896687500.0, -4.8291015625}, {1898218750.0, -4.81103515625}, {1899750000.0, -4.79833984375}, {1901281250.0, -4.783447265625}, {1902812500.0, -4.7666015625}, {1904343750.0, -4.752685546875}, {1905875000.0, -4.734619140625}, {1907406250.0, -4.720458984375}, {1908937500.0, -4.704833984375}, {1910468750.0, -4.6875}, {1912000000.0, -4.6708984375}, {1913531250.0, -4.65576171875}, {1915062500.0, -4.637939453125}, {1916593750.0, -4.625244140625}, {1918125000.0, -4.607421875}, {1919656250.0, -4.593505859375}, {1921187500.0, -4.5791015625}, {1922718750.0, -4.562255859375}, {1924250000.0, -4.546142578125}, {1925781250.0, -4.530029296875}, {1927312500.0, -4.5166015625}, {1928843750.0, -4.500732421875}, {1930375000.0, -4.48388671875}, {1931906250.0, -4.468994140625}, {1933437500.0, -4.4541015625}, {1934968750.0, -4.439453125}, {1936500000.0, -4.42529296875}, {1938031250.0, -4.41064453125}, {1939562500.0, -4.39599609375}, {1941093750.0, -4.38134765625}, {1942625000.0, -4.36572265625}, {1944156250.0, -4.3515625}, {1945687500.0, -4.338134765625}, {1947218750.0, -4.3232421875}, {1948750000.0, -4.311279296875}, {1950281250.0, -4.29833984375}, {1951812500.0, -4.283935546875}, {1953343750.0, -4.270263671875}, {1954875000.0, -4.25927734375}, {1956406250.0, -4.248779296875}, {1957937500.0, -4.23046875}, {1959468750.0, -4.22119140625}, {1961000000.0, -4.2138671875}, {1962531250.0, -4.202880859375}, {1964062500.0, -4.190185546875}, {1965593750.0, -4.17919921875}, {1967125000.0, -4.171142578125}, {1968656250.0, -4.1650390625}, {1970187500.0, -4.152587890625}, {1971718750.0, -4.147216796875}, {1973250000.0, -4.135498046875}, {1974781250.0, -4.12939453125}, {1976312500.0, -4.122802734375}, {1977843750.0, -4.119384765625}, {1979375000.0, -4.107666015625}, {1980906250.0, -4.105712890625}, {1982437500.0, -4.099853515625}, {1983968750.0, -4.090576171875}, {1985500000.0, -4.087158203125}, {1987031250.0, -4.07763671875}, {1988562500.0, -4.072998046875}, {1990093750.0, -4.06494140625}, {1991625000.0, -4.05712890625}, {1993156250.0, -4.054931640625}, {1994687500.0, -4.04736328125}, {1996218750.0, -4.04052734375}, {1997750000.0, -4.03564453125}, {1999281250.0, -4.02734375}, {2000812500.0, -4.017578125}, {2002343750.0, -4.015380859375}, {2003875000.0, -4.004638671875}, {2005406250.0, -3.999755859375}, {2006937500.0, -3.9918212890625}, {2008468750.0, -3.9862060546875}, {2010000000.0, -3.9775390625}, {2011531250.0, -3.9718017578125}, {2013062500.0, -3.9674072265625}, {2014593750.0, -3.9564208984375}, {2016125000.0, -3.947265625}, {2017656250.0, -3.9422607421875}, {2019187500.0, -3.935302734375}, {2020718750.0, -3.9287109375}, {2022250000.0, -3.9207763671875}, {2023781250.0, -3.9140625}, {2025312500.0, -3.905517578125}, {2026843750.0, -3.901123046875}, {2028375000.0, -3.89453125}, {2029906250.0, -3.8836669921875}, {2031437500.0, -3.876220703125}, {2032968750.0, -3.8707275390625}, {2034500000.0, -3.8592529296875}, {2036031250.0, -3.8570556640625}, {2037562500.0, -3.846435546875}, {2039093750.0, -3.8421630859375}, {2040625000.0, -3.8321533203125}, {2042156250.0, -3.822021484375}, {2043687500.0, -3.8175048828125}, {2045218750.0, -3.808349609375}, {2046750000.0, -3.80029296875}, {2048281250.0, -3.7906494140625}, {2049812500.0, -3.7860107421875}, {2051343750.0, -3.7747802734375}, {2052875000.0, -3.771484375}, {2054406250.0, -3.7598876953125}, {2055937500.0, -3.7537841796875}, {2057468750.0, -3.74560546875}, {2059000000.0, -3.7393798828125}, {2060531250.0, -3.73291015625}, {2062062500.0, -3.7261962890625}, {2063593750.0, -3.7203369140625}, {2065125000.0, -3.714599609375}, {2066656250.0, -3.7052001953125}, {2068187500.0, -3.7003173828125}, {2069718750.0, -3.6976318359375}, {2071250000.0, -3.69091796875}, {2072781250.0, -3.6905517578125}, {2074312500.0, -3.6849365234375}, {2075843750.0, -3.67822265625}, {2077375000.0, -3.677978515625}, {2078906250.0, -3.6756591796875}, {2080437500.0, -3.6754150390625}, {2081968750.0, -3.671142578125}, {2083500000.0, -3.6693115234375}, {2085031250.0, -3.671142578125}, {2086562500.0, -3.66259765625}, {2088093750.0, -3.6627197265625}, {2089625000.0, -3.6600341796875}, {2091156250.0, -3.6610107421875}, {2092687500.0, -3.656982421875}, {2094218750.0, -3.6514892578125}, {2095750000.0, -3.6507568359375}, {2097281250.0, -3.64501953125}, {2098812500.0, -3.640869140625}, {2100343750.0, -3.640380859375}, {2101875000.0, -3.635498046875}, {2103406250.0, -3.6292724609375}, {2104937500.0, -3.626708984375}, {2106468750.0, -3.62548828125}, {2108000000.0, -3.61669921875}, {2109531250.0, -3.6143798828125}, {2111062500.0, -3.60888671875}, {2112593750.0, -3.605224609375}, {2114125000.0, -3.597900390625}, {2115656250.0, -3.595703125}, {2117187500.0, -3.5909423828125}, {2118718750.0, -3.584716796875}, {2120250000.0, -3.5855712890625}, {2121781250.0, -3.5770263671875}, {2123312500.0, -3.576171875}, {2124843750.0, -3.5655517578125}, {2126375000.0, -3.5601806640625}, {2127906250.0, -3.556884765625}, {2129437500.0, -3.5521240234375}, {2130968750.0, -3.5465087890625}, {2132500000.0, -3.5433349609375}, {2134031250.0, -3.537109375}, {2135562500.0, -3.523681640625}, {2137093750.0, -3.51806640625}, {2138625000.0, -3.512451171875}, {2140156250.0, -3.5087890625}, {2141687500.0, -3.501953125}, {2143218750.0, -3.49658203125}, {2144750000.0, -3.4825439453125}, {2146281250.0, -3.4769287109375}, {2147812500.0, -3.4666748046875}, {2149343750.0, -3.4608154296875}, {2150875000.0, -3.453125}, {2152406250.0, -3.4439697265625}, {2153937500.0, -3.4361572265625}, {2155468750.0, -3.4310302734375}, {2157000000.0, -3.421875}, {2158531250.0, -3.4146728515625}, {2160062500.0, -3.405517578125}, {2161593750.0, -3.3973388671875}, {2163125000.0, -3.388671875}, {2164656250.0, -3.3829345703125}, {2166187500.0, -3.3770751953125}, {2167718750.0, -3.372802734375}, {2169250000.0, -3.369873046875}, {2170781250.0, -3.362060546875}, {2172312500.0, -3.3583984375}, {2173843750.0, -3.351806640625}, {2175375000.0, -3.3477783203125}, {2176906250.0, -3.346435546875}, {2178437500.0, -3.3426513671875}, {2179968750.0, -3.3370361328125}, {2181500000.0, -3.3370361328125}, {2183031250.0, -3.33544921875}, {2184562500.0, -3.33349609375}, {2186093750.0, -3.33203125}, {2187625000.0, -3.3306884765625}, {2189156250.0, -3.3280029296875}, {2190687500.0, -3.3267822265625}, {2192218750.0, -3.3275146484375}, {2193750000.0, -3.32861328125}, {2195281250.0, -3.3291015625}, {2196812500.0, -3.3282470703125}, {2198343750.0, -3.3250732421875}, {2199875000.0, -3.319580078125}, {2201406250.0, -3.3212890625}, {2202937500.0, -3.3187255859375}, {2204468750.0, -3.3173828125}, {2206000000.0, -3.3154296875}, {2207531250.0, -3.3165283203125}, {2209062500.0, -3.3106689453125}, {2210593750.0, -3.3114013671875}, {2212125000.0, -3.3067626953125}, {2213656250.0, -3.307373046875}, {2215187500.0, -3.298828125}, {2216718750.0, -3.3006591796875}, {2218250000.0, -3.2982177734375}, {2219781250.0, -3.292236328125}, {2221312500.0, -3.29296875}, {2222843750.0, -3.2880859375}, {2224375000.0, -3.283935546875}, {2225906250.0, -3.284912109375}, {2227437500.0, -3.2813720703125}, {2228968750.0, -3.2757568359375}, {2230500000.0, -3.2767333984375}, {2232031250.0, -3.2691650390625}, {2233562500.0, -3.270751953125}, {2235093750.0, -3.265380859375}, {2236625000.0, -3.262451171875}, {2238156250.0, -3.2603759765625}, {2239687500.0, -3.2518310546875}, {2241218750.0, -3.2508544921875}, {2242750000.0, -3.248779296875}, {2244281250.0, -3.2388916015625}, {2245812500.0, -3.2393798828125}, {2247343750.0, -3.22998046875}, {2248875000.0, -3.228271484375}, {2250406250.0, -3.2205810546875}, {2251937500.0, -3.2132568359375}, {2253468750.0, -3.210205078125}, {2255000000.0, -3.2032470703125}, {2256531250.0, -3.19482421875}, {2258062500.0, -3.18798828125}, {2259593750.0, -3.183349609375}, {2261125000.0, -3.1776123046875}, {2262656250.0, -3.1693115234375}, {2264187500.0, -3.1639404296875}, {2265718750.0, -3.1580810546875}, {2267250000.0, -3.145263671875}, {2268781250.0, -3.1385498046875}, {2270312500.0, -3.1365966796875}, {2271843750.0, -3.128662109375}, {2273375000.0, -3.127197265625}, {2274906250.0, -3.1209716796875}, {2276437500.0, -3.1163330078125}, {2277968750.0, -3.11572265625}, {2279500000.0, -3.107666015625}, {2281031250.0, -3.1060791015625}, {2282562500.0, -3.0980224609375}, {2284093750.0, -3.1026611328125}, {2285625000.0, -3.097900390625}, {2287156250.0, -3.099853515625}, {2288687500.0, -3.09814453125}, {2290218750.0, -3.0960693359375}, {2291750000.0, -3.0953369140625}, {2293281250.0, -3.095703125}, {2294812500.0, -3.0968017578125}, {2296343750.0, -3.0947265625}, {2297875000.0, -3.0914306640625}, {2299406250.0, -3.0926513671875}, {2300937500.0, -3.0938720703125}, {2302468750.0, -3.097900390625}, {2304000000.0, -3.0931396484375}, {2305531250.0, -3.0946044921875}, {2307062500.0, -3.09375}, {2308593750.0, -3.097412109375}, {2310125000.0, -3.0943603515625}, {2311656250.0, -3.1019287109375}, {2313187500.0, -3.0994873046875}, {2314718750.0, -3.1031494140625}, {2316250000.0, -3.1009521484375}, {2317781250.0, -3.1031494140625}, {2319312500.0, -3.1064453125}, {2320843750.0, -3.1068115234375}, {2322375000.0, -3.1107177734375}, {2323906250.0, -3.109130859375}, {2325437500.0, -3.112060546875}, {2326968750.0, -3.112060546875}, {2328500000.0, -3.1124267578125}, {2330031250.0, -3.115234375}, {2331562500.0, -3.110107421875}, {2333093750.0, -3.113037109375}, {2334625000.0, -3.1173095703125}, {2336156250.0, -3.1192626953125}, {2337687500.0, -3.11572265625}, {2339218750.0, -3.1165771484375}, {2340750000.0, -3.1160888671875}, {2342281250.0, -3.11181640625}, {2343812500.0, -3.1114501953125}, {2345343750.0, -3.11083984375}, {2346875000.0, -3.103759765625}, {2348406250.0, -3.099853515625}, {2349937500.0, -3.0989990234375}, {2351468750.0, -3.0914306640625}, {2353000000.0, -3.0875244140625}, {2354531250.0, -3.0814208984375}, {2356062500.0, -3.073486328125}, {2357593750.0, -3.0693359375}, {2359125000.0, -3.059814453125}, {2360656250.0, -3.05419921875}, {2362187500.0, -3.0496826171875}, {2363718750.0, -3.042724609375}, {2365250000.0, -3.0343017578125}, {2366781250.0, -3.0245361328125}, {2368312500.0, -3.0179443359375}, {2369843750.0, -3.0126953125}, {2371375000.0, -3.005615234375}, {2372906250.0, -3.000732421875}, {2374437500.0, -2.9925537109375}, {2375968750.0, -2.9842529296875}, {2377500000.0, -2.981689453125}, {2379031250.0, -2.9752197265625}, {2380562500.0, -2.96875}, {2382093750.0, -2.9677734375}, {2383625000.0, -2.9610595703125}, {2385156250.0, -2.9559326171875}, {2386687500.0, -2.9537353515625}, {2388218750.0, -2.9473876953125}, {2389750000.0, -2.94677734375}, {2391281250.0, -2.94482421875}, {2392812500.0, -2.9434814453125}, {2394343750.0, -2.942626953125}, {2395875000.0, -2.9398193359375}, {2397406250.0, -2.93994140625}, {2398937500.0, -2.9383544921875}, {2400468750.0, -2.9383544921875}, {2402000000.0, -2.934814453125}, {2403531250.0, -2.933349609375}, {2405062500.0, -2.9345703125}, {2406593750.0, -2.9326171875}, {2408125000.0, -2.93310546875}, {2409656250.0, -2.9324951171875}, {2411187500.0, -2.933349609375}, {2412718750.0, -2.930419921875}, {2414250000.0, -2.928955078125}, {2415781250.0, -2.934814453125}, {2417312500.0, -2.93310546875}, {2418843750.0, -2.9351806640625}, {2420375000.0, -2.93994140625}, {2421906250.0, -2.935546875}, {2423437500.0, -2.9403076171875}, {2424968750.0, -2.9415283203125}, {2426500000.0, -2.9486083984375}, {2428031250.0, -2.9442138671875}, {2429562500.0, -2.94775390625}, {2431093750.0, -2.95263671875}, {2432625000.0, -2.9527587890625}, {2434156250.0, -2.9598388671875}, {2435687500.0, -2.963134765625}, {2437218750.0, -2.9625244140625}, {2438750000.0, -2.965576171875}, {2440281250.0, -2.9666748046875}, {2441812500.0, -2.9693603515625}, {2443343750.0, -2.9722900390625}, {2444875000.0, -2.9708251953125}, {2446406250.0, -2.969482421875}, {2447937500.0, -2.9716796875}, {2449468750.0, -2.9696044921875}, {2451000000.0, -2.9688720703125}, {2452531250.0, -2.9713134765625}, {2454062500.0, -2.968017578125}, {2455593750.0, -2.964111328125}, {2457125000.0, -2.963134765625}, {2458656250.0, -2.95751953125}, {2460187500.0, -2.95556640625}, {2461718750.0, -2.9476318359375}, {2463250000.0, -2.943603515625}, {2464781250.0, -2.9373779296875}, {2466312500.0, -2.9344482421875}, {2467843750.0, -2.924072265625}, {2469375000.0, -2.9202880859375}, {2470906250.0, -2.9102783203125}, {2472437500.0, -2.9044189453125}, {2473968750.0, -2.9005126953125}, {2475500000.0, -2.895263671875}, {2477031250.0, -2.8848876953125}, {2478562500.0, -2.878662109375}, {2480093750.0, -2.873779296875}, {2481625000.0, -2.866455078125}, {2483156250.0, -2.8590087890625}, {2484687500.0, -2.8555908203125}, {2486218750.0, -2.85400390625}, {2487750000.0, -2.8486328125}, {2489281250.0, -2.84375}, {2490812500.0, -2.841796875}, {2492343750.0, -2.8387451171875}, {2493875000.0, -2.837158203125}, {2495406250.0, -2.8336181640625}, {2496937500.0, -2.8331298828125}, {2498468750.0, -2.8311767578125}, {2500000000.0, -2.8309326171875}], 3 "dup VISA session":refnum<visa-resource-name>="GPIB0::22::INSTR")   [LabVIEW 2018]
doc: "It is recommended that you hold off triggers before running this VI as the HP8753 tends to \"hang\" if data is read while measurements are being taken.\n\n This VI is used to collect and display data generated by the HP8753 Network Analyzer. The VI can display error-corrected data, error-corrected trace memory, fully formatted data and memory traces. For further information on these types of data see Processsing Chain figure in the HPIB programming note. When the data type is a formatted data, the instruments screen will change to reflect what is being displayed, eg. selecting \"formatted memory\" changes the display to \"MEMORY\".\n\n The data values shown depend upon the data type and the measurement format. If the data type is \"error-corrected data\" or \"error-corrected trace memory\" and/or the measurement format is \"Smith chart\" or \"polar\", the data values are real,imaginary pairs. Otherwise the data values are stimulus,response pairs. These pairs correspond to what is shown in the graphical display.\n\n Data can also be saved to a file with this VI. When saving a file, the stimulus is always shown. The real,imaginary components or the response value are also shown depending upon the data type and the measurement format. \n\n No units are shown on the VI front panel or in the data file. All units are basic units of Hz, dB, seconds, ohms, etc. The \"saved data comments\" control should be used for any special information such as the measurement format, averaging and smoothing information, etc.\n\n Whether or not data is saved and whether the output is in real,imaginary pairs or stimulus,response parirs affects the speed of this VI. When data is saved to a file and/or when data is in stimulus,response pairs, requires the reading of the stimulus values which slows the VI down. The fastest reads are done when the data type is \"error-corrected data\" or \"error-corrected trace memory\" and/or the measurement format is \"Smith chart\" or \"polar\" and data is not being saved to a file.\n\n This VI sets the format, ie. linear or logarithmic, depending upon the sweep type. \n\nFYI - Originally this VI was written without considering the stimulus values. In most case this would be fine for display purposes as the point number could be used for the X value as most sweeps are evenly spaced. This is not the case with frequency list sweeps which can have big gaps in the sweep. For this reason the stimulus value is read (at least in the cases explained above) to make the LabVIEW display match what is display on the instrument's display."
uses:
  <vilib>/Instr/_visa.llb/VISA GPIB Control REN Mode.ctl
  8720/Agilent 87XX Series/Agilent 87XX Series.lvlib
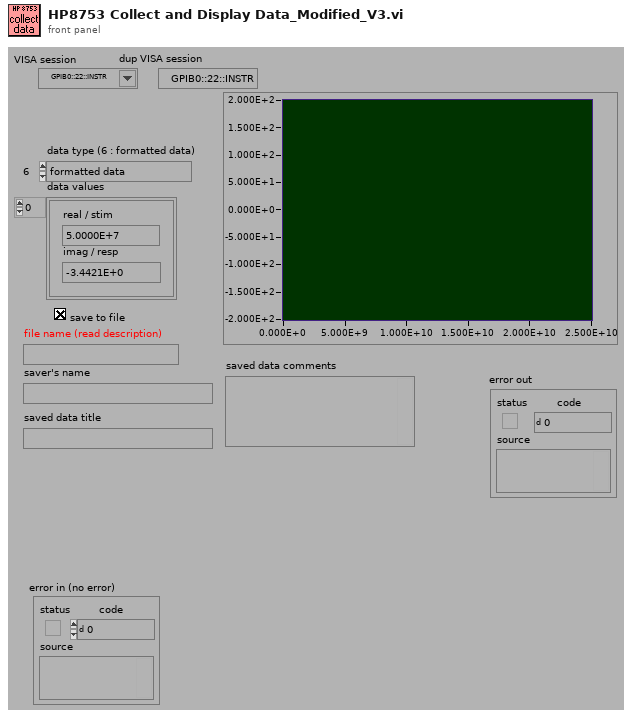
[diagram p1: front panel]
types:
  T1 = typedef "VISA GPIB Control REN Mode.ctl" = u16
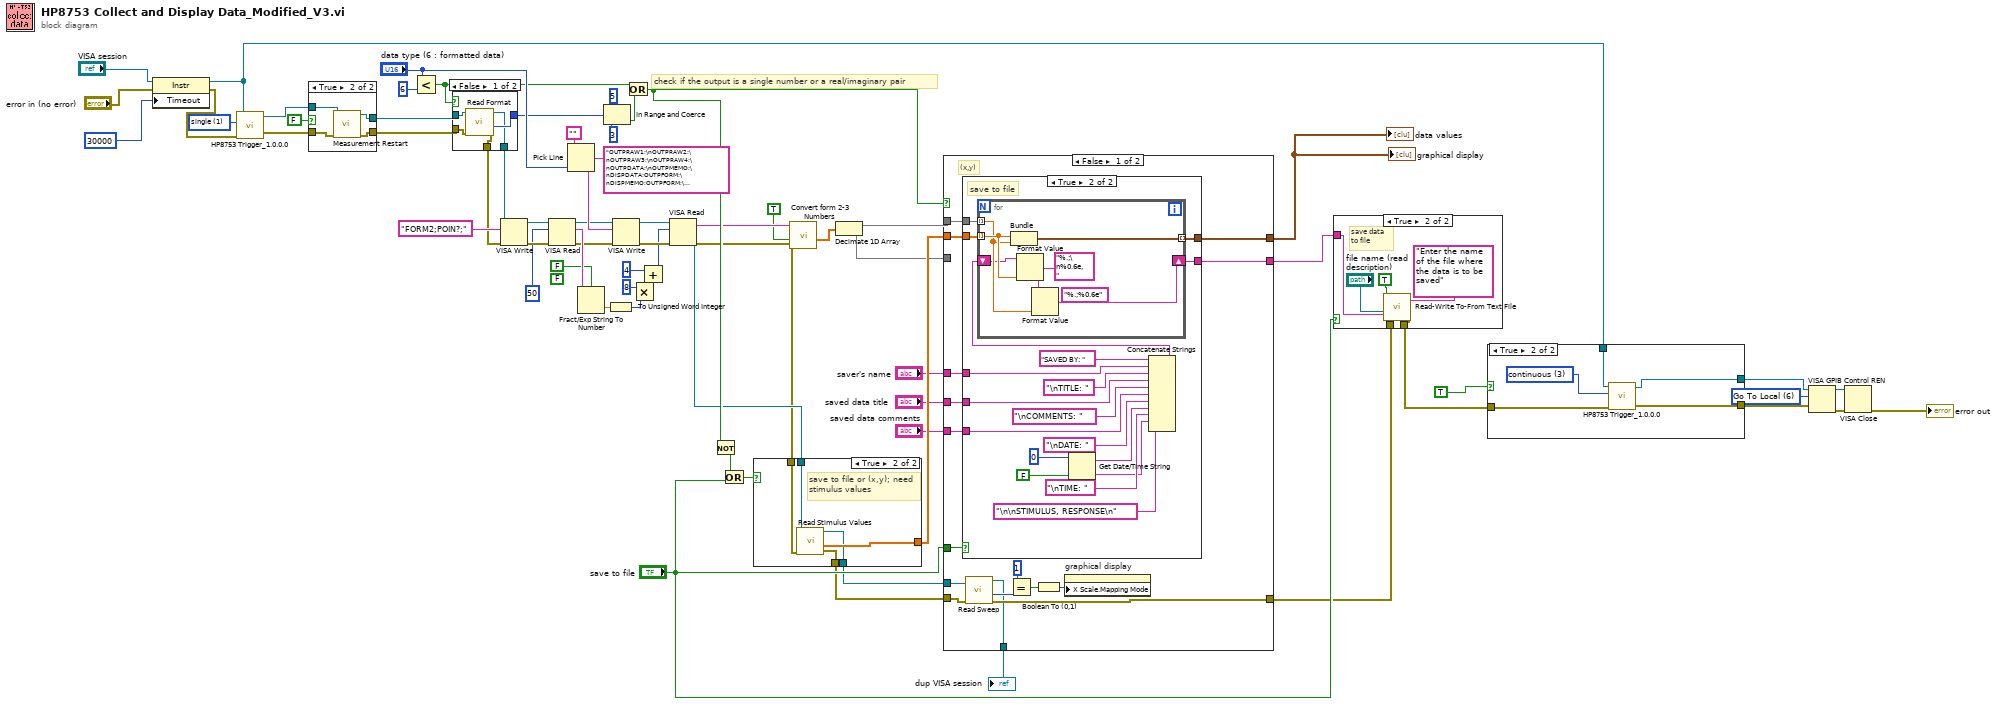
[diagram p0: block diagram]
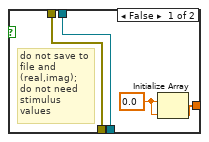
[diagram p4: hidden frame]
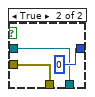
[diagram p5: hidden frame]
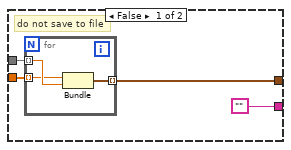
[diagram p7: hidden frame]
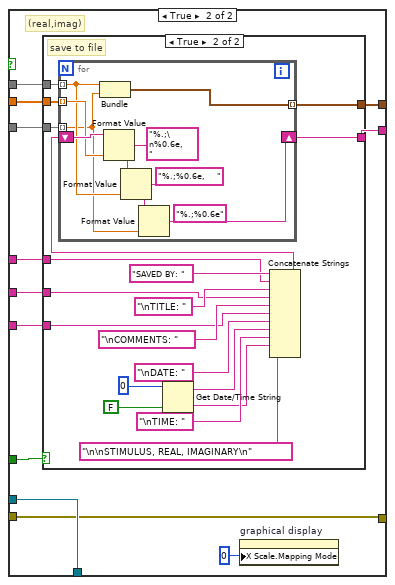
[diagram p8: hidden frame]
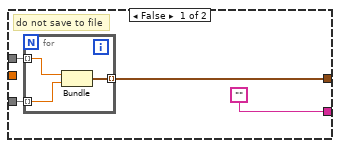
[diagram p9: hidden frame]
diagram:
  w7 = T1 6 items=["Deassert REN", "Assert REN", "Go To Local; Deassert REN ", "Assert REN; Address Device", "Local Lockout (Addressed Devices)", "Local Lockout (This Device)", "Go To Local"] ("Mode")
  w15 = u16 1 items=["hold", "single", "number of groups", "continuous"] ("trigger (1 : single)")
  (unwired) FALSE ("use system decimal point (T)")
  # "check if the output is a single number or a real/imaginary pair"
  n1 = property class="Instr"(reference="VISA session", error in="error in (no error)", "Timeout"=u32 30000 ("General Settings:Timeout Value")) -> (reference out=w8:refnum<visa-resource-name>, error out=w12:errorcluster)
  n2 = call "HP8753 Trigger_1.0.0.0.vi"("error in (no error)"=w12, "trigger (1 : single)"=w15, "VISA session"=w8) -> ("error out"=w16:errorcluster, "dup VISA session"=w19:refnum<visa-resource-name>)  [unwired: 2 in]
  n3 = case shown="True" FALSE {
    tunnel: w19 -> [w71 w75]
    tunnel: [w71 w74] -> w18
    tunnel: [w70 w73] -> w17
    tunnel: w16 -> [w70 w72]
    frame False {
    }
    frame True {
      n4 = call "Measurement Restart.vi"("error in (no error)"=w72, "VISA resource name"=w75) -> ("error out"=w73:errorcluster, "VISA resource name out"=w74:refnum<visa-resource-name>)  [unwired: 8 in]
    }
  }
  n5 = Less?(x="data type (6 : formatted data)", y=u16 6) -> (x < y?=w51:bool)
  n6 = case shown="False" w51 {
    tunnel: [w80 0] -> w50
    tunnel: w18 -> [w76 w81]
    tunnel: w17 -> [w79 w82]
    tunnel: [w78 w81] -> w42
    tunnel: [w77 w82] -> w41
    frame False {
      n7 = call "Read Format.vi"("error in (no error)"=w79, "VISA resource name"=w76) -> ("error out"=w77:errorcluster, "format"=w80:i32, "VISA resource name out"=w78:refnum<visa-resource-name>)  [unwired: 7 in]
    }
    frame True {
    }
  }
  n8 = VISA Write(VISA resource name=w42, write buffer="FORM2;POIN?;", error in (no error)=w41) -> (VISA resource name out=w23:refnum<visa-resource-name>, error out=w66:errorcluster)  [unwired: 1 out]
  n9 = VISA Read(VISA resource name=w23, byte count=u32 50, error in (no error)=w66) -> (VISA resource name out=w48:refnum<visa-resource-name>, read buffer=w64:string, error out=w63:errorcluster)  [unwired: 1 out]
  n10 = Pick Line(string ("")="", multi-line string="OUTPRAW1;\nOUTPRAW2;\nOUTPRAW3;\nOUTPRAW4;\nOUTPDATA;\nOUTPMEMO;\nDISPDATA;OUTPFORM;\nDISPMEMO;OUTPFORM;\nDISPDDM;OUTPFORM;\nDISPDMM;OUTPFORM;", line index="data type (6 : formatted data)") -> (output string=w53:string)
  n11 = Fract/Exp String To Number(use system decimal point (T)=FALSE, string=w64) -> (number=w65:dbl)  [unwired: 2 in, 1 out]
  n12 = In Range and Coerce(upper limit=5, x=w50, lower limit=3) -> (In Range?=w67:bool)  [unwired: 1 out]
  n13 = To Unsigned Word Integer(number=w65) -> (unsigned 16bit integer=w33:u16)
  n14 = VISA Write(VISA resource name=w48, write buffer=w53, error in (no error)=w63) -> (VISA resource name out=w22:refnum<visa-resource-name>, error out=w62:errorcluster)  [unwired: 1 out]
  n15 = Or(x=w51, y=w67) -> (x .or. y?=w44:bool)
  n16 = Multiply(x=u16 8, y=w33) -> (x*y=w60:u16)
  n17 = Add(x=u16 4, y=w60) -> (x+y=w24:u16)
  n18 = VISA Read(VISA resource name=w22, byte count=w24, error in (no error)=w62) -> (VISA resource name out=w40:refnum<visa-resource-name>, read buffer=w27:string, error out=w28:errorcluster)  [unwired: 1 out]
  n19 = Not(x=w44) -> (.not. x?=w45:bool)
  n20 = Or(x=w45, y="save to file") -> (x .or. y?=w47:bool)
  n21 = call "Convert form 2-3 Numbers.vi"("error in (no error)"=w28, "data format"=TRUE, "input string"=w27) -> ("error out"=w29:errorcluster, "converted numbers"=w32:dbl[])  [unwired: 7 in]
  n22 = case shown="True" w47 {
    tunnel: w29 -> [w85 w91]
    tunnel: w40 -> [w84 w90]
    tunnel: [w87 w92] -> w43
    tunnel: [w85 w89] -> w35
    tunnel: [w84 w88] -> w36
    frame False {
      w86 = 0.0
      # "do not save to file and (real,imag);\ndo not need stimulus values"
      n23 = Initialize Array(w86, w86) -> (w87:dbl[])
    }
    frame True {
      # "save to file or (x,y); need\nstimulus values"
      n24 = call "Read Stimulus Values.vi"("error in (no error)"=w91, "VISA resource name"=w90) -> ("error out"=w89:errorcluster, "stimulus list"=w92:dbl[], "VISA resource name out"=w88:refnum<visa-resource-name>)  [unwired: 7 in]
    }
  }
  n25 = Decimate 1D Array(w32) -> (w31:dbl[], w30:dbl[])
  n26 = case shown="False" w44 {
    tunnel: w30 -> [_ w149]
    tunnel: w31 -> [w107 w152]
    tunnel: w43 -> [w106 w151]
    tunnel: [w105 w150] -> w49
    tunnel: "save to file" -> [w108 w153]
    tunnel: [w104 w148] -> w58
    tunnel: "saver's name" -> [w103 w147]
    tunnel: "saved data title" -> [w102 w146]
    tunnel: "saved data comments" -> [w101 w145]
    tunnel: w35 -> [w100 w143]
    tunnel: w36 -> [w99 w144]
    tunnel: [w94 w143] -> w34
    tunnel: [w93 w144] -> w21
    frame False {
      # "(x,y)"
      n27 = case shown="True" w108 {
        tunnel: w107 -> [w112 w133]
        tunnel: w106 -> [w111 w132]
        tunnel: [w110 w121] -> w105
        tunnel: ["" w120] -> w104
        tunnel: w103 -> [_ w119]
        tunnel: w102 -> [_ w118]
        tunnel: w101 -> [_ w117]
        frame False {
          # "do not save to file"
          n28 = for {
            tunnel: w112 -> [w114] mode=indexing
            tunnel: [w115] -> w110 mode=indexing
            tunnel: w111 -> [w113] mode=indexing
            n29 = Bundle(w113, w114) -> (w115:cluster{dbl, dbl})  [unwired: 1 in]
          }
        }
        frame True {
          # "save to file"
          n30 = Get Date/Time String(date format (0)=0, want seconds? (F)=FALSE) -> (date string=w125:string, time string=w123:string)  [unwired: 1 in]
          n31 = Concatenate Strings("SAVED BY: ", w119, "\nTITLE: ", w118, "\nCOMMENTS: ", w117, "\nDATE: ", w125, "\nTIME: ", w123, "\n\nSTIMULUS, RESPONSE\n") -> (w122:string)
          n32 = for {
            tunnel: w133 -> [w136] mode=indexing
            tunnel: [w141] -> w121 mode=indexing
            tunnel: w132 -> [w137] mode=indexing
            shift-right: [w134] -> w120
            shift-left: w122 -> [w135]
            n33 = Bundle(w137, w136) -> (w141:cluster{dbl, dbl})  [unwired: 1 in]
            n34 = Format Value(string ("")=w135, format string="%.;\n%0.6e,  ", value (0)=w137) -> (output string=w138:string)
            n35 = Format Value(string ("")=w138, format string="%.;%0.6e", value (0)=w136) -> (output string=w134:string)
          }
        }
      }
      n36 = call "Read Sweep.vi"("error in (no error)"=w100, "VISA resource name"=w99) -> ("error out"=w94:errorcluster, "sweep type"=w98:i32, "VISA resource name out"=w93:refnum<visa-resource-name>)  [unwired: 7 in]
      n37 = Equal?(x=1, y=w98) -> (x = y?=w96:bool)
      n38 = Boolean To (0,1)(Boolean=w96) -> (0, 1=w95:i16)
      n39 = property on="graphical display" class="XYGraph (strict)"("X Scale.Mapping Mode"=w95) -> ()  [unwired: 2 in, 2 out]
    }
    frame True {
      # "(real,imag)"
      n40 = case shown="True" w153 {
        tunnel: w152 -> [w157 w179]
        tunnel: w151 -> [_ w166]
        tunnel: [w156 w165] -> w150
        tunnel: ["" w168] -> w148
        tunnel: w149 -> [w154 w167]
        tunnel: w147 -> [_ w164]
        tunnel: w146 -> [_ w163]
        tunnel: w145 -> [_ w162]
        frame False {
          # "do not save to file"
          n41 = for {
            tunnel: w157 -> [w159] mode=indexing
            tunnel: [w160] -> w156 mode=indexing
            tunnel: w154 -> [w158] mode=indexing
            n42 = Bundle(w159, w158) -> (w160:cluster{dbl, dbl})  [unwired: 1 in]
          }
        }
        frame True {
          # "save to file"
          n43 = Get Date/Time String(date format (0)=0, want seconds? (F)=FALSE) -> (date string=w172:string, time string=w170:string)  [unwired: 1 in]
          n44 = Concatenate Strings("SAVED BY: ", w164, "\nTITLE: ", w163, "\nCOMMENTS: ", w162, "\nDATE: ", w172, "\nTIME: ", w170, "\n\nSTIMULUS, REAL, IMAGINARY\n") -> (w169:string)
          n45 = for {
            tunnel: w179 -> [w181] mode=indexing
            tunnel: [w190] -> w165 mode=indexing
            shift-right: [w182] -> w168
            shift-left: w169 -> [w186]
            tunnel: w167 -> [w180] mode=indexing
            tunnel: w166 -> [w185] mode=indexing
            n46 = Bundle(w181, w180) -> (w190:cluster{dbl, dbl})  [unwired: 1 in]
            n47 = Format Value(string ("")=w186, format string="%.;\n%0.6e,    ", value (0)=w185) -> (output string=w187:string)
            n48 = Format Value(string ("")=w187, format string="%.;%0.6e,    ", value (0)=w181) -> (output string=w183:string)
            n49 = Format Value(string ("")=w183, format string="%.;%0.6e", value (0)=w180) -> (output string=w182:string)
          }
        }
      }
      n50 = property on="graphical display" class="XYGraph (strict)"("X Scale.Mapping Mode"=u8 0) -> ()  [unwired: 2 in, 2 out]
    }
  }
  "data values" <- w49
  "graphical display" <- w49
  "dup VISA session" <- w21
  n51 = case shown="True" "save to file" {
    tunnel: w58 -> [_ w194]
    tunnel: w34 -> [w191 w193]
    tunnel: [w191 w192] -> w9
    frame False {
    }
    frame True {
      # "save data to file"
      n52 = call "Read-Write To-From Text File.vi"("string to be written"=w194, "dialog box prompt"="Enter the name of the file where the data is to be saved", "error in (no error)"=w193, "file name (read description)"="file name (read description)", "read/write (f:read)"=TRUE) -> ("error out"=w192:errorcluster)  [unwired: 5 in, 1 out]
    }
  }
  n53 = case shown="True" TRUE {
    tunnel: w9 -> [w199 w204]
    tunnel: w8 -> [w198 w202]
    tunnel: [w199 w201] -> w3
    tunnel: [w198 w200] -> w2
    frame False {
    }
    frame True {
      w203 = u16 3 items=["hold", "single", "number of groups", "continuous"] ("trigger (1 : single)")
      n54 = call "HP8753 Trigger_1.0.0.0.vi"("error in (no error)"=w204, "trigger (1 : single)"=w203, "VISA session"=w202) -> ("error out"=w201:errorcluster, "dup VISA session"=w200:refnum<visa-resource-name>)  [unwired: 2 in]
    }
  }
  n55 = VISA GPIB Control REN(8:w3, 10:w7, 11:w2) -> (0:w5:errorcluster, 3:w6:refnum<visa-resource-name>)
  n56 = VISA Close(VISA resource name=w6, error in (no error)=w5) -> (error out=→"error out":errorcluster)
